vi "DetectorTest_MainV3.vi"() -> ()   [LabVIEW 2012]
uses:
  <vilib>/Utility/file.llb/Read From Spreadsheet File (DBL).vi
  <vilib>/Analysis/NI_AALBase.lvlib
panel:
  in  "TL4000 In":refnum<visa-resource-name> caption="resource name"
  out "Laser Counter":i32
  out "TL4000 Out":refnum<visa-resource-name> caption="instrument handle out"
  out "Calibration":cluster{"Y":dbl[], "Y":dbl[]}[](graph)
  out "Output Power (mW)":dbl
  in  "Load Calibration File":path
  out "Counter":i32
  out "NameList":string[](array[string])=["Diode_Open_3000", "Diode_Open_2000", "Diode_Open_1000", "Diode_Open_500", "Diode_Open_300", "Diode_Open_200", "Diode_Open_100", "Diode_Open_70", "Diode_Open_50", "Diode_Open_20", "Diode_Open_5_500", "Diode_Open_5_300", "Diode_Open_5_200", "Diode_Open_5_100", "Diode_Open_5_70", "Diode_Open_5_50", "Diode_Open_5_20", "Diode_Full_500", "Diode_Full_300", "Diode_Full_200", "Diode_Full_100", "Diode_Full_70", "Diode_Full_50", "Diode_Full_20", "Diode_Open_100_A", "Diode_Open_200_A", "QE_pad"]
  in  "Wafer Info Flash 2":T1={"Cell Name"="5500_130_05", "Package"="", "Coating"="", "LRC?"=enum."J2", "Comment"=""}
  in  "Parameters Flash 2":T2 {"Voc" format="%#_4g"; "Isc" format="%#_4g"; "FF" format="%#_4g"; "Imax" format="%#_4g"; "Vmax" format="%#_4g"; "Pmax" format="%#_4g"; "Itest" format="%#_4g"}
  in  "Wafer Info Flash":T1={"Cell Name"="Diode_Open_5_100", "Package"="", "Coating"="", "LRC?"=enum."J2", "Comment"=""}
  in  "Parameters Flash":T2={"Voc"=0.0, "Isc"=0.0, "FF"=0.0, "Vtest"=0.0, "Imax"=0.0, "Vmax"=0.0, "Pmax"=0.0, "Itest"=0.0, "Efficiency"=0.0, "Incident Power"=0.0, "Power Density (W/cm^2)"=0.0, "Cell Area (cm²)"=12801.99006, "Number of AM1.5D Suns"=0.0, "Input Current (mA)"=0.0, "Equivalent 1 sun Jsc"=0.0} {"Voc" format="%#_4g"; "Isc" format="%#_4g"; "FF" format="%#_4g"; "Imax" format="%#_4g"; "Vmax" format="%#_4g"; "Pmax" format="%#_4g"; "Itest" format="%#_4g"}
  out "RawData file":path=path "C:/Users/Flash/Desktop/Data/Detector test data/A-3348-2-A_Diode_Open_5_100_20171205171726.csv"
  out "Fine Cell Clusters":T3(array[cluster])=[{"Cell Name"="Diode_Open_5_100", "X-coord"=56060.0, "Y-coord"=24330.0, "Area"=12801.99006, "Grid Shadowing"=0.0, "Xdim"=50.0, "Ydim"=50.0, "Mesa Area"=7853.981634}, {"Cell Name"="Diode_Open_5_100", "X-coord"=56060.0, "Y-coord"=14330.0, "Area"=12801.99006, "Grid Shadowing"=0.0, "Xdim"=50.0, "Ydim"=50.0, "Mesa Area"=7853.981634}, {"Cell Name"="Diode_Open_5_100", "X-coord"=-3940.0, "Y-coord"=4330.0, "Area"=12801.99006, "Grid Shadowing"=0.0, "Xdim"=50.0, "Ydim"=50.0, "Mesa Area"=7853.981634}, {"Cell Name"="Diode_Open_5_100", "X-coord"=-9540.0, "Y-coord"=10700.0, "Area"=12801.99006, "Grid Shadowing"=0.0, "Xdim"=50.0, "Ydim"=50.0, "Mesa Area"=7853.981634}, {"Cell Name"="Diode_Open_5_100", "X-coord"=46060.0, "Y-coord"=4330.0, "Area"=12801.99006, "Grid Shadowing"=0.0, "Xdim"=50.0, "Ydim"=50.0, "Mesa Area"=7853.981634}, {"Cell Name"="Diode_Open_5_100", "X-coord"=6060.0, "Y-coord"=-5670.0, "Area"=12801.99006, "Grid Shadowing"=0.0, "Xdim"=50.0, "Ydim"=50.0, "Mesa Area"=7853.981634}, {"Cell Name"="Diode_Open_5_100", "X-coord"=460.0, "Y-coord"=700.0, "Area"=12801.99006, "Grid Shadowing"=0.0, "Xdim"=50.0, "Ydim"=50.0, "Mesa Area"=7853.981634}, {"Cell Name"="Diode_Open_5_100", "X-coord"=16060.0, "Y-coord"=-5670.0, "Area"=12801.99006, "Grid Shadowing"=0.0, "Xdim"=50.0, "Ydim"=50.0, "Mesa Area"=7853.981634}, {"Cell Name"="Diode_Open_5_100", "X-coord"=26060.0, "Y-coord"=-5670.0, "Area"=12801.99006, "Grid Shadowing"=0.0, "Xdim"=50.0, "Ydim"=50.0, "Mesa Area"=7853.981634}, {"Cell Name"="Diode_Open_5_100", "X-coord"=30460.0, "Y-coord"=700.0, "Area"=12801.99006, "Grid Shadowing"=0.0, "Xdim"=50.0, "Ydim"=50.0, "Mesa Area"=7853.981634}]
  out "Selected Data":cluster{dbl[], dbl[]}={[nan, nan, nan, nan, nan, nan, nan, nan, nan, nan, nan, nan, nan, nan, nan, nan, nan, nan, nan, nan, nan, nan, nan, nan, nan, nan, nan, nan, nan, nan, nan, nan, nan, nan, nan, nan, nan, nan, nan, nan, nan, nan, nan, nan, nan, nan, nan, nan, nan, nan, nan, nan, nan, nan, nan, nan, nan, nan, nan, nan, nan, nan, nan, nan, nan, nan, nan, nan, nan, nan, nan, nan, nan, nan, nan, nan, nan, nan, nan, nan, nan, nan, nan, nan, nan, nan, nan, nan, nan, nan, nan, nan, nan, nan, nan, nan, nan, nan, nan, nan, nan, nan, nan, nan], [nan, nan, nan, nan, nan, nan, nan, nan, nan, nan, nan, nan, nan, nan, nan, nan, nan, nan, nan, nan, nan, nan, nan, nan, nan, nan, nan, nan, nan, nan, nan, nan, nan, nan, nan, nan, nan, nan, nan, nan, nan, nan, nan, nan, nan, nan, nan, nan, nan, nan, nan, nan, nan, nan, nan, nan, nan, nan, nan, nan, nan, nan, nan, nan, nan, nan, nan, nan, nan, nan, nan, nan, nan, nan, nan, nan, nan, nan, nan, nan, nan, nan, nan, nan, nan, nan, nan, nan, nan, nan, nan, nan, nan, nan, nan, nan, nan, nan, nan, nan, nan, nan, nan, nan]}
  in  "Test Results 2":T4
  in  "Session Info 2":T5={"V set"=-1.0, "I compliance"=0.001, "J set"=0.01, "I set"=0.0, "V compliance"=1.0, "Laser Power (mW)"=0.0, "TestID"=0, "Session Time"=timestamp(0 s since 1904-01-01), "Operator"="Radek"} {"V compliance" format="%#_6f"; "I compliance" format="%#_6e"}
  in  "Die Info 2":T6={"Device Name"="", "ActiveArea_um2"=3848.451, "MesaArea_um2"=3848.451, "x"=0.0, "y"=0.0}
  in  "Wafer Info 2":T7
  in  "Test Results":T4={"I meas"=-8.21153e-09, "V meas"=0.229564, "Time"=timestamp(3595368212.7604895 s since 1904-01-01)}
  in  "Session Info":T5={"V set"=-1.0, "I compliance"=0.001, "J set"=0.01, "I set"=1.5393804e-06, "V compliance"=1.0, "Laser Power (mW)"=0.0, "TestID"=289, "Session Time"=timestamp(3595367846.336531 s since 1904-01-01), "Operator"="pkawula"} {"V compliance" format="%#_6f"; "I compliance" format="%#_6e"}
  in  "Die Info":T6={"Device Name"="Diode_Open_5_100", "ActiveArea_um2"=12801.99006, "MesaArea_um2"=7853.981634, "x"=6060.0, "y"=44330.0}
  in  "Wafer Info":T7={"Wafer Name"="A-3348-2-A", "Scribe"="BG531-103", "Mask"="SL066", "Lot"="SJC_ENG_342_4"}
  in  "Name Array":string[](array[string])=["Wafer name", "Scribe", "Mask", "Lot", "Device name", "Active Area", "Mesa Area", "x", "y", "Imeas", "Vmeas", "Time", "Vset", "Icomp", "Jset", "Iset", "Vcomp", "Laser Power", "TestID", "SessionTime", "Operator", "Selected"]
  in  "TestID file":path=path "C:/Users/Flash/Desktop/LabVIEW/Detector IV/rawtest_log.csv"
  in  "update wafer":bool
  in  "Lot":string="SJC_ENG_342_4"
  in  "Laser Current (mA)":dbl
  in  "Device Name":string="Diode_Open_5_100"
  in  "Scribe":string="BG531-105"
  in  "MesaArea_um2":dbl=7853.981634
  out "Status":string="idle"
  out "error out":errorcluster
  in  "error in (no error)":errorcluster
  out "Manaul Plot 1":cluster{"V manual":dbl[], dbl[]}[](array[cluster])=[{"V manual"=[-1.5, -1.45128, -1.40256, -1.35385, -1.30513, -1.25641, -1.20769, -1.15897, -1.11026, -1.06154, -1.01282, -0.964103, -0.915385, -0.866667, -0.817949, -0.769231, -0.720513, -0.671795, -0.623077, -0.574359, -0.525641, -0.476923, -0.428205, -0.379487, -0.330769, -0.282051, -0.233333, -0.184615, -0.135897, -0.0871795, -0.0384615, 0.0102564, 0.0589744, 0.107692, 0.15641, 0.205128, 0.253846, 0.302564, 0.351282, 0.4], [0.000371182, 0.000368087, 0.000365666, 0.000361585, 0.000358777, 0.000355415, 0.000352273, 0.00034839, 0.000345122, 0.00034151, 0.00033751, 0.000332836, 0.000329855, 0.000326461, 0.000322528, 0.000317656, 0.000313266, 0.000310053, 0.000304697, 0.000300113, 0.00029575, 0.000290713, 0.000285749, 0.00028048, 0.000275303, 0.000269023, 0.000263057, 0.000256756, 0.000250067, 0.000242646, 0.000235352, 0.000226249, 0.000216807, 0.000205541, 0.000192231, 0.000174354, 0.000146988, 9.49448e-05, 1.32493e-05, 0.000227531]}, {"V manual"=[-1.0, nan, nan, nan, nan, nan, nan, nan, nan, nan, nan, nan, nan, nan, nan, nan, nan, nan, nan, nan, nan, nan, nan, nan, nan, nan, nan, nan, nan, nan, nan, nan, nan, nan, nan, nan, nan, nan, nan, nan], [0.0003364616, nan, nan, nan, nan, nan, nan, nan, nan, nan, nan, nan, nan, nan, nan, nan, nan, nan, nan, nan, nan, nan, nan, nan, nan, nan, nan, nan, nan, nan, nan, nan, nan, nan, nan, nan, nan, nan, nan, nan]}, {"V manual"=[0.369974, nan, nan, nan, nan, nan, nan, nan, nan, nan, nan, nan, nan, nan, nan, nan, nan, nan, nan, nan, nan, nan, nan, nan, nan, nan, nan, nan, nan, nan, nan, nan, nan, nan, nan, nan, nan, nan, nan, nan], [8.183848863e-05, nan, nan, nan, nan, nan, nan, nan, nan, nan, nan, nan, nan, nan, nan, nan, nan, nan, nan, nan, nan, nan, nan, nan, nan, nan, nan, nan, nan, nan, nan, nan, nan, nan, nan, nan, nan, nan, nan, nan]}]
  out "Manual Plot 0":cluster{"V manual":dbl[], "I manual":dbl[]}[](array[cluster])=[{"V manual"=[-1.5, -1.45128, -1.40256, -1.35385, -1.30513, -1.25641, -1.20769, -1.15897, -1.11026, -1.06154, -1.01282, -0.964103, -0.915385, -0.866667, -0.817949, -0.769231, -0.720513, -0.671795, -0.623077, -0.574359, -0.525641, -0.476923, -0.428205, -0.379487, -0.330769, -0.282051, -0.233333, -0.184615, -0.135897, -0.0871795, -0.0384615, 0.0102564, 0.0589744, 0.107692, 0.15641, 0.205128, 0.253846, 0.302564, 0.351282, 0.4], "I manual"=[-0.000371182, -0.000368087, -0.000365666, -0.000361585, -0.000358777, -0.000355415, -0.000352273, -0.00034839, -0.000345122, -0.00034151, -0.00033751, -0.000332836, -0.000329855, -0.000326461, -0.000322528, -0.000317656, -0.000313266, -0.000310053, -0.000304697, -0.000300113, -0.00029575, -0.000290713, -0.000285749, -0.00028048, -0.000275303, -0.000269023, -0.000263057, -0.000256756, -0.000250067, -0.000242646, -0.000235352, -0.000226249, -0.000216807, -0.000205541, -0.000192231, -0.000174354, -0.000146988, -9.49448e-05, 1.32493e-05, 0.000227531]}, {"V manual"=[-1.0, nan, nan, nan, nan, nan, nan, nan, nan, nan, nan, nan, nan, nan, nan, nan, nan, nan, nan, nan, nan, nan, nan, nan, nan, nan, nan, nan, nan, nan, nan, nan, nan, nan, nan, nan, nan, nan, nan, nan], "I manual"=[-0.0003364616, nan, nan, nan, nan, nan, nan, nan, nan, nan, nan, nan, nan, nan, nan, nan, nan, nan, nan, nan, nan, nan, nan, nan, nan, nan, nan, nan, nan, nan, nan, nan, nan, nan, nan, nan, nan, nan, nan, nan]}, {"V manual"=[0.369974, nan, nan, nan, nan, nan, nan, nan, nan, nan, nan, nan, nan, nan, nan, nan, nan, nan, nan, nan, nan, nan, nan, nan, nan, nan, nan, nan, nan, nan, nan, nan, nan, nan, nan, nan, nan, nan, nan, nan], "I manual"=[8.183848863e-05, nan, nan, nan, nan, nan, nan, nan, nan, nan, nan, nan, nan, nan, nan, nan, nan, nan, nan, nan, nan, nan, nan, nan, nan, nan, nan, nan, nan, nan, nan, nan, nan, nan, nan, nan, nan, nan, nan, nan]}]
  in  "Reset 1st die":bool
  in  "Sweep Settings":T8={"Channel"=enum."Channel A", "Vstart"=-2.0, "Vend"=0.5, "# of points"=30, "NPLC"=1.0, "I compliance"=0.001, "Delay ms"=500.0}
  in  "Reset xy":bool
  out "current y":i32
  out "current x":i32
  in  "sweep delay ms":dbl=500.0
  in  "I compliance":dbl=0.001
  in  "points":u16=40
  in  "V end":dbl=0.4
  in  "V start":dbl=-1.5
  in  "Repeat Vf":u32=1
  out "I set":dbl=7.853981633999999e-07
  in  "V compliance":dbl=1.0 format="%#_6f"
  in  "Vf delay ms":dbl=100.0
  in  "J set A/cm2":dbl=0.01
  in  "Repeat Id":u32=5
  in  "I compliance":dbl=0.001 format="%#_6e"
  in  "Id delay ms":dbl=500.0
  in  "V set":dbl=-1.0
  out "Vmeas Settings":T9={"Channel"=enum."Channel A", "Iset"=-1.0, "NPLC"=1.0, "V compliance"=0.001, "Repeat time"=3, "Delay ms"=500.0}
  out "Imeas Settings":T10={"Channel"=enum."Channel A", "Vset"=-1.0, "NPLC"=1.0, "I compliance"=0.001, "Repeat time"=3, "Delay ms"=500.0}
  out "Array of Cell Data Clusters":T11(array[cluster])=[{"Cell Name"="Diode_Open_5_100", "X-coord"=-13940.0, "Y-coord"=24330.0, "Area"=12801.99006, "Grid Shadowing"=0.0, "Ydim"=50.0, "Xdim"=50.0, "Meas Area"=7853.981634}, {"Cell Name"="Diode_Open_5_100", "X-coord"=-19540.0, "Y-coord"=30700.0, "Area"=12801.99006, "Grid Shadowing"=0.0, "Ydim"=50.0, "Xdim"=50.0, "Meas Area"=7853.981634}, {"Cell Name"="Diode_Open_5_100", "X-coord"=-3940.0, "Y-coord"=24330.0, "Area"=12801.99006, "Grid Shadowing"=0.0, "Ydim"=50.0, "Xdim"=50.0, "Meas Area"=7853.981634}, {"Cell Name"="Diode_Open_5_100", "X-coord"=-9540.0, "Y-coord"=30700.0, "Area"=12801.99006, "Grid Shadowing"=0.0, "Ydim"=50.0, "Xdim"=50.0, "Meas Area"=7853.981634}, {"Cell Name"="Diode_Open_5_100", "X-coord"=6060.0, "Y-coord"=24330.0, "Area"=12801.99006, "Grid Shadowing"=0.0, "Ydim"=50.0, "Xdim"=50.0, "Meas Area"=7853.981634}, {"Cell Name"="Diode_Open_5_100", "X-coord"=460.0, "Y-coord"=30700.0, "Area"=12801.99006, "Grid Shadowing"=0.0, "Ydim"=50.0, "Xdim"=50.0, "Meas Area"=7853.981634}, {"Cell Name"="Diode_Open_5_100", "X-coord"=16060.0, "Y-coord"=24330.0, "Area"=12801.99006, "Grid Shadowing"=0.0, "Ydim"=50.0, "Xdim"=50.0, "Meas Area"=7853.981634}, {"Cell Name"="Diode_Open_5_100", "X-coord"=10460.0, "Y-coord"=30700.0, "Area"=12801.99006, "Grid Shadowing"=0.0, "Ydim"=50.0, "Xdim"=50.0, "Meas Area"=7853.981634}, {"Cell Name"="Diode_Open_5_100", "X-coord"=26060.0, "Y-coord"=24330.0, "Area"=12801.99006, "Grid Shadowing"=0.0, "Ydim"=50.0, "Xdim"=50.0, "Meas Area"=7853.981634}, {"Cell Name"="Diode_Open_5_100", "X-coord"=20460.0, "Y-coord"=30700.0, "Area"=12801.99006, "Grid Shadowing"=0.0, "Ydim"=50.0, "Xdim"=50.0, "Meas Area"=7853.981634}, {"Cell Name"="Diode_Open_5_100", "X-coord"=36060.0, "Y-coord"=24330.0, "Area"=12801.99006, "Grid Shadowing"=0.0, "Ydim"=50.0, "Xdim"=50.0, "Meas Area"=7853.981634}, {"Cell Name"="Diode_Open_5_100", "X-coord"=30460.0, "Y-coord"=30700.0, "Area"=12801.99006, "Grid Shadowing"=0.0, "Ydim"=50.0, "Xdim"=50.0, "Meas Area"=7853.981634}, {"Cell Name"="Diode_Open_5_100", "X-coord"=46060.0, "Y-coord"=24330.0, "Area"=12801.99006, "Grid Shadowing"=0.0, "Ydim"=50.0, "Xdim"=50.0, "Meas Area"=7853.981634}, {"Cell Name"="Diode_Open_5_100", "X-coord"=40460.0, "Y-coord"=30700.0, "Area"=12801.99006, "Grid Shadowing"=0.0, "Ydim"=50.0, "Xdim"=50.0, "Meas Area"=7853.981634}, {"Cell Name"="Diode_Open_5_100", "X-coord"=56060.0, "Y-coord"=24330.0, "Area"=12801.99006, "Grid Shadowing"=0.0, "Ydim"=50.0, "Xdim"=50.0, "Meas Area"=7853.981634}, {"Cell Name"="Diode_Open_5_100", "X-coord"=50460.0, "Y-coord"=30700.0, "Area"=12801.99006, "Grid Shadowing"=0.0, "Ydim"=50.0, "Xdim"=50.0, "Meas Area"=7853.981634}, {"Cell Name"="Diode_Open_5_100", "X-coord"=-13940.0, "Y-coord"=14330.0, "Area"=12801.99006, "Grid Shadowing"=0.0, "Ydim"=50.0, "Xdim"=50.0, "Meas Area"=7853.981634}, {"Cell Name"="Diode_Open_5_100", "X-coord"=-19540.0, "Y-coord"=20700.0, "Area"=12801.99006, "Grid Shadowing"=0.0, "Ydim"=50.0, "Xdim"=50.0, "Meas Area"=7853.981634}, {"Cell Name"="Diode_Open_5_100", "X-coord"=-3940.0, "Y-coord"=14330.0, "Area"=12801.99006, "Grid Shadowing"=0.0, "Ydim"=50.0, "Xdim"=50.0, "Meas Area"=7853.981634}, {"Cell Name"="Diode_Open_5_100", "X-coord"=-9540.0, "Y-coord"=20700.0, "Area"=12801.99006, "Grid Shadowing"=0.0, "Ydim"=50.0, "Xdim"=50.0, "Meas Area"=7853.981634}, {"Cell Name"="Diode_Open_5_100", "X-coord"=16060.0, "Y-coord"=14330.0, "Area"=12801.99006, "Grid Shadowing"=0.0, "Ydim"=50.0, "Xdim"=50.0, "Meas Area"=7853.981634}, {"Cell Name"="Diode_Open_5_100", "X-coord"=10460.0, "Y-coord"=20700.0, "Area"=12801.99006, "Grid Shadowing"=0.0, "Ydim"=50.0, "Xdim"=50.0, "Meas Area"=7853.981634}, {"Cell Name"="Diode_Open_5_100", "X-coord"=26060.0, "Y-coord"=14330.0, "Area"=12801.99006, "Grid Shadowing"=0.0, "Ydim"=50.0, "Xdim"=50.0, "Meas Area"=7853.981634}, {"Cell Name"="Diode_Open_5_100", "X-coord"=20460.0, "Y-coord"=20700.0, "Area"=12801.99006, "Grid Shadowing"=0.0, "Ydim"=50.0, "Xdim"=50.0, "Meas Area"=7853.981634}, {"Cell Name"="Diode_Open_5_100", "X-coord"=46060.0, "Y-coord"=14330.0, "Area"=12801.99006, "Grid Shadowing"=0.0, "Ydim"=50.0, "Xdim"=50.0, "Meas Area"=7853.981634}, {"Cell Name"="Diode_Open_5_100", "X-coord"=40460.0, "Y-coord"=20700.0, "Area"=12801.99006, "Grid Shadowing"=0.0, "Ydim"=50.0, "Xdim"=50.0, "Meas Area"=7853.981634}, {"Cell Name"="Diode_Open_5_100", "X-coord"=56060.0, "Y-coord"=14330.0, "Area"=12801.99006, "Grid Shadowing"=0.0, "Ydim"=50.0, "Xdim"=50.0, "Meas Area"=7853.981634}, {"Cell Name"="Diode_Open_5_100", "X-coord"=50460.0, "Y-coord"=20700.0, "Area"=12801.99006, "Grid Shadowing"=0.0, "Ydim"=50.0, "Xdim"=50.0, "Meas Area"=7853.981634}, {"Cell Name"="Diode_Open_5_100", "X-coord"=-3940.0, "Y-coord"=4330.0, "Area"=12801.99006, "Grid Shadowing"=0.0, "Ydim"=50.0, "Xdim"=50.0, "Meas Area"=7853.981634}, {"Cell Name"="Diode_Open_5_100", "X-coord"=-9540.0, "Y-coord"=10700.0, "Area"=12801.99006, "Grid Shadowing"=0.0, "Ydim"=50.0, "Xdim"=50.0, "Meas Area"=7853.981634}, {"Cell Name"="Diode_Open_5_100", "X-coord"=6060.0, "Y-coord"=4330.0, "Area"=12801.99006, "Grid Shadowing"=0.0, "Ydim"=50.0, "Xdim"=50.0, "Meas Area"=7853.981634}, {"Cell Name"="Diode_Open_5_100", "X-coord"=460.0, "Y-coord"=10700.0, "Area"=12801.99006, "Grid Shadowing"=0.0, "Ydim"=50.0, "Xdim"=50.0, "Meas Area"=7853.981634}, {"Cell Name"="Diode_Open_5_100", "X-coord"=16060.0, "Y-coord"=4330.0, "Area"=12801.99006, "Grid Shadowing"=0.0, "Ydim"=50.0, "Xdim"=50.0, "Meas Area"=7853.981634}, {"Cell Name"="Diode_Open_5_100", "X-coord"=10460.0, "Y-coord"=10700.0, "Area"=12801.99006, "Grid Shadowing"=0.0, "Ydim"=50.0, "Xdim"=50.0, "Meas Area"=7853.981634}, {"Cell Name"="Diode_Open_5_100", "X-coord"=26060.0, "Y-coord"=4330.0, "Area"=12801.99006, "Grid Shadowing"=0.0, "Ydim"=50.0, "Xdim"=50.0, "Meas Area"=7853.981634}, {"Cell Name"="Diode_Open_5_100", "X-coord"=20460.0, "Y-coord"=10700.0, "Area"=12801.99006, "Grid Shadowing"=0.0, "Ydim"=50.0, "Xdim"=50.0, "Meas Area"=7853.981634}, {"Cell Name"="Diode_Open_5_100", "X-coord"=36060.0, "Y-coord"=4330.0, "Area"=12801.99006, "Grid Shadowing"=0.0, "Ydim"=50.0, "Xdim"=50.0, "Meas Area"=7853.981634}, {"Cell Name"="Diode_Open_5_100", "X-coord"=30460.0, "Y-coord"=10700.0, "Area"=12801.99006, "Grid Shadowing"=0.0, "Ydim"=50.0, "Xdim"=50.0, "Meas Area"=7853.981634}, {"Cell Name"="Diode_Open_5_100", "X-coord"=46060.0, "Y-coord"=4330.0, "Area"=12801.99006, "Grid Shadowing"=0.0, "Ydim"=50.0, "Xdim"=50.0, "Meas Area"=7853.981634}, {"Cell Name"="Diode_Open_5_100", "X-coord"=40460.0, "Y-coord"=10700.0, "Area"=12801.99006, "Grid Shadowing"=0.0, "Ydim"=50.0, "Xdim"=50.0, "Meas Area"=7853.981634}, {"Cell Name"="Diode_Open_5_100", "X-coord"=6060.0, "Y-coord"=-5670.0, "Area"=12801.99006, "Grid Shadowing"=0.0, "Ydim"=50.0, "Xdim"=50.0, "Meas Area"=7853.981634}, {"Cell Name"="Diode_Open_5_100", "X-coord"=460.0, "Y-coord"=700.0, "Area"=12801.99006, "Grid Shadowing"=0.0, "Ydim"=50.0, "Xdim"=50.0, "Meas Area"=7853.981634}, {"Cell Name"="Diode_Open_5_100", "X-coord"=16060.0, "Y-coord"=-5670.0, "Area"=12801.99006, "Grid Shadowing"=0.0, "Ydim"=50.0, "Xdim"=50.0, "Meas Area"=7853.981634}, {"Cell Name"="Diode_Open_5_100", "X-coord"=10460.0, "Y-coord"=700.0, "Area"=12801.99006, "Grid Shadowing"=0.0, "Ydim"=50.0, "Xdim"=50.0, "Meas Area"=7853.981634}, {"Cell Name"="Diode_Open_5_100", "X-coord"=26060.0, "Y-coord"=-5670.0, "Area"=12801.99006, "Grid Shadowing"=0.0, "Ydim"=50.0, "Xdim"=50.0, "Meas Area"=7853.981634}, {"Cell Name"="Diode_Open_5_100", "X-coord"=20460.0, "Y-coord"=700.0, "Area"=12801.99006, "Grid Shadowing"=0.0, "Ydim"=50.0, "Xdim"=50.0, "Meas Area"=7853.981634}, {"Cell Name"="Diode_Open_5_100", "X-coord"=36060.0, "Y-coord"=-5670.0, "Area"=12801.99006, "Grid Shadowing"=0.0, "Ydim"=50.0, "Xdim"=50.0, "Meas Area"=7853.981634}, {"Cell Name"="Diode_Open_5_100", "X-coord"=30460.0, "Y-coord"=700.0, "Area"=12801.99006, "Grid Shadowing"=0.0, "Ydim"=50.0, "Xdim"=50.0, "Meas Area"=7853.981634}, {"Cell Name"="Diode_Open_5_100", "X-coord"=6060.0, "Y-coord"=54330.0, "Area"=12801.99006, "Grid Shadowing"=0.0, "Ydim"=50.0, "Xdim"=50.0, "Meas Area"=7853.981634}, {"Cell Name"="Diode_Open_5_100", "X-coord"=460.0, "Y-coord"=60700.0, "Area"=12801.99006, "Grid Shadowing"=0.0, "Ydim"=50.0, "Xdim"=50.0, "Meas Area"=7853.981634}, {"Cell Name"="Diode_Open_5_100", "X-coord"=6060.0, "Y-coord"=64330.0, "Area"=12801.99006, "Grid Shadowing"=0.0, "Ydim"=50.0, "Xdim"=50.0, "Meas Area"=7853.981634}, {"Cell Name"="Diode_Open_5_100", "X-coord"=460.0, "Y-coord"=70700.0, "Area"=12801.99006, "Grid Shadowing"=0.0, "Ydim"=50.0, "Xdim"=50.0, "Meas Area"=7853.981634}, {"Cell Name"="Diode_Open_5_100", "X-coord"=16060.0, "Y-coord"=64330.0, "Area"=12801.99006, "Grid Shadowing"=0.0, "Ydim"=50.0, "Xdim"=50.0, "Meas Area"=7853.981634}, {"Cell Name"="Diode_Open_5_100", "X-coord"=10460.0, "Y-coord"=70700.0, "Area"=12801.99006, "Grid Shadowing"=0.0, "Ydim"=50.0, "Xdim"=50.0, "Meas Area"=7853.981634}, {"Cell Name"="Diode_Open_5_100", "X-coord"=26060.0, "Y-coord"=64330.0, "Area"=12801.99006, "Grid Shadowing"=0.0, "Ydim"=50.0, "Xdim"=50.0, "Meas Area"=7853.981634}, {"Cell Name"="Diode_Open_5_100", "X-coord"=20460.0, "Y-coord"=70700.0, "Area"=12801.99006, "Grid Shadowing"=0.0, "Ydim"=50.0, "Xdim"=50.0, "Meas Area"=7853.981634}, {"Cell Name"="Diode_Open_5_100", "X-coord"=36060.0, "Y-coord"=64330.0, "Area"=12801.99006, "Grid Shadowing"=0.0, "Ydim"=50.0, "Xdim"=50.0, "Meas Area"=7853.981634}, {"Cell Name"="Diode_Open_5_100", "X-coord"=30460.0, "Y-coord"=70700.0, "Area"=12801.99006, "Grid Shadowing"=0.0, "Ydim"=50.0, "Xdim"=50.0, "Meas Area"=7853.981634}, {"Cell Name"="Diode_Open_5_100", "X-coord"=-3940.0, "Y-coord"=54330.0, "Area"=12801.99006, "Grid Shadowing"=0.0, "Ydim"=50.0, "Xdim"=50.0, "Meas Area"=7853.981634}, {"Cell Name"="Diode_Open_5_100", "X-coord"=-9540.0, "Y-coord"=60700.0, "Area"=12801.99006, "Grid Shadowing"=0.0, "Ydim"=50.0, "Xdim"=50.0, "Meas Area"=7853.981634}, {"Cell Name"="Diode_Open_5_100", "X-coord"=16060.0, "Y-coord"=54330.0, "Area"=12801.99006, "Grid Shadowing"=0.0, "Ydim"=50.0, "Xdim"=50.0, "Meas Area"=7853.981634}, {"Cell Name"="Diode_Open_5_100", "X-coord"=10460.0, "Y-coord"=60700.0, "Area"=12801.99006, "Grid Shadowing"=0.0, "Ydim"=50.0, "Xdim"=50.0, "Meas Area"=7853.981634}, {"Cell Name"="Diode_Open_5_100", "X-coord"=26060.0, "Y-coord"=54330.0, "Area"=12801.99006, "Grid Shadowing"=0.0, "Ydim"=50.0, "Xdim"=50.0, "Meas Area"=7853.981634}, {"Cell Name"="Diode_Open_5_100", "X-coord"=20460.0, "Y-coord"=60700.0, "Area"=12801.99006, "Grid Shadowing"=0.0, "Ydim"=50.0, "Xdim"=50.0, "Meas Area"=7853.981634}, {"Cell Name"="Diode_Open_5_100", "X-coord"=36060.0, "Y-coord"=54330.0, "Area"=12801.99006, "Grid Shadowing"=0.0, "Ydim"=50.0, "Xdim"=50.0, "Meas Area"=7853.981634}, {"Cell Name"="Diode_Open_5_100", "X-coord"=30460.0, "Y-coord"=60700.0, "Area"=12801.99006, "Grid Shadowing"=0.0, "Ydim"=50.0, "Xdim"=50.0, "Meas Area"=7853.981634}, {"Cell Name"="Diode_Open_5_100", "X-coord"=46060.0, "Y-coord"=54330.0, "Area"=12801.99006, "Grid Shadowing"=0.0, "Ydim"=50.0, "Xdim"=50.0, "Meas Area"=7853.981634}, {"Cell Name"="Diode_Open_5_100", "X-coord"=40460.0, "Y-coord"=60700.0, "Area"=12801.99006, "Grid Shadowing"=0.0, "Ydim"=50.0, "Xdim"=50.0, "Meas Area"=7853.981634}, {"Cell Name"="Diode_Open_5_100", "X-coord"=-13940.0, "Y-coord"=44330.0, "Area"=12801.99006, "Grid Shadowing"=0.0, "Ydim"=50.0, "Xdim"=50.0, "Meas Area"=7853.981634}, {"Cell Name"="Diode_Open_5_100", "X-coord"=-19540.0, "Y-coord"=50700.0, "Area"=12801.99006, "Grid Shadowing"=0.0, "Ydim"=50.0, "Xdim"=50.0, "Meas Area"=7853.981634}, {"Cell Name"="Diode_Open_5_100", "X-coord"=-3940.0, "Y-coord"=44330.0, "Area"=12801.99006, "Grid Shadowing"=0.0, "Ydim"=50.0, "Xdim"=50.0, "Meas Area"=7853.981634}, {"Cell Name"="Diode_Open_5_100", "X-coord"=-9540.0, "Y-coord"=50700.0, "Area"=12801.99006, "Grid Shadowing"=0.0, "Ydim"=50.0, "Xdim"=50.0, "Meas Area"=7853.981634}, {"Cell Name"="Diode_Open_5_100", "X-coord"=56060.0, "Y-coord"=34330.0, "Area"=12801.99006, "Grid Shadowing"=0.0, "Ydim"=50.0, "Xdim"=50.0, "Meas Area"=7853.981634}, {"Cell Name"="Diode_Open_5_100", "X-coord"=50460.0, "Y-coord"=40700.0, "Area"=12801.99006, "Grid Shadowing"=0.0, "Ydim"=50.0, "Xdim"=50.0, "Meas Area"=7853.981634}, {"Cell Name"="Diode_Open_5_100", "X-coord"=46060.0, "Y-coord"=34330.0, "Area"=12801.99006, "Grid Shadowing"=0.0, "Ydim"=50.0, "Xdim"=50.0, "Meas Area"=7853.981634}, {"Cell Name"="Diode_Open_5_100", "X-coord"=40460.0, "Y-coord"=40700.0, "Area"=12801.99006, "Grid Shadowing"=0.0, "Ydim"=50.0, "Xdim"=50.0, "Meas Area"=7853.981634}, {"Cell Name"="Diode_Open_5_100", "X-coord"=36060.0, "Y-coord"=34330.0, "Area"=12801.99006, "Grid Shadowing"=0.0, "Ydim"=50.0, "Xdim"=50.0, "Meas Area"=7853.981634}, {"Cell Name"="Diode_Open_5_100", "X-coord"=30460.0, "Y-coord"=40700.0, "Area"=12801.99006, "Grid Shadowing"=0.0, "Ydim"=50.0, "Xdim"=50.0, "Meas Area"=7853.981634}, {"Cell Name"="Diode_Open_5_100", "X-coord"=26060.0, "Y-coord"=34330.0, "Area"=12801.99006, "Grid Shadowing"=0.0, "Ydim"=50.0, "Xdim"=50.0, "Meas Area"=7853.981634}, {"Cell Name"="Diode_Open_5_100", "X-coord"=20460.0, "Y-coord"=40700.0, "Area"=12801.99006, "Grid Shadowing"=0.0, "Ydim"=50.0, "Xdim"=50.0, "Meas Area"=7853.981634}, {"Cell Name"="Diode_Open_5_100", "X-coord"=16060.0, "Y-coord"=34330.0, "Area"=12801.99006, "Grid Shadowing"=0.0, "Ydim"=50.0, "Xdim"=50.0, "Meas Area"=7853.981634}, {"Cell Name"="Diode_Open_5_100", "X-coord"=10460.0, "Y-coord"=40700.0, "Area"=12801.99006, "Grid Shadowing"=0.0, "Ydim"=50.0, "Xdim"=50.0, "Meas Area"=7853.981634}, {"Cell Name"="Diode_Open_5_100", "X-coord"=6060.0, "Y-coord"=34330.0, "Area"=12801.99006, "Grid Shadowing"=0.0, "Ydim"=50.0, "Xdim"=50.0, "Meas Area"=7853.981634}, {"Cell Name"="Diode_Open_5_100", "X-coord"=460.0, "Y-coord"=40700.0, "Area"=12801.99006, "Grid Shadowing"=0.0, "Ydim"=50.0, "Xdim"=50.0, "Meas Area"=7853.981634}, {"Cell Name"="Diode_Open_5_100", "X-coord"=-3940.0, "Y-coord"=34330.0, "Area"=12801.99006, "Grid Shadowing"=0.0, "Ydim"=50.0, "Xdim"=50.0, "Meas Area"=7853.981634}, {"Cell Name"="Diode_Open_5_100", "X-coord"=-9540.0, "Y-coord"=40700.0, "Area"=12801.99006, "Grid Shadowing"=0.0, "Ydim"=50.0, "Xdim"=50.0, "Meas Area"=7853.981634}, {"Cell Name"="Diode_Open_5_100", "X-coord"=-13940.0, "Y-coord"=34330.0, "Area"=12801.99006, "Grid Shadowing"=0.0, "Ydim"=50.0, "Xdim"=50.0, "Meas Area"=7853.981634}, {"Cell Name"="Diode_Open_5_100", "X-coord"=-19540.0, "Y-coord"=40700.0, "Area"=12801.99006, "Grid Shadowing"=0.0, "Ydim"=50.0, "Xdim"=50.0, "Meas Area"=7853.981634}, {"Cell Name"="Diode_Open_5_100", "X-coord"=56060.0, "Y-coord"=44330.0, "Area"=12801.99006, "Grid Shadowing"=0.0, "Ydim"=50.0, "Xdim"=50.0, "Meas Area"=7853.981634}, {"Cell Name"="Diode_Open_5_100", "X-coord"=50460.0, "Y-coord"=50700.0, "Area"=12801.99006, "Grid Shadowing"=0.0, "Ydim"=50.0, "Xdim"=50.0, "Meas Area"=7853.981634}, {"Cell Name"="Diode_Open_5_100", "X-coord"=46060.0, "Y-coord"=44330.0, "Area"=12801.99006, "Grid Shadowing"=0.0, "Ydim"=50.0, "Xdim"=50.0, "Meas Area"=7853.981634}, {"Cell Name"="Diode_Open_5_100", "X-coord"=40460.0, "Y-coord"=50700.0, "Area"=12801.99006, "Grid Shadowing"=0.0, "Ydim"=50.0, "Xdim"=50.0, "Meas Area"=7853.981634}, {"Cell Name"="Diode_Open_5_100", "X-coord"=26060.0, "Y-coord"=44330.0, "Area"=12801.99006, "Grid Shadowing"=0.0, "Ydim"=50.0, "Xdim"=50.0, "Meas Area"=7853.981634}, {"Cell Name"="Diode_Open_5_100", "X-coord"=20460.0, "Y-coord"=50700.0, "Area"=12801.99006, "Grid Shadowing"=0.0, "Ydim"=50.0, "Xdim"=50.0, "Meas Area"=7853.981634}, {"Cell Name"="Diode_Open_5_100", "X-coord"=16060.0, "Y-coord"=44330.0, "Area"=12801.99006, "Grid Shadowing"=0.0, "Ydim"=50.0, "Xdim"=50.0, "Meas Area"=7853.981634}, {"Cell Name"="Diode_Open_5_100", "X-coord"=10460.0, "Y-coord"=50700.0, "Area"=12801.99006, "Grid Shadowing"=0.0, "Ydim"=50.0, "Xdim"=50.0, "Meas Area"=7853.981634}, {"Cell Name"="Diode_Open_5_100", "X-coord"=30460.0, "Y-coord"=20700.0, "Area"=12801.99006, "Grid Shadowing"=0.0, "Ydim"=50.0, "Xdim"=50.0, "Meas Area"=7853.981634}, {"Cell Name"="Diode_Open_5_100", "X-coord"=36060.0, "Y-coord"=14330.0, "Area"=12801.99006, "Grid Shadowing"=0.0, "Ydim"=50.0, "Xdim"=50.0, "Meas Area"=7853.981634}, {"Cell Name"="Diode_Open_5_100", "X-coord"=460.0, "Y-coord"=20700.0, "Area"=12801.99006, "Grid Shadowing"=0.0, "Ydim"=50.0, "Xdim"=50.0, "Meas Area"=7853.981634}, {"Cell Name"="Diode_Open_5_100", "X-coord"=6060.0, "Y-coord"=14330.0, "Area"=12801.99006, "Grid Shadowing"=0.0, "Ydim"=50.0, "Xdim"=50.0, "Meas Area"=7853.981634}, {"Cell Name"="Diode_Open_5_100", "X-coord"=30460.0, "Y-coord"=50700.0, "Area"=12801.99006, "Grid Shadowing"=0.0, "Ydim"=50.0, "Xdim"=50.0, "Meas Area"=7853.981634}, {"Cell Name"="Diode_Open_5_100", "X-coord"=36060.0, "Y-coord"=44330.0, "Area"=12801.99006, "Grid Shadowing"=0.0, "Ydim"=50.0, "Xdim"=50.0, "Meas Area"=7853.981634}, {"Cell Name"="Diode_Open_5_100", "X-coord"=460.0, "Y-coord"=50700.0, "Area"=12801.99006, "Grid Shadowing"=0.0, "Ydim"=50.0, "Xdim"=50.0, "Meas Area"=7853.981634}, {"Cell Name"="Diode_Open_5_100", "X-coord"=6060.0, "Y-coord"=44330.0, "Area"=12801.99006, "Grid Shadowing"=0.0, "Ydim"=50.0, "Xdim"=50.0, "Meas Area"=7853.981634}]
  in  "stop":bool
  in  "ActiveArea_um2":dbl=12801.99006
  in  "NPLC":dbl=1.0
  in  "Operator":string(combo)="pkawula"
  in  "Mask":string="SL066"
  in  "Wafer Name":string="A-3348-3-A"
  in  "Tab Control":T12(tab)
  in  "Clear Laser List":bool
  in  "Remove from Laser List":bool
  in  "Add to Laser":bool
  in  "Desired Current (mA)":dbl
  in  "Laser List":i32(listbox)=-1
  in  "Start auto":bool
  in  "Clear List":bool
  in  "Refresh Device":bool
  in  "Mask Name":string="SL066"
  in  "Remove from List":bool
  in  "Add to list":bool
  in  "Available Device Name":string(combo)="Diode_Open_200_A"
  in  "Test List":i32(listbox)=-1
  in  "Mask File all":path=path "C:/Users/Flash/Desktop/Mask Files/SL066 Detector/SL066_mask_map_file_V3_align on D3000.csv"
  in  "Manual_Test":bool
  in  "Manual IV settting":enum32{"Linear plot", "Log plot"}(radio)
  out "Vmeas manual":dbl=0.369974
  out "Imeas manual":dbl=-0.0003364616
  out "Iarray manual":dbl[](array[numeric])=[-0.000371182, -0.000368087, -0.000365666, -0.000361585, -0.000358777, -0.000355415, -0.000352273, -0.00034839, -0.000345122, -0.00034151, -0.00033751, -0.000332836, -0.000329855, -0.000326461, -0.000322528, -0.000317656, -0.000313266, -0.000310053, -0.000304697, -0.000300113, -0.00029575, -0.000290713, -0.000285749, -0.00028048, -0.000275303, -0.000269023, -0.000263057, -0.000256756, -0.000250067, -0.000242646, -0.000235352, -0.000226249, -0.000216807, -0.000205541, -0.000192231, -0.000174354, -0.000146988, -9.49448e-05, 1.32493e-05, 0.000227531]
  out "Varray manual":dbl[](array[numeric])=[-1.5, -1.45128, -1.40256, -1.35385, -1.30513, -1.25641, -1.20769, -1.15897, -1.11026, -1.06154, -1.01282, -0.964103, -0.915385, -0.866667, -0.817949, -0.769231, -0.720513, -0.671795, -0.623077, -0.574359, -0.525641, -0.476923, -0.428205, -0.379487, -0.330769, -0.282051, -0.233333, -0.184615, -0.135897, -0.0871795, -0.0384615, 0.0102564, 0.0589744, 0.107692, 0.15641, 0.205128, 0.253846, 0.302564, 0.351282, 0.4]
  out "y target":i32=28070
  out "x target":i32=-15300
  in  "Die Number":u16(ring) items=["0", "1", "2", "3", "4", "5", "6", "7", "8", "9", "10", "11", "12", "13", "14", "15", "16", "17", "18", "19", "20", "21", "22", "23", "24", "25", "26", "27", "28", "29", "30", "31", "32", "33", "34", "35", "36", "37", "38", "39", "40", "41", "42", "43", "44", "45", "46", "47", "48", "49", "50", "51", "52", "53", "54", "55", "56", "57", "58", "59", "60", "61", "62", "63", "64", "65", "66", "67", "68", "69", "70", "71", "72", "73", "74", "75", "76", "77", "78", "79", "80", "81", "82", "83", "84", "85", "86", "87", "88", "89", "90", "91", "92", "93", "94", "95", "96", "97", "98", "99", "100", "101", "102", "103"]
  in  "load file":bool
  in  "Move to":bool
  in  "Mask File Manual":path=path "C:/Users/Flash/Desktop/Mask Files/SL066 Detector/SL066_mask_map_file_V3_align on D3000_Diode_Open_1000.csv"
  out "Manual IV":cluster{"V manual":dbl[], "I manual":dbl[]}[](graph)=[{"V manual"=[-1.5, -1.45128, -1.40256, -1.35385, -1.30513, -1.25641, -1.20769, -1.15897, -1.11026, -1.06154, -1.01282, -0.964103, -0.915385, -0.866667, -0.817949, -0.769231, -0.720513, -0.671795, -0.623077, -0.574359, -0.525641, -0.476923, -0.428205, -0.379487, -0.330769, -0.282051, -0.233333, -0.184615, -0.135897, -0.0871795, -0.0384615, 0.0102564, 0.0589744, 0.107692, 0.15641, 0.205128, 0.253846, 0.302564, 0.351282, 0.4], "I manual"=[-0.000371182, -0.000368087, -0.000365666, -0.000361585, -0.000358777, -0.000355415, -0.000352273, -0.00034839, -0.000345122, -0.00034151, -0.00033751, -0.000332836, -0.000329855, -0.000326461, -0.000322528, -0.000317656, -0.000313266, -0.000310053, -0.000304697, -0.000300113, -0.00029575, -0.000290713, -0.000285749, -0.00028048, -0.000275303, -0.000269023, -0.000263057, -0.000256756, -0.000250067, -0.000242646, -0.000235352, -0.000226249, -0.000216807, -0.000205541, -0.000192231, -0.000174354, -0.000146988, -9.49448e-05, 1.32493e-05, 0.000227531]}, {"V manual"=[-1.0, nan, nan, nan, nan, nan, nan, nan, nan, nan, nan, nan, nan, nan, nan, nan, nan, nan, nan, nan, nan, nan, nan, nan, nan, nan, nan, nan, nan, nan, nan, nan, nan, nan, nan, nan, nan, nan, nan, nan], "I manual"=[-0.0003364616, nan, nan, nan, nan, nan, nan, nan, nan, nan, nan, nan, nan, nan, nan, nan, nan, nan, nan, nan, nan, nan, nan, nan, nan, nan, nan, nan, nan, nan, nan, nan, nan, nan, nan, nan, nan, nan, nan, nan]}, {"V manual"=[0.369974, nan, nan, nan, nan, nan, nan, nan, nan, nan, nan, nan, nan, nan, nan, nan, nan, nan, nan, nan, nan, nan, nan, nan, nan, nan, nan, nan, nan, nan, nan, nan, nan, nan, nan, nan, nan, nan, nan, nan], "I manual"=[8.183848863e-05, nan, nan, nan, nan, nan, nan, nan, nan, nan, nan, nan, nan, nan, nan, nan, nan, nan, nan, nan, nan, nan, nan, nan, nan, nan, nan, nan, nan, nan, nan, nan, nan, nan, nan, nan, nan, nan, nan, nan]}]
  in  "Load raw":bool
  in  "Select":bool
  in  "Number Select":u16=10
  in  "Vmax":dbl=0.95
  in  "Vmin":dbl=0.05
  out "Test FileName":string="A-3348-2-A_Diode_Open_5_100_20171205171726.csv"
  out "RawTest ID":u32=289
  out "Progress":u8(slide)=99 scale=0.0..100.0
  out "Current Device":u32=104
  out "Total Device":u32=104
  out "V meas":dbl[](array[numeric])=[0.233008, 0.99988, 0.230081, 0.231856, 0.222896, 0.227718, 0.220368, 0.221624, 0.223083, 0.225844, 0.224788, 0.226016, 0.230367, 0.226863, 0.236152, 0.999885, 0.236278, 0.231894, 0.227969, 0.231092, 0.223719, 0.223157, 0.221075, 0.223088, 0.229423, 0.227845, 0.234104, 0.999884, 0.236984, 0.234402, 0.229175, 0.22777, 0.221645, 0.226168, 0.222958, 0.221157, 0.226097, 0.22608, 0.22911, 0.227312, 0.233594, 0.239497, 0.228026, 0.226055, 0.22758, 0.222034, 0.225611, 0.229698, 0.235983, 0.999873, 0.999878, 0.999876, 0.999884, 0.99988, 0.999881, 0.999878, 0.999876, 0.999876, 0.242386, 0.999877, 0.232405, 0.999877, 0.232378, 0.999881, 0.235204, 0.999878, 0.999878, 0.999878, 0.240209, 0.23837, 0.999879, 0.241394, 0.999882, 0.999877, 0.232764, 0.231476, 0.227194, 0.228614, 0.227446, 0.225845, 0.222835, 0.226481, 0.225718, 0.229356, 0.232511, 0.999874, 0.999878, 0.999879, 0.511839, 0.999881, 0.236876, 0.237455, 0.224476, 0.236416, 0.222221, 0.230631, 0.225214, 0.22589, 0.226556, 0.226418, 0.234927, 0.233388, 0.237265, 0.229564]
  out "I meas":dbl[](array[numeric])=[-1.791366e-08, -1.1957407999999998e-10, -8.510296e-09, -1.1848348e-08, -1.0634712e-08, -7.94538e-09, -1.0664641999999998e-08, -1.5484518e-08, -1.2807029999999998e-08, -1.2872500000000002e-08, -8.70304e-09, -1.0948554000000001e-08, -6.430202000000001e-09, -8.940911999999999e-09, -4.269804e-09, -2.3908200000000002e-09, -6.1184e-09, -7.475178e-09, -9.294318e-09, -1.0505516000000001e-08, -7.3206440000000005e-09, -8.520726e-09, -8.80908e-09, -1.0621755999999999e-08, -6.43336e-09, -8.429852e-09, -5.041916000000001e-09, -1.9718416e-10, -4.6682759999999995e-09, -5.138274e-09, -6.394414e-09, -7.840453999999999e-09, -8.213534e-09, -8.437916e-09, -8.39969e-09, -1.0195582e-08, -5.942146e-09, -7.641714e-09, -4.799278e-09, -6.2362860000000006e-09, -4.420012e-09, -3.2603080000000005e-09, -5.559286e-09, -5.7098779999999995e-09, -5.365526e-09, -7.813004e-09, -6.011059999999999e-09, -5.480968e-09, -1.035395e-08, 7.317542e-11, -6.2418100000000004e-12, 2.8383740000000004e-11, 3.794192e-11, 4.911428e-12, 2.923012e-11, 2.809286e-11, 3.036024e-11, -1.6028400000000002e-10, -9.937287999999999e-09, 4.2383680000000005e-11, -1.1358554000000001e-08, 3.9725299999999996e-11, -1.0078494000000001e-08, 6.30498e-11, -7.550982e-09, 8.784526e-11, -5.557216e-10, -9.84718e-11, -7.308986e-09, -1.3814348000000002e-08, 7.365464000000002e-11, -8.052186000000001e-09, -1.1067396e-11, -2.554022e-09, -7.325092e-09, -7.05232e-09, -9.755659999999999e-09, -1.1196856000000001e-08, -1.4346882000000001e-08, -1.4860736000000002e-08, -1.5036204e-08, -1.3369388e-08, -1.0021694e-08, -9.621842e-09, -8.068194e-09, 5.4979339999999994e-11, 5.7530419999999994e-12, -3.246182e-09, -4.980356000000001e-09, -2.7533859999999997e-09, -6.70936e-09, -6.9177280000000005e-09, -1.4554624e-08, -1.4164096000000001e-08, -1.6854384e-08, -1.380222e-08, -7.668758e-09, -5.926224e-09, -1.1557444000000001e-08, -7.354524000000001e-09, -8.160112000000001e-09, -9.152704000000001e-09, -1.1161659999999998e-08, -8.21153e-09]
  in  "RawData Save Path":path=path "C:/Users/Flash/Desktop/Data/Detector test data"
  in  "StartRaw":bool
  out "Vforward hist":T13(graph)={"X Values"=[0.25934385, 0.33729555, 0.41524725, 0.49319895, 0.57115065, 0.64910235, 0.72705405, 0.80500575, 0.88295745, 0.96090915], "Histogram: h(x)"=[78, 0, 0, 1, 0, 0, 0, 0, 0, 25]}
  out "Idark hist":T13(graph)={"X Values"=[-1.7013584737e-08, -1.5213434211e-08, -1.3413283685000001e-08, -1.1613133159000001e-08, -9.812982633000001e-09, -8.012832107e-09, -6.212681581000001e-09, -4.4125310550000005e-09, -2.6123805290000004e-09, -8.12230003e-10], "Histogram: h(x)"=[2, 5, 6, 6, 14, 23, 15, 7, 5, 21]}
  in  "Mask File Raw":path=path "C:/Users/Flash/Desktop/Mask Files/SL066 Detector/SL066_mask_map_file_V3_align on D3000_Diode_Open_5_100.csv"
  out "Spec Plot":cluster{"V meas":dbl[], "I meas":dbl[]}[](graph)=[{"V meas"=[0.233008, 0.99988, 0.230081, 0.231856, 0.222896, 0.227718, 0.220368, 0.221624, 0.223083, 0.225844, 0.224788, 0.226016, 0.230367, 0.226863, 0.236152, 0.999885, 0.236278, 0.231894, 0.227969, 0.231092, 0.223719, 0.223157, 0.221075, 0.223088, 0.229423, 0.227845, 0.234104, 0.999884, 0.236984, 0.234402, 0.229175, 0.22777, 0.221645, 0.226168, 0.222958, 0.221157, 0.226097, 0.22608, 0.22911, 0.227312, 0.233594, 0.239497, 0.228026, 0.226055, 0.22758, 0.222034, 0.225611, 0.229698, 0.235983, 0.999873, 0.999878, 0.999876, 0.999884, 0.99988, 0.999881, 0.999878, 0.999876, 0.999876, 0.242386, 0.999877, 0.232405, 0.999877, 0.232378, 0.999881, 0.235204, 0.999878, 0.999878, 0.999878, 0.240209, 0.23837, 0.999879, 0.241394, 0.999882, 0.999877, 0.232764, 0.231476, 0.227194, 0.228614, 0.227446, 0.225845, 0.222835, 0.226481, 0.225718, 0.229356, 0.232511, 0.999874, 0.999878, 0.999879, 0.511839, 0.999881, 0.236876, 0.237455, 0.224476, 0.236416, 0.222221, 0.230631, 0.225214, 0.22589, 0.226556, 0.226418, 0.234927, 0.233388, 0.237265, 0.229564], "I meas"=[-1.791366e-08, -1.1957407999999998e-10, -8.510296e-09, -1.1848348e-08, -1.0634712e-08, -7.94538e-09, -1.0664641999999998e-08, -1.5484518e-08, -1.2807029999999998e-08, -1.2872500000000002e-08, -8.70304e-09, -1.0948554000000001e-08, -6.430202000000001e-09, -8.940911999999999e-09, -4.269804e-09, -2.3908200000000002e-09, -6.1184e-09, -7.475178e-09, -9.294318e-09, -1.0505516000000001e-08, -7.3206440000000005e-09, -8.520726e-09, -8.80908e-09, -1.0621755999999999e-08, -6.43336e-09, -8.429852e-09, -5.041916000000001e-09, -1.9718416e-10, -4.6682759999999995e-09, -5.138274e-09, -6.394414e-09, -7.840453999999999e-09, -8.213534e-09, -8.437916e-09, -8.39969e-09, -1.0195582e-08, -5.942146e-09, -7.641714e-09, -4.799278e-09, -6.2362860000000006e-09, -4.420012e-09, -3.2603080000000005e-09, -5.559286e-09, -5.7098779999999995e-09, -5.365526e-09, -7.813004e-09, -6.011059999999999e-09, -5.480968e-09, -1.035395e-08, 7.317542e-11, -6.2418100000000004e-12, 2.8383740000000004e-11, 3.794192e-11, 4.911428e-12, 2.923012e-11, 2.809286e-11, 3.036024e-11, -1.6028400000000002e-10, -9.937287999999999e-09, 4.2383680000000005e-11, -1.1358554000000001e-08, 3.9725299999999996e-11, -1.0078494000000001e-08, 6.30498e-11, -7.550982e-09, 8.784526e-11, -5.557216e-10, -9.84718e-11, -7.308986e-09, -1.3814348000000002e-08, 7.365464000000002e-11, -8.052186000000001e-09, -1.1067396e-11, -2.554022e-09, -7.325092e-09, -7.05232e-09, -9.755659999999999e-09, -1.1196856000000001e-08, -1.4346882000000001e-08, -1.4860736000000002e-08, -1.5036204e-08, -1.3369388e-08, -1.0021694e-08, -9.621842e-09, -8.068194e-09, 5.4979339999999994e-11, 5.7530419999999994e-12, -3.246182e-09, -4.980356000000001e-09, -2.7533859999999997e-09, -6.70936e-09, -6.9177280000000005e-09, -1.4554624e-08, -1.4164096000000001e-08, -1.6854384e-08, -1.380222e-08, -7.668758e-09, -5.926224e-09, -1.1557444000000001e-08, -7.354524000000001e-09, -8.160112000000001e-09, -9.152704000000001e-09, -1.1161659999999998e-08, -8.21153e-09]}, {"V meas"=[0.236152, 0.234104, 0.236984, 0.234402, 0.22911, 0.233594, 0.239497, 0.228026, 0.22758, 0.229698, nan, nan, nan, nan, nan, nan, nan, nan, nan, nan, nan, nan, nan, nan, nan, nan, nan, nan, nan, nan, nan, nan, nan, nan, nan, nan, nan, nan, nan, nan, nan, nan, nan, nan, nan, nan, nan, nan, nan, nan, nan, nan, nan, nan, nan, nan, nan, nan, nan, nan, nan, nan, nan, nan, nan, nan, nan, nan, nan, nan, nan, nan, nan, nan, nan, nan, nan, nan, nan, nan, nan, nan, nan, nan, nan, nan, nan, nan, nan, nan, nan, nan, nan, nan, nan, nan, nan, nan, nan, nan, nan, nan, nan, nan], "I meas"=[-4.269804e-09, -5.041916000000001e-09, -4.6682759999999995e-09, -5.138274e-09, -4.799278e-09, -4.420012e-09, -3.2603080000000005e-09, -5.559286e-09, -5.365526e-09, -5.480968e-09, nan, nan, nan, nan, nan, nan, nan, nan, nan, nan, nan, nan, nan, nan, nan, nan, nan, nan, nan, nan, nan, nan, nan, nan, nan, nan, nan, nan, nan, nan, nan, nan, nan, nan, nan, nan, nan, nan, nan, nan, nan, nan, nan, nan, nan, nan, nan, nan, nan, nan, nan, nan, nan, nan, nan, nan, nan, nan, nan, nan, nan, nan, nan, nan, nan, nan, nan, nan, nan, nan, nan, nan, nan, nan, nan, nan, nan, nan, nan, nan, nan, nan, nan, nan, nan, nan, nan, nan, nan, nan, nan, nan, nan, nan]}]
  in  "FineTest save path":path=path "C:/Users/Flash/Desktop/Data/Detector test data/IV"
  out "I fine":dbl[](array[numeric])=[-1.52182e-05, -1.47166e-05, -1.48638e-05, -1.4948e-05, -1.49634e-05, -1.49403e-05, -1.48575e-05, -1.48749e-05, -1.47754e-05, -1.47251e-05, -1.46559e-05, -1.45851e-05, -1.45028e-05, -1.43852e-05, -1.42468e-05, -1.41684e-05, -1.40308e-05, -1.39364e-05, -1.37397e-05, -1.35679e-05, -1.3482e-05, -1.32093e-05, -1.2996e-05, -1.28281e-05, -1.25632e-05, -1.23417e-05, -1.20643e-05, -1.17371e-05, -1.14516e-05, -1.10657e-05, -1.06617e-05, -1.02025e-05, -9.26216e-06, -9.00798e-06, -8.21814e-06, -7.12779e-06, -5.50195e-06, -2.50105e-06, 4.02524e-06, 2.01571e-05]
  out "V fine":dbl[](array[numeric])=[-1.5, -1.45128, -1.40256, -1.35385, -1.30513, -1.25641, -1.20769, -1.15897, -1.11026, -1.06154, -1.01282, -0.964103, -0.915385, -0.866667, -0.817949, -0.769231, -0.720513, -0.671795, -0.623077, -0.574359, -0.525641, -0.476923, -0.428205, -0.379487, -0.330769, -0.282051, -0.233333, -0.184615, -0.135897, -0.0871795, -0.0384615, 0.0102564, 0.0589744, 0.107692, 0.15641, 0.205128, 0.253846, 0.302564, 0.351282, 0.4]
  out "Current Device":u32=10
  out "Total Device":u32=10
  out "IV fine log":cluster{dbl[], dbl[]}[](graph)=[{[-1.5, -1.45128, -1.40256, -1.35385, -1.30513, -1.25641, -1.20769, -1.15897, -1.11026, -1.06154, -1.01282, -0.964103, -0.915385, -0.866667, -0.817949, -0.769231, -0.720513, -0.671795, -0.623077, -0.574359, -0.525641, -0.476923, -0.428205, -0.379487, -0.330769, -0.282051, -0.233333, -0.184615, -0.135897, -0.0871795, -0.0384615, 0.0102564, 0.0589744, 0.107692, 0.15641, 0.205128, 0.253846, 0.302564, 0.351282, 0.4], [1.62518e-05, 1.59058e-05, 1.58552e-05, 1.58521e-05, 1.61136e-05, 1.58325e-05, 1.57837e-05, 1.57923e-05, 1.59421e-05, 1.57195e-05, 1.57072e-05, 1.57655e-05, 1.57462e-05, 1.56593e-05, 1.55775e-05, 1.56026e-05, 1.55346e-05, 1.54639e-05, 1.53912e-05, 1.53075e-05, 1.51382e-05, 1.50399e-05, 1.4928e-05, 1.47321e-05, 1.44447e-05, 1.42751e-05, 1.40992e-05, 1.37417e-05, 1.3347e-05, 1.30217e-05, 1.26796e-05, 1.21766e-05, 1.16136e-05, 1.09335e-05, 1.00961e-05, 8.60584e-06, 7.26446e-06, 4.26576e-06, 1.99124e-06, 1.66138e-05]}, {[-1.5, -1.45128, -1.40256, -1.35385, -1.30513, -1.25641, -1.20769, -1.15897, -1.11026, -1.06154, -1.01282, -0.964103, -0.915385, -0.866667, -0.817949, -0.769231, -0.720513, -0.671795, -0.623077, -0.574359, -0.525641, -0.476923, -0.428205, -0.379487, -0.330769, -0.282051, -0.233333, -0.184615, -0.135897, -0.0871795, -0.0384615, 0.0102564, 0.0589744, 0.107692, 0.15641, 0.205128, 0.253846, 0.302564, 0.351282, 0.4], [1.36029e-05, 1.39238e-05, 1.40077e-05, 1.39787e-05, 1.37902e-05, 1.38254e-05, 1.38807e-05, 1.39993e-05, 1.37559e-05, 1.37594e-05, 1.39334e-05, 1.38859e-05, 1.37374e-05, 1.37784e-05, 1.38315e-05, 1.3849e-05, 1.36736e-05, 1.36255e-05, 1.36181e-05, 1.35913e-05, 1.34346e-05, 1.33435e-05, 1.31651e-05, 1.30411e-05, 1.28623e-05, 1.27277e-05, 1.24139e-05, 1.2144e-05, 1.18426e-05, 1.15662e-05, 1.11112e-05, 1.06968e-05, 1.02089e-05, 9.22437e-06, 8.85657e-06, 7.82706e-06, 6.25243e-06, 3.38221e-06, 2.74369e-06, 1.77865e-05]}, {[-1.5, -1.45128, -1.40256, -1.35385, -1.30513, -1.25641, -1.20769, -1.15897, -1.11026, -1.06154, -1.01282, -0.964103, -0.915385, -0.866667, -0.817949, -0.769231, -0.720513, -0.671795, -0.623077, -0.574359, -0.525641, -0.476923, -0.428205, -0.379487, -0.330769, -0.282051, -0.233333, -0.184615, -0.135897, -0.0871795, -0.0384615, 0.0102564, 0.0589744, 0.107692, 0.15641, 0.205128, 0.253846, 0.302564, 0.351282, 0.4], [1.45487e-05, 1.44793e-05, 1.45091e-05, 1.45759e-05, 1.44845e-05, 1.44589e-05, 1.44101e-05, 1.43467e-05, 1.42634e-05, 1.42416e-05, 1.41538e-05, 1.39764e-05, 1.38688e-05, 1.37779e-05, 1.3677e-05, 1.34647e-05, 1.3336e-05, 1.32085e-05, 1.30882e-05, 1.28545e-05, 1.26536e-05, 1.24643e-05, 1.22342e-05, 1.20329e-05, 1.17647e-05, 1.14825e-05, 1.12311e-05, 1.09497e-05, 1.06108e-05, 1.02268e-05, 9.51786e-06, 9.44586e-06, 8.95039e-06, 8.37403e-06, 7.69201e-06, 6.79217e-06, 5.3745e-06, 2.81715e-06, 2.94395e-06, 1.74863e-05]}, {[-1.5, -1.45128, -1.40256, -1.35385, -1.30513, -1.25641, -1.20769, -1.15897, -1.11026, -1.06154, -1.01282, -0.964103, -0.915385, -0.866667, -0.817949, -0.769231, -0.720513, -0.671795, -0.623077, -0.574359, -0.525641, -0.476923, -0.428205, -0.379487, -0.330769, -0.282051, -0.233333, -0.184615, -0.135897, -0.0871795, -0.0384615, 0.0102564, 0.0589744, 0.107692, 0.15641, 0.205128, 0.253846, 0.302564, 0.351282, 0.4], [1.43268e-05, 1.41291e-05, 1.40792e-05, 1.40388e-05, 1.41617e-05, 1.40803e-05, 1.40236e-05, 1.39445e-05, 1.39384e-05, 1.3893e-05, 1.38786e-05, 1.38031e-05, 1.37261e-05, 1.37001e-05, 1.35949e-05, 1.3466e-05, 1.33568e-05, 1.31818e-05, 1.30797e-05, 1.28908e-05, 1.2725e-05, 1.25568e-05, 1.23307e-05, 1.21443e-05, 1.19645e-05, 1.17361e-05, 1.14207e-05, 1.11251e-05, 1.08126e-05, 1.04759e-05, 1.01039e-05, 9.29569e-06, 9.16141e-06, 8.54072e-06, 7.80004e-06, 6.80414e-06, 5.32019e-06, 2.59009e-06, 3.20517e-06, 1.73178e-05]}, {[-1.5, -1.45128, -1.40256, -1.35385, -1.30513, -1.25641, -1.20769, -1.15897, -1.11026, -1.06154, -1.01282, -0.964103, -0.915385, -0.866667, -0.817949, -0.769231, -0.720513, -0.671795, -0.623077, -0.574359, -0.525641, -0.476923, -0.428205, -0.379487, -0.330769, -0.282051, -0.233333, -0.184615, -0.135897, -0.0871795, -0.0384615, 0.0102564, 0.0589744, 0.107692, 0.15641, 0.205128, 0.253846, 0.302564, 0.351282, 0.4], [1.45128e-05, 1.44784e-05, 1.44337e-05, 1.45008e-05, 1.44765e-05, 1.44197e-05, 1.44825e-05, 1.44147e-05, 1.44257e-05, 1.44417e-05, 1.44472e-05, 1.43745e-05, 1.43881e-05, 1.43696e-05, 1.43656e-05, 1.44001e-05, 1.4292e-05, 1.43096e-05, 1.42966e-05, 1.42992e-05, 1.42272e-05, 1.41855e-05, 1.40808e-05, 1.39327e-05, 1.38064e-05, 1.37047e-05, 1.34936e-05, 1.32621e-05, 1.30014e-05, 1.26801e-05, 1.23085e-05, 1.18747e-05, 1.12903e-05, 1.06544e-05, 9.40974e-06, 8.59154e-06, 6.76655e-06, 3.48424e-06, 3.40767e-06, 1.98841e-05]}, {[-1.5, -1.45128, -1.40256, -1.35385, -1.30513, -1.25641, -1.20769, -1.15897, -1.11026, -1.06154, -1.01282, -0.964103, -0.915385, -0.866667, -0.817949, -0.769231, -0.720513, -0.671795, -0.623077, -0.574359, -0.525641, -0.476923, -0.428205, -0.379487, -0.330769, -0.282051, -0.233333, -0.184615, -0.135897, -0.0871795, -0.0384615, 0.0102564, 0.0589744, 0.107692, 0.15641, 0.205128, 0.253846, 0.302564, 0.351282, 0.4], [1.40475e-05, 1.4354e-05, 1.44564e-05, 1.44012e-05, 1.42809e-05, 1.43571e-05, 1.43786e-05, 1.43287e-05, 1.42537e-05, 1.42975e-05, 1.43208e-05, 1.42332e-05, 1.41469e-05, 1.41822e-05, 1.42689e-05, 1.42063e-05, 1.40896e-05, 1.39596e-05, 1.39855e-05, 1.39085e-05, 1.37852e-05, 1.36034e-05, 1.34773e-05, 1.33117e-05, 1.30942e-05, 1.28233e-05, 1.25734e-05, 1.22817e-05, 1.19194e-05, 1.16165e-05, 1.11835e-05, 1.07278e-05, 1.02202e-05, 9.20555e-06, 8.77193e-06, 7.70772e-06, 6.0801e-06, 3.16101e-06, 3.17945e-06, 1.88686e-05]}, {[-1.5, -1.45128, -1.40256, -1.35385, -1.30513, -1.25641, -1.20769, -1.15897, -1.11026, -1.06154, -1.01282, -0.964103, -0.915385, -0.866667, -0.817949, -0.769231, -0.720513, -0.671795, -0.623077, -0.574359, -0.525641, -0.476923, -0.428205, -0.379487, -0.330769, -0.282051, -0.233333, -0.184615, -0.135897, -0.0871795, -0.0384615, 0.0102564, 0.0589744, 0.107692, 0.15641, 0.205128, 0.253846, 0.302564, 0.351282, 0.4], [1.54351e-05, 1.50601e-05, 1.51056e-05, 1.52663e-05, 1.52168e-05, 1.51171e-05, 1.507e-05, 1.51743e-05, 1.51078e-05, 1.50298e-05, 1.49971e-05, 1.49526e-05, 1.49294e-05, 1.48765e-05, 1.46879e-05, 1.45901e-05, 1.44709e-05, 1.43723e-05, 1.41737e-05, 1.39806e-05, 1.37765e-05, 1.36025e-05, 1.338e-05, 1.30992e-05, 1.28407e-05, 1.25943e-05, 1.22959e-05, 1.19637e-05, 1.16023e-05, 1.12135e-05, 1.08209e-05, 1.03236e-05, 9.4587e-06, 9.22359e-06, 8.4509e-06, 7.48066e-06, 5.98309e-06, 3.29111e-06, 2.65596e-06, 1.74357e-05]}, {[-1.5, -1.45128, -1.40256, -1.35385, -1.30513, -1.25641, -1.20769, -1.15897, -1.11026, -1.06154, -1.01282, -0.964103, -0.915385, -0.866667, -0.817949, -0.769231, -0.720513, -0.671795, -0.623077, -0.574359, -0.525641, -0.476923, -0.428205, -0.379487, -0.330769, -0.282051, -0.233333, -0.184615, -0.135897, -0.0871795, -0.0384615, 0.0102564, 0.0589744, 0.107692, 0.15641, 0.205128, 0.253846, 0.302564, 0.351282, 0.4], [1.53447e-05, 1.47831e-05, 1.47122e-05, 1.46429e-05, 1.47243e-05, 1.47328e-05, 1.47086e-05, 1.46028e-05, 1.47432e-05, 1.47113e-05, 1.47218e-05, 1.46376e-05, 1.46699e-05, 1.46152e-05, 1.46717e-05, 1.46125e-05, 1.45853e-05, 1.46234e-05, 1.45533e-05, 1.44673e-05, 1.44896e-05, 1.4478e-05, 1.4459e-05, 1.43998e-05, 1.43584e-05, 1.425e-05, 1.42328e-05, 1.40931e-05, 1.38244e-05, 1.35004e-05, 1.31121e-05, 1.26449e-05, 1.20102e-05, 1.12588e-05, 1.02839e-05, 8.58833e-06, 6.90248e-06, 3.40666e-06, 3.80601e-06, 2.08878e-05]}, {[-1.5, -1.45128, -1.40256, -1.35385, -1.30513, -1.25641, -1.20769, -1.15897, -1.11026, -1.06154, -1.01282, -0.964103, -0.915385, -0.866667, -0.817949, -0.769231, -0.720513, -0.671795, -0.623077, -0.574359, -0.525641, -0.476923, -0.428205, -0.379487, -0.330769, -0.282051, -0.233333, -0.184615, -0.135897, -0.0871795, -0.0384615, 0.0102564, 0.0589744, 0.107692, 0.15641, 0.205128, 0.253846, 0.302564, 0.351282, 0.4], [1.44727e-05, 1.4384e-05, 1.44688e-05, 1.43704e-05, 1.43565e-05, 1.44014e-05, 1.44225e-05, 1.44796e-05, 1.43648e-05, 1.4355e-05, 1.43902e-05, 1.4375e-05, 1.43596e-05, 1.42258e-05, 1.43194e-05, 1.43306e-05, 1.42962e-05, 1.41932e-05, 1.41703e-05, 1.40789e-05, 1.41097e-05, 1.39534e-05, 1.39183e-05, 1.38152e-05, 1.36883e-05, 1.34469e-05, 1.32306e-05, 1.29288e-05, 1.27267e-05, 1.23973e-05, 1.19846e-05, 1.14551e-05, 1.08658e-05, 1.01658e-05, 8.93522e-06, 8.01026e-06, 6.20114e-06, 2.94987e-06, 3.83666e-06, 2.00962e-05]}, {[-1.5, -1.45128, -1.40256, -1.35385, -1.30513, -1.25641, -1.20769, -1.15897, -1.11026, -1.06154, -1.01282, -0.964103, -0.915385, -0.866667, -0.817949, -0.769231, -0.720513, -0.671795, -0.623077, -0.574359, -0.525641, -0.476923, -0.428205, -0.379487, -0.330769, -0.282051, -0.233333, -0.184615, -0.135897, -0.0871795, -0.0384615, 0.0102564, 0.0589744, 0.107692, 0.15641, 0.205128, 0.253846, 0.302564, 0.351282, 0.4], [1.52182e-05, 1.47166e-05, 1.48638e-05, 1.4948e-05, 1.49634e-05, 1.49403e-05, 1.48575e-05, 1.48749e-05, 1.47754e-05, 1.47251e-05, 1.46559e-05, 1.45851e-05, 1.45028e-05, 1.43852e-05, 1.42468e-05, 1.41684e-05, 1.40308e-05, 1.39364e-05, 1.37397e-05, 1.35679e-05, 1.3482e-05, 1.32093e-05, 1.2996e-05, 1.28281e-05, 1.25632e-05, 1.23417e-05, 1.20643e-05, 1.17371e-05, 1.14516e-05, 1.10657e-05, 1.06617e-05, 1.02025e-05, 9.26216e-06, 9.00798e-06, 8.21814e-06, 7.12779e-06, 5.50195e-06, 2.50105e-06, 4.02524e-06, 2.01571e-05]}]
  out "Progress 2":u8(slide)=100 scale=0.0..100.0
  in  "StartFine":bool
  out "IV fine linear":cluster{dbl[], dbl[]}[](graph)=[{[-1.5, -1.45128, -1.40256, -1.35385, -1.30513, -1.25641, -1.20769, -1.15897, -1.11026, -1.06154, -1.01282, -0.964103, -0.915385, -0.866667, -0.817949, -0.769231, -0.720513, -0.671795, -0.623077, -0.574359, -0.525641, -0.476923, -0.428205, -0.379487, -0.330769, -0.282051, -0.233333, -0.184615, -0.135897, -0.0871795, -0.0384615, 0.0102564, 0.0589744, 0.107692, 0.15641, 0.205128, 0.253846, 0.302564, 0.351282, 0.4], [-1.62518e-05, -1.59058e-05, -1.58552e-05, -1.58521e-05, -1.61136e-05, -1.58325e-05, -1.57837e-05, -1.57923e-05, -1.59421e-05, -1.57195e-05, -1.57072e-05, -1.57655e-05, -1.57462e-05, -1.56593e-05, -1.55775e-05, -1.56026e-05, -1.55346e-05, -1.54639e-05, -1.53912e-05, -1.53075e-05, -1.51382e-05, -1.50399e-05, -1.4928e-05, -1.47321e-05, -1.44447e-05, -1.42751e-05, -1.40992e-05, -1.37417e-05, -1.3347e-05, -1.30217e-05, -1.26796e-05, -1.21766e-05, -1.16136e-05, -1.09335e-05, -1.00961e-05, -8.60584e-06, -7.26446e-06, -4.26576e-06, 1.99124e-06, 1.66138e-05]}, {[-1.5, -1.45128, -1.40256, -1.35385, -1.30513, -1.25641, -1.20769, -1.15897, -1.11026, -1.06154, -1.01282, -0.964103, -0.915385, -0.866667, -0.817949, -0.769231, -0.720513, -0.671795, -0.623077, -0.574359, -0.525641, -0.476923, -0.428205, -0.379487, -0.330769, -0.282051, -0.233333, -0.184615, -0.135897, -0.0871795, -0.0384615, 0.0102564, 0.0589744, 0.107692, 0.15641, 0.205128, 0.253846, 0.302564, 0.351282, 0.4], [-1.36029e-05, -1.39238e-05, -1.40077e-05, -1.39787e-05, -1.37902e-05, -1.38254e-05, -1.38807e-05, -1.39993e-05, -1.37559e-05, -1.37594e-05, -1.39334e-05, -1.38859e-05, -1.37374e-05, -1.37784e-05, -1.38315e-05, -1.3849e-05, -1.36736e-05, -1.36255e-05, -1.36181e-05, -1.35913e-05, -1.34346e-05, -1.33435e-05, -1.31651e-05, -1.30411e-05, -1.28623e-05, -1.27277e-05, -1.24139e-05, -1.2144e-05, -1.18426e-05, -1.15662e-05, -1.11112e-05, -1.06968e-05, -1.02089e-05, -9.22437e-06, -8.85657e-06, -7.82706e-06, -6.25243e-06, -3.38221e-06, 2.74369e-06, 1.77865e-05]}, {[-1.5, -1.45128, -1.40256, -1.35385, -1.30513, -1.25641, -1.20769, -1.15897, -1.11026, -1.06154, -1.01282, -0.964103, -0.915385, -0.866667, -0.817949, -0.769231, -0.720513, -0.671795, -0.623077, -0.574359, -0.525641, -0.476923, -0.428205, -0.379487, -0.330769, -0.282051, -0.233333, -0.184615, -0.135897, -0.0871795, -0.0384615, 0.0102564, 0.0589744, 0.107692, 0.15641, 0.205128, 0.253846, 0.302564, 0.351282, 0.4], [-1.45487e-05, -1.44793e-05, -1.45091e-05, -1.45759e-05, -1.44845e-05, -1.44589e-05, -1.44101e-05, -1.43467e-05, -1.42634e-05, -1.42416e-05, -1.41538e-05, -1.39764e-05, -1.38688e-05, -1.37779e-05, -1.3677e-05, -1.34647e-05, -1.3336e-05, -1.32085e-05, -1.30882e-05, -1.28545e-05, -1.26536e-05, -1.24643e-05, -1.22342e-05, -1.20329e-05, -1.17647e-05, -1.14825e-05, -1.12311e-05, -1.09497e-05, -1.06108e-05, -1.02268e-05, -9.51786e-06, -9.44586e-06, -8.95039e-06, -8.37403e-06, -7.69201e-06, -6.79217e-06, -5.3745e-06, -2.81715e-06, 2.94395e-06, 1.74863e-05]}, {[-1.5, -1.45128, -1.40256, -1.35385, -1.30513, -1.25641, -1.20769, -1.15897, -1.11026, -1.06154, -1.01282, -0.964103, -0.915385, -0.866667, -0.817949, -0.769231, -0.720513, -0.671795, -0.623077, -0.574359, -0.525641, -0.476923, -0.428205, -0.379487, -0.330769, -0.282051, -0.233333, -0.184615, -0.135897, -0.0871795, -0.0384615, 0.0102564, 0.0589744, 0.107692, 0.15641, 0.205128, 0.253846, 0.302564, 0.351282, 0.4], [-1.43268e-05, -1.41291e-05, -1.40792e-05, -1.40388e-05, -1.41617e-05, -1.40803e-05, -1.40236e-05, -1.39445e-05, -1.39384e-05, -1.3893e-05, -1.38786e-05, -1.38031e-05, -1.37261e-05, -1.37001e-05, -1.35949e-05, -1.3466e-05, -1.33568e-05, -1.31818e-05, -1.30797e-05, -1.28908e-05, -1.2725e-05, -1.25568e-05, -1.23307e-05, -1.21443e-05, -1.19645e-05, -1.17361e-05, -1.14207e-05, -1.11251e-05, -1.08126e-05, -1.04759e-05, -1.01039e-05, -9.29569e-06, -9.16141e-06, -8.54072e-06, -7.80004e-06, -6.80414e-06, -5.32019e-06, -2.59009e-06, 3.20517e-06, 1.73178e-05]}, {[-1.5, -1.45128, -1.40256, -1.35385, -1.30513, -1.25641, -1.20769, -1.15897, -1.11026, -1.06154, -1.01282, -0.964103, -0.915385, -0.866667, -0.817949, -0.769231, -0.720513, -0.671795, -0.623077, -0.574359, -0.525641, -0.476923, -0.428205, -0.379487, -0.330769, -0.282051, -0.233333, -0.184615, -0.135897, -0.0871795, -0.0384615, 0.0102564, 0.0589744, 0.107692, 0.15641, 0.205128, 0.253846, 0.302564, 0.351282, 0.4], [-1.45128e-05, -1.44784e-05, -1.44337e-05, -1.45008e-05, -1.44765e-05, -1.44197e-05, -1.44825e-05, -1.44147e-05, -1.44257e-05, -1.44417e-05, -1.44472e-05, -1.43745e-05, -1.43881e-05, -1.43696e-05, -1.43656e-05, -1.44001e-05, -1.4292e-05, -1.43096e-05, -1.42966e-05, -1.42992e-05, -1.42272e-05, -1.41855e-05, -1.40808e-05, -1.39327e-05, -1.38064e-05, -1.37047e-05, -1.34936e-05, -1.32621e-05, -1.30014e-05, -1.26801e-05, -1.23085e-05, -1.18747e-05, -1.12903e-05, -1.06544e-05, -9.40974e-06, -8.59154e-06, -6.76655e-06, -3.48424e-06, 3.40767e-06, 1.98841e-05]}, {[-1.5, -1.45128, -1.40256, -1.35385, -1.30513, -1.25641, -1.20769, -1.15897, -1.11026, -1.06154, -1.01282, -0.964103, -0.915385, -0.866667, -0.817949, -0.769231, -0.720513, -0.671795, -0.623077, -0.574359, -0.525641, -0.476923, -0.428205, -0.379487, -0.330769, -0.282051, -0.233333, -0.184615, -0.135897, -0.0871795, -0.0384615, 0.0102564, 0.0589744, 0.107692, 0.15641, 0.205128, 0.253846, 0.302564, 0.351282, 0.4], [-1.40475e-05, -1.4354e-05, -1.44564e-05, -1.44012e-05, -1.42809e-05, -1.43571e-05, -1.43786e-05, -1.43287e-05, -1.42537e-05, -1.42975e-05, -1.43208e-05, -1.42332e-05, -1.41469e-05, -1.41822e-05, -1.42689e-05, -1.42063e-05, -1.40896e-05, -1.39596e-05, -1.39855e-05, -1.39085e-05, -1.37852e-05, -1.36034e-05, -1.34773e-05, -1.33117e-05, -1.30942e-05, -1.28233e-05, -1.25734e-05, -1.22817e-05, -1.19194e-05, -1.16165e-05, -1.11835e-05, -1.07278e-05, -1.02202e-05, -9.20555e-06, -8.77193e-06, -7.70772e-06, -6.0801e-06, -3.16101e-06, 3.17945e-06, 1.88686e-05]}, {[-1.5, -1.45128, -1.40256, -1.35385, -1.30513, -1.25641, -1.20769, -1.15897, -1.11026, -1.06154, -1.01282, -0.964103, -0.915385, -0.866667, -0.817949, -0.769231, -0.720513, -0.671795, -0.623077, -0.574359, -0.525641, -0.476923, -0.428205, -0.379487, -0.330769, -0.282051, -0.233333, -0.184615, -0.135897, -0.0871795, -0.0384615, 0.0102564, 0.0589744, 0.107692, 0.15641, 0.205128, 0.253846, 0.302564, 0.351282, 0.4], [-1.54351e-05, -1.50601e-05, -1.51056e-05, -1.52663e-05, -1.52168e-05, -1.51171e-05, -1.507e-05, -1.51743e-05, -1.51078e-05, -1.50298e-05, -1.49971e-05, -1.49526e-05, -1.49294e-05, -1.48765e-05, -1.46879e-05, -1.45901e-05, -1.44709e-05, -1.43723e-05, -1.41737e-05, -1.39806e-05, -1.37765e-05, -1.36025e-05, -1.338e-05, -1.30992e-05, -1.28407e-05, -1.25943e-05, -1.22959e-05, -1.19637e-05, -1.16023e-05, -1.12135e-05, -1.08209e-05, -1.03236e-05, -9.4587e-06, -9.22359e-06, -8.4509e-06, -7.48066e-06, -5.98309e-06, -3.29111e-06, 2.65596e-06, 1.74357e-05]}, {[-1.5, -1.45128, -1.40256, -1.35385, -1.30513, -1.25641, -1.20769, -1.15897, -1.11026, -1.06154, -1.01282, -0.964103, -0.915385, -0.866667, -0.817949, -0.769231, -0.720513, -0.671795, -0.623077, -0.574359, -0.525641, -0.476923, -0.428205, -0.379487, -0.330769, -0.282051, -0.233333, -0.184615, -0.135897, -0.0871795, -0.0384615, 0.0102564, 0.0589744, 0.107692, 0.15641, 0.205128, 0.253846, 0.302564, 0.351282, 0.4], [-1.53447e-05, -1.47831e-05, -1.47122e-05, -1.46429e-05, -1.47243e-05, -1.47328e-05, -1.47086e-05, -1.46028e-05, -1.47432e-05, -1.47113e-05, -1.47218e-05, -1.46376e-05, -1.46699e-05, -1.46152e-05, -1.46717e-05, -1.46125e-05, -1.45853e-05, -1.46234e-05, -1.45533e-05, -1.44673e-05, -1.44896e-05, -1.4478e-05, -1.4459e-05, -1.43998e-05, -1.43584e-05, -1.425e-05, -1.42328e-05, -1.40931e-05, -1.38244e-05, -1.35004e-05, -1.31121e-05, -1.26449e-05, -1.20102e-05, -1.12588e-05, -1.02839e-05, -8.58833e-06, -6.90248e-06, -3.40666e-06, 3.80601e-06, 2.08878e-05]}, {[-1.5, -1.45128, -1.40256, -1.35385, -1.30513, -1.25641, -1.20769, -1.15897, -1.11026, -1.06154, -1.01282, -0.964103, -0.915385, -0.866667, -0.817949, -0.769231, -0.720513, -0.671795, -0.623077, -0.574359, -0.525641, -0.476923, -0.428205, -0.379487, -0.330769, -0.282051, -0.233333, -0.184615, -0.135897, -0.0871795, -0.0384615, 0.0102564, 0.0589744, 0.107692, 0.15641, 0.205128, 0.253846, 0.302564, 0.351282, 0.4], [-1.44727e-05, -1.4384e-05, -1.44688e-05, -1.43704e-05, -1.43565e-05, -1.44014e-05, -1.44225e-05, -1.44796e-05, -1.43648e-05, -1.4355e-05, -1.43902e-05, -1.4375e-05, -1.43596e-05, -1.42258e-05, -1.43194e-05, -1.43306e-05, -1.42962e-05, -1.41932e-05, -1.41703e-05, -1.40789e-05, -1.41097e-05, -1.39534e-05, -1.39183e-05, -1.38152e-05, -1.36883e-05, -1.34469e-05, -1.32306e-05, -1.29288e-05, -1.27267e-05, -1.23973e-05, -1.19846e-05, -1.14551e-05, -1.08658e-05, -1.01658e-05, -8.93522e-06, -8.01026e-06, -6.20114e-06, -2.94987e-06, 3.83666e-06, 2.00962e-05]}, {[-1.5, -1.45128, -1.40256, -1.35385, -1.30513, -1.25641, -1.20769, -1.15897, -1.11026, -1.06154, -1.01282, -0.964103, -0.915385, -0.866667, -0.817949, -0.769231, -0.720513, -0.671795, -0.623077, -0.574359, -0.525641, -0.476923, -0.428205, -0.379487, -0.330769, -0.282051, -0.233333, -0.184615, -0.135897, -0.0871795, -0.0384615, 0.0102564, 0.0589744, 0.107692, 0.15641, 0.205128, 0.253846, 0.302564, 0.351282, 0.4], [-1.52182e-05, -1.47166e-05, -1.48638e-05, -1.4948e-05, -1.49634e-05, -1.49403e-05, -1.48575e-05, -1.48749e-05, -1.47754e-05, -1.47251e-05, -1.46559e-05, -1.45851e-05, -1.45028e-05, -1.43852e-05, -1.42468e-05, -1.41684e-05, -1.40308e-05, -1.39364e-05, -1.37397e-05, -1.35679e-05, -1.3482e-05, -1.32093e-05, -1.2996e-05, -1.28281e-05, -1.25632e-05, -1.23417e-05, -1.20643e-05, -1.17371e-05, -1.14516e-05, -1.10657e-05, -1.06617e-05, -1.02025e-05, -9.26216e-06, -9.00798e-06, -8.21814e-06, -7.12779e-06, -5.50195e-06, -2.50105e-06, 4.02524e-06, 2.01571e-05]}]
  in  "Mask File Fine":path=path "C:/Users/Flash/Desktop/Data/Detector test data/SL066_mask_map_file_V3_align on D3000_Diode_Open_1000_A-3348-2-A_1000123103_040000.0PM.csv"
  in  "Prober GPIB":string="0:1"
  in  "SMU":refnum<visa-resource-name>="GPIB0::26::INSTR"
  in  "Channel":enum32{"Channel A", "Channel B"}(ring)
  # "0 is for dark IV!"
  # "Sweep Settings"
  # "Forward Voltage"
  # "Dark/Light Current"
  # "Check settings before click start!"
  # "Make sure current x and y are same as prober before click Start!"
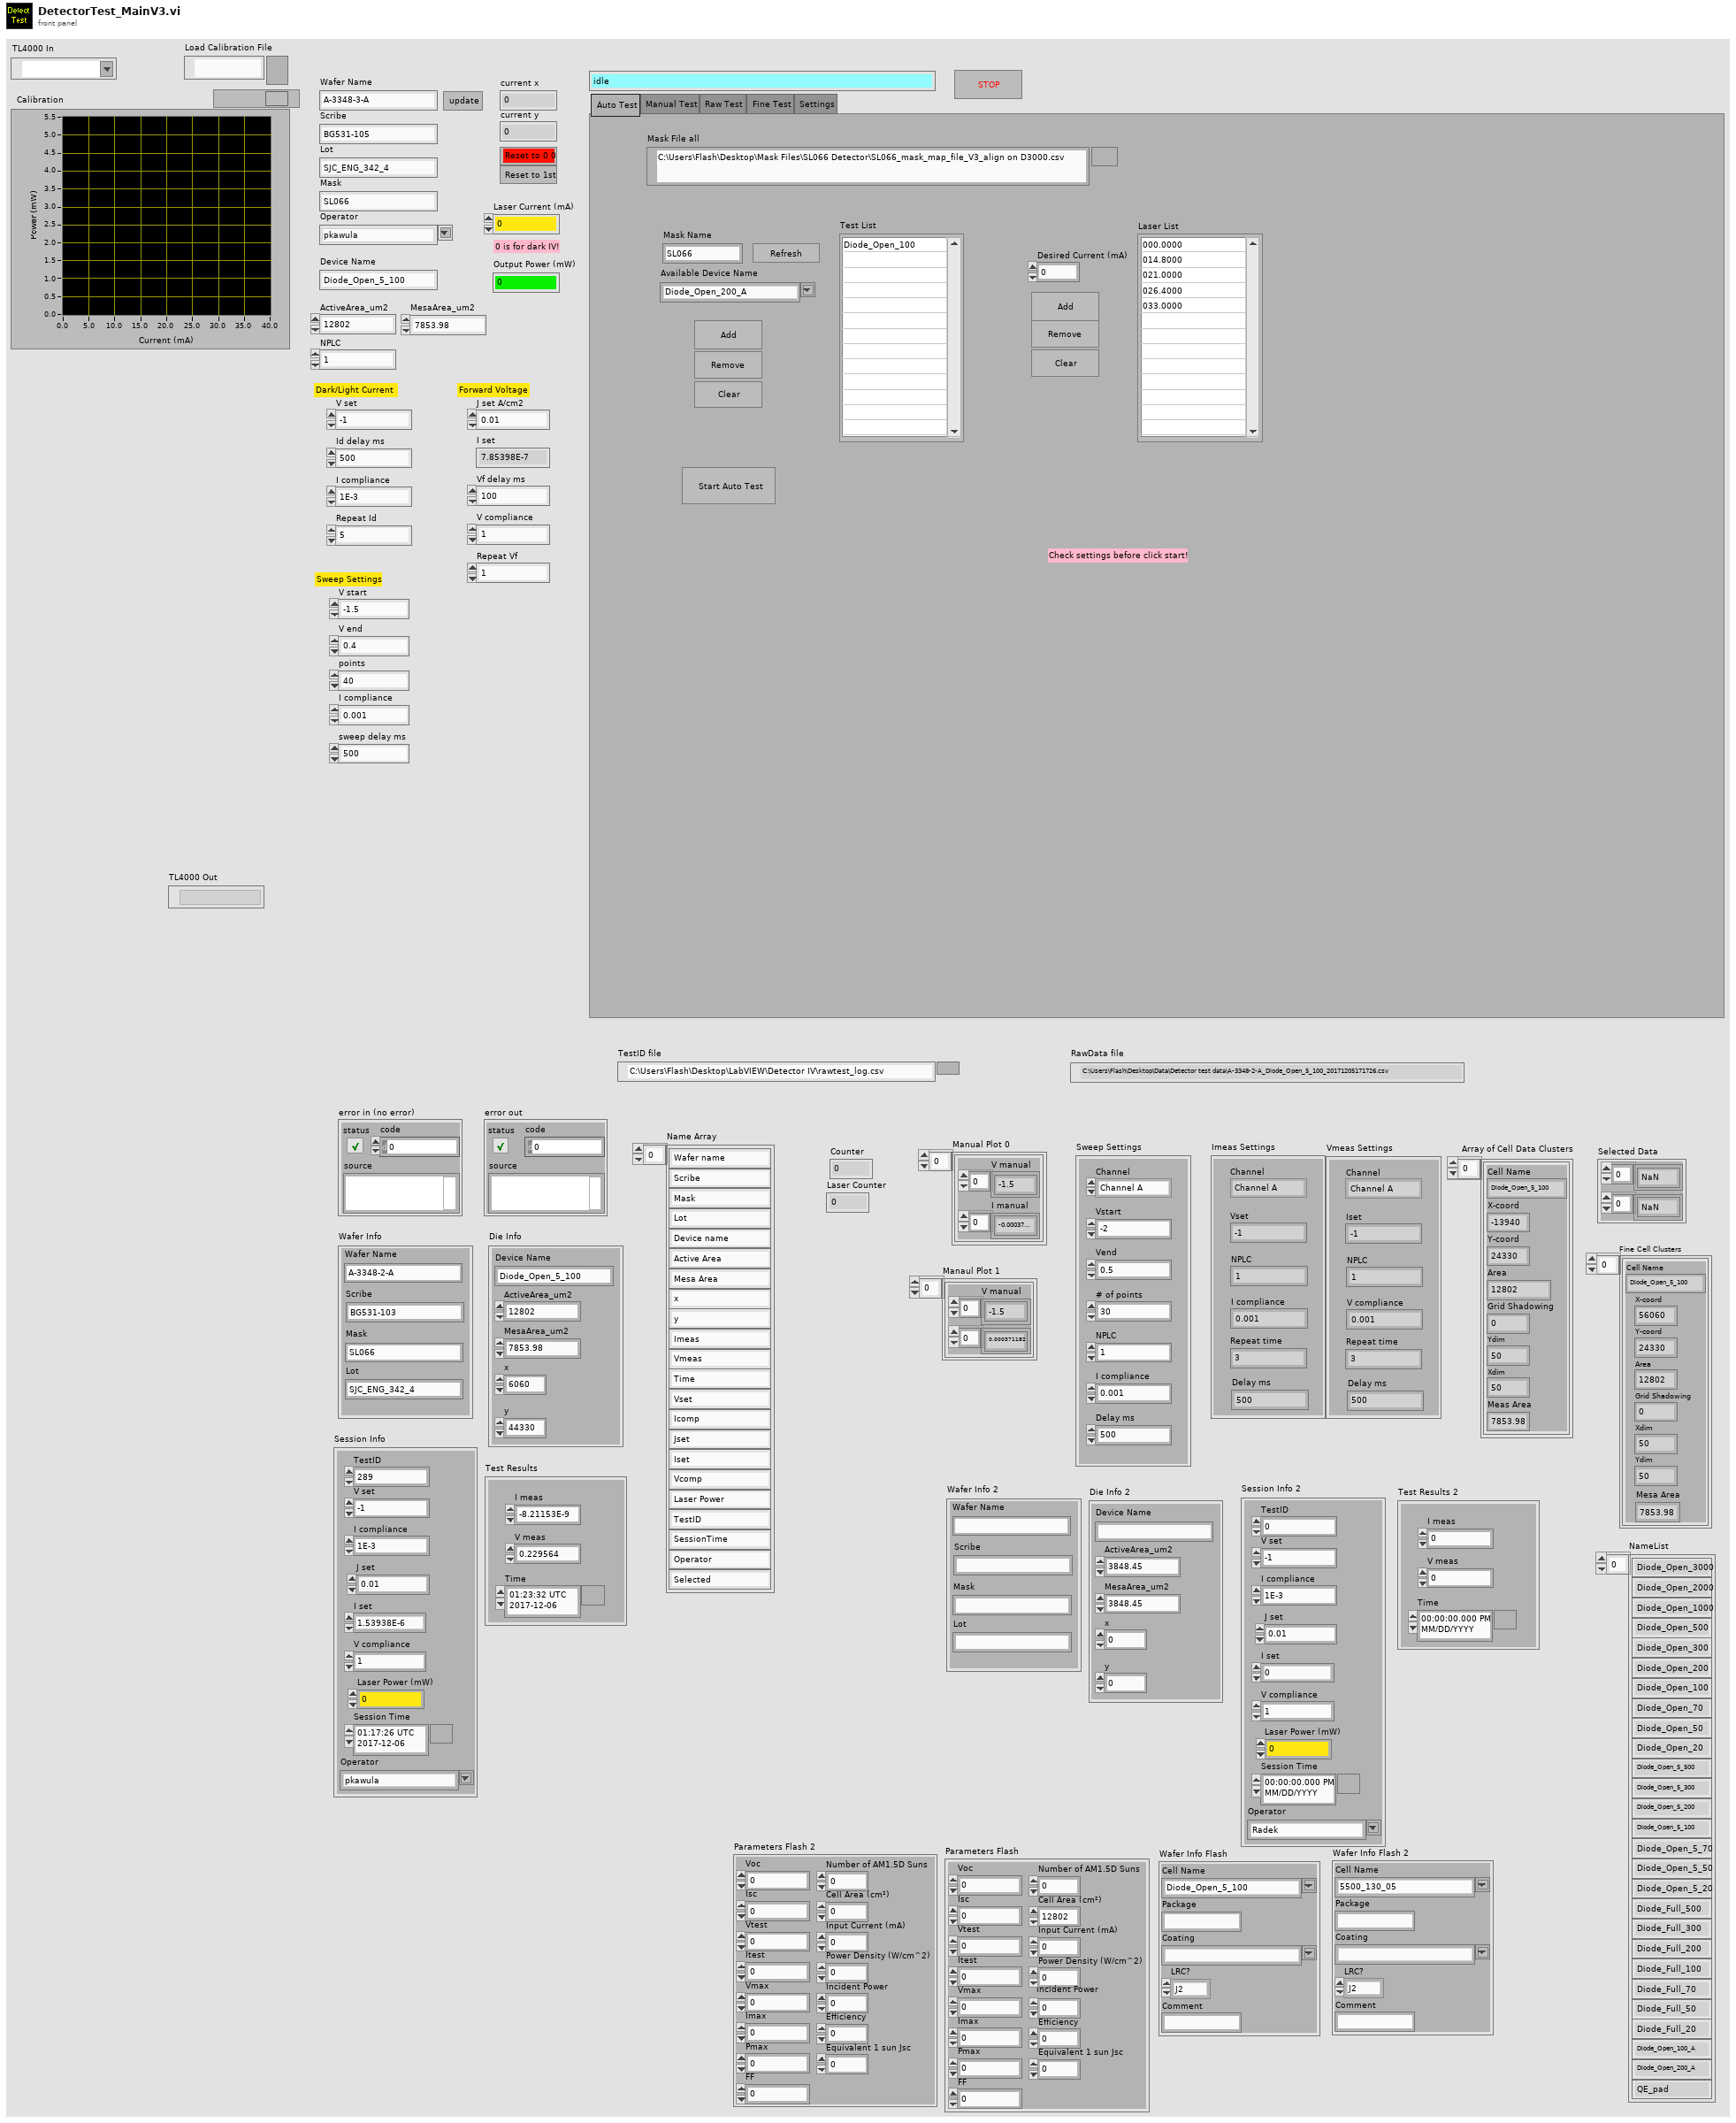
[diagram p1: front panel]
types:
  T1 = cluster{"Cell Name":string, "Package":string, "Coating":string, "LRC?":enum16{"J1", "J2", "LRC"}, "Comment":string}
  T2 = cluster{"Voc":dbl, "Isc":dbl, "FF":dbl, "Vtest":dbl, "Imax":dbl, "Vmax":dbl, "Pmax":dbl, "Itest":dbl, "Efficiency":dbl, "Incident Power":dbl, "Power Density (W/cm^2)":dbl, "Cell Area (cm²)":dbl, "Number of AM1.5D Suns":dbl, "Input Current (mA)":dbl, "Equivalent 1 sun Jsc":dbl}
  T3 = cluster{"Cell Name":string, "X-coord":dbl, "Y-coord":dbl, "Area":dbl, "Grid Shadowing":dbl, "Xdim":dbl, "Ydim":dbl, "Mesa Area":dbl}[]
  T4 = cluster{"I meas":dbl, "V meas":dbl, "Time":timestamp}
  T5 = cluster{"V set":dbl, "I compliance":dbl, "J set":dbl, "I set":dbl, "V compliance":dbl, "Laser Power (mW)":dbl, "TestID":u32, "Session Time":timestamp, "Operator":string}
  T6 = cluster{"Device Name":string, "ActiveArea_um2":dbl, "MesaArea_um2":dbl, "x":dbl, "y":dbl}
  T7 = cluster{"Wafer Name":string, "Scribe":string, "Mask":string, "Lot":string}
  T8 = cluster{"Channel":enum32{"Channel A", "Channel B"}, "Vstart":dbl, "Vend":dbl, "# of points":u16, "NPLC":dbl, "I compliance":dbl, "Delay ms":dbl}
  T9 = cluster{"Channel":enum32{"Channel A", "Channel B"}, "Iset":dbl, "NPLC":dbl, "V compliance":dbl, "Repeat time":u16, "Delay ms":dbl}
  T10 = cluster{"Channel":enum32{"Channel A", "Channel B"}, "Vset":dbl, "NPLC":dbl, "I compliance":dbl, "Repeat time":u16, "Delay ms":dbl}
  T11 = cluster{"Cell Name":string, "X-coord":dbl, "Y-coord":dbl, "Area":dbl, "Grid Shadowing":dbl, "Ydim":dbl, "Xdim":dbl, "Meas Area":dbl}[]
  T12 = enum32{"Auto Test", "Manual Test", "Raw Test", "Fine Test", "Settings"}
  T13 = cluster{"X Values":dbl[], "Histogram: h(x)":i32[]}
  T14 = cluster{"Cell Name":string, "X-coord":dbl, "Y-coord":dbl, "Area":dbl, "Grid Shadowing":dbl, "Ydim":dbl, "Xdim":dbl, "Meas Area":dbl}
  T15 = cluster{"Varray manual":dbl[], "Iarray manual":dbl[]}[]
  T16 = cluster{"WaferName":string, "Scribe":string, "Structure":string, "Lot":string, "Mask":string}
  T17 = cluster{"V set":dbl, "I compliance":dbl, "J set":dbl, "I set":dbl, "V compliance":dbl, "Laser Power (mW)":dbl, "TestID":u32, "Operator":string}
  T18 = cluster{"Device Name":string, "ActiveArea_um2":dbl, "MesaArea_um2":dbl}
  T19 = cluster{"Cell Name":string, "X-coord":dbl, "Y-coord":dbl, "Area":dbl, "Grid Shadowing":dbl, "Xdim":dbl, "Ydim":dbl, "Mesa Area":dbl}
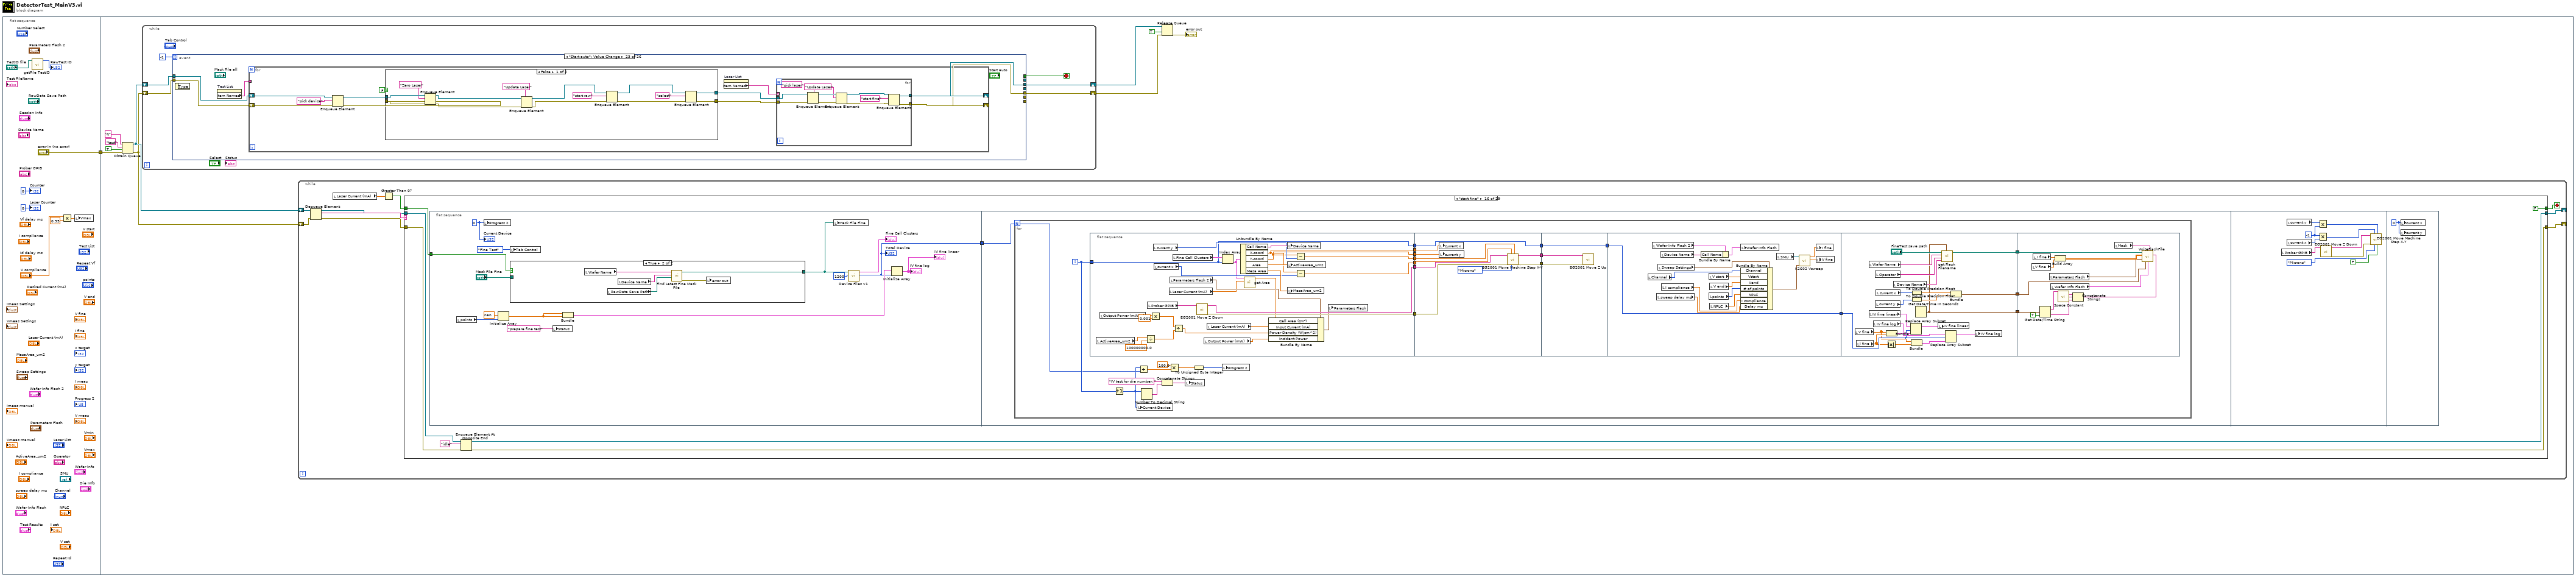
[diagram p0: block diagram]
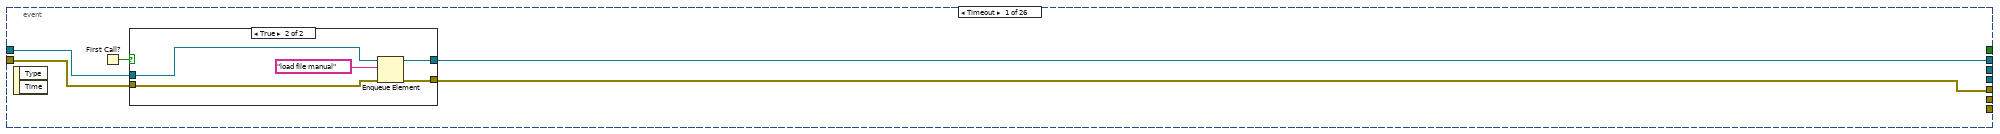
[diagram p2: hidden frame]
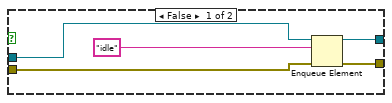
[diagram p3: hidden frame]
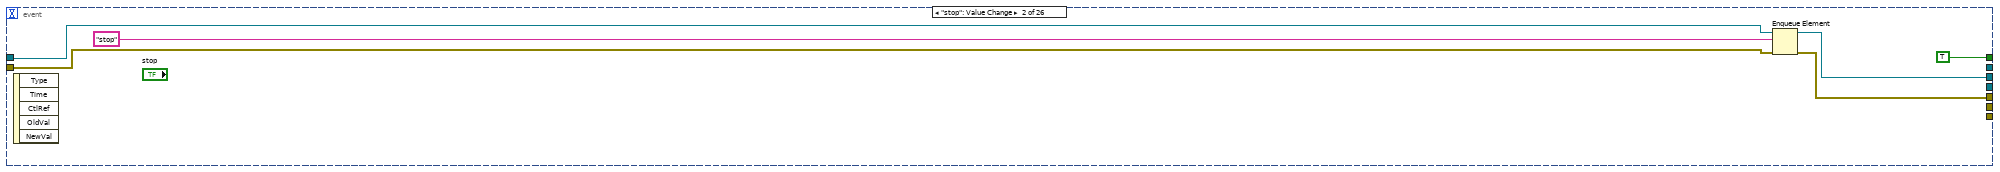
[diagram p4: hidden frame]
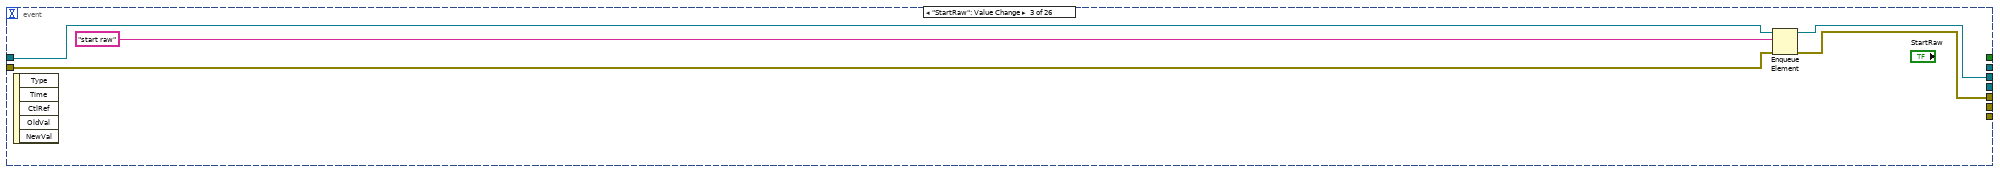
[diagram p5: hidden frame]
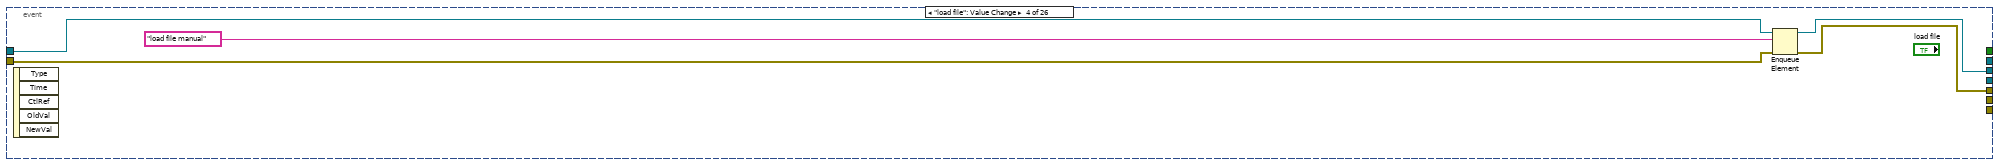
[diagram p6: hidden frame]
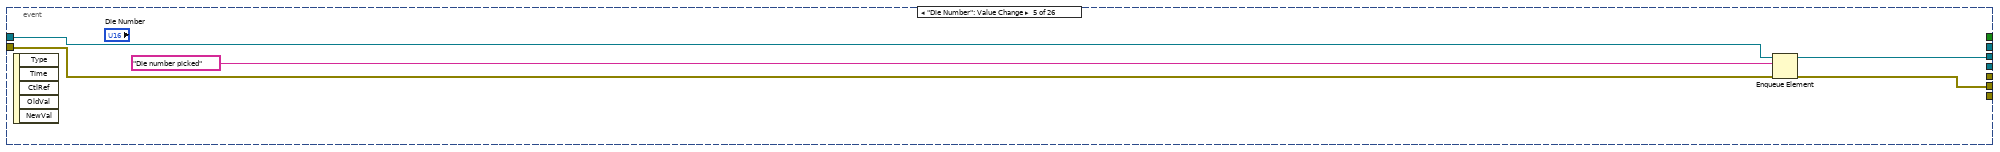
[diagram p7: hidden frame]
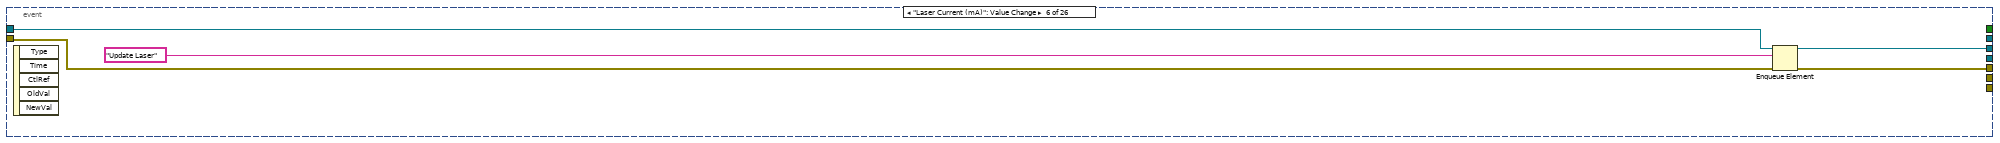
[diagram p8: hidden frame]
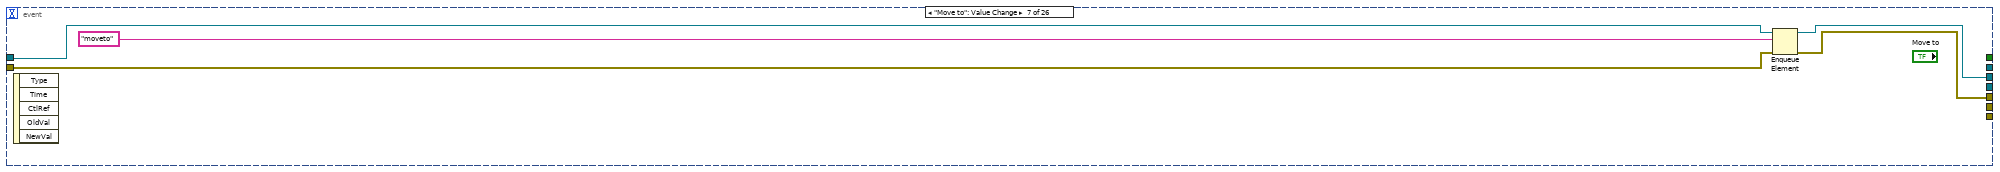
[diagram p9: hidden frame]
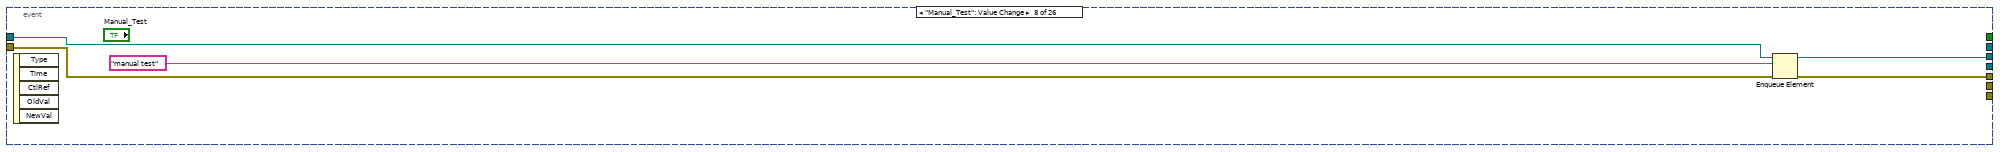
[diagram p10: hidden frame]
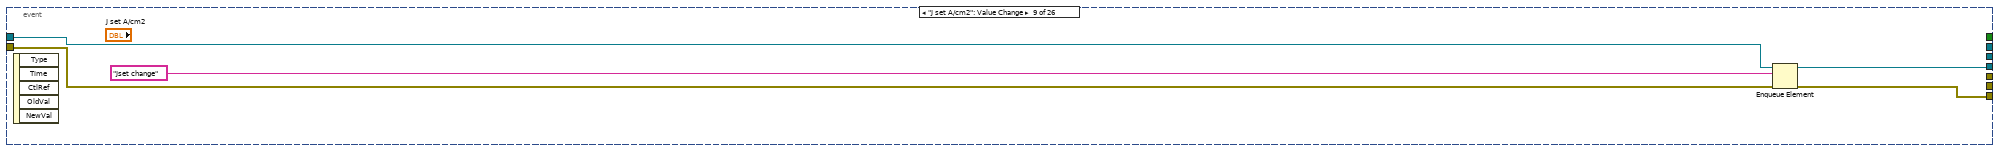
[diagram p11: hidden frame]
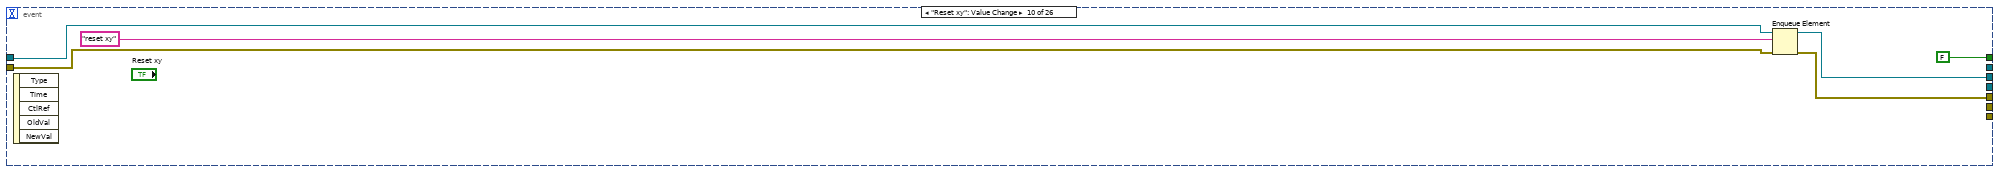
[diagram p12: hidden frame]
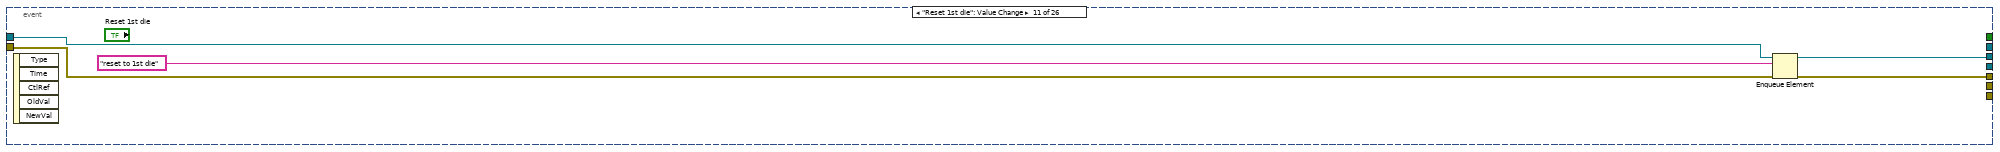
[diagram p13: hidden frame]
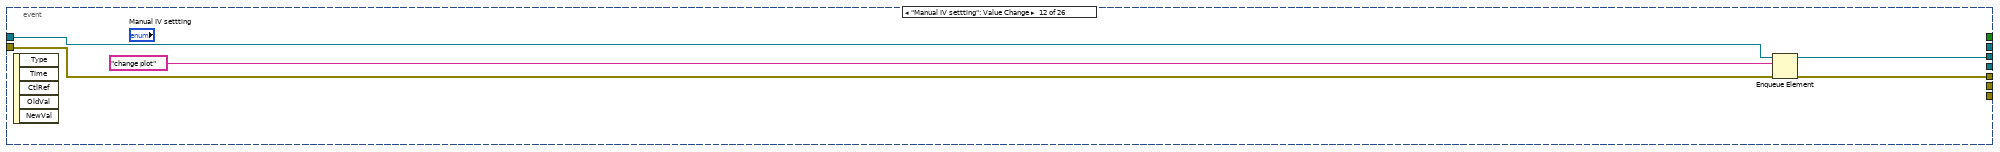
[diagram p14: hidden frame]
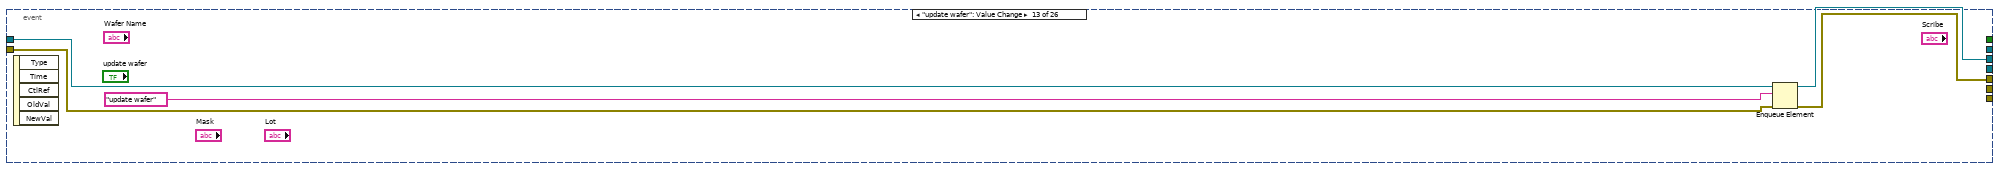
[diagram p15: hidden frame]
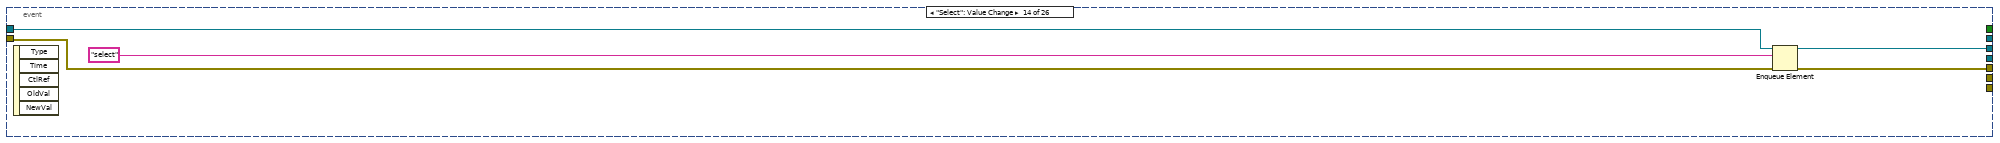
[diagram p16: hidden frame]
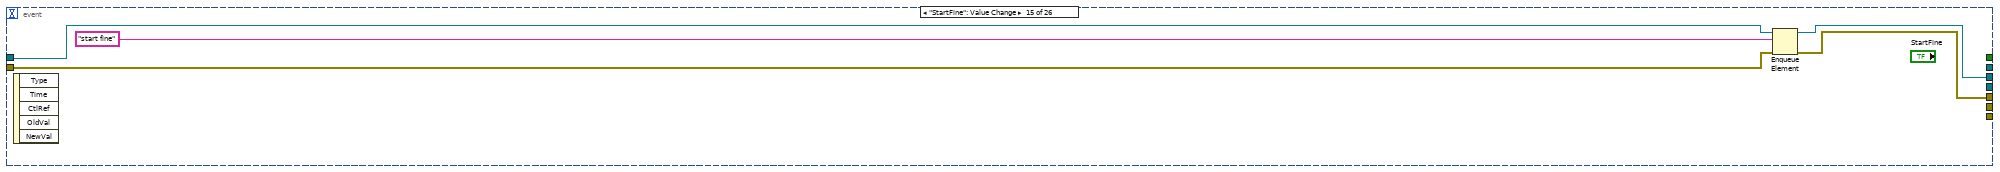
[diagram p17: hidden frame]
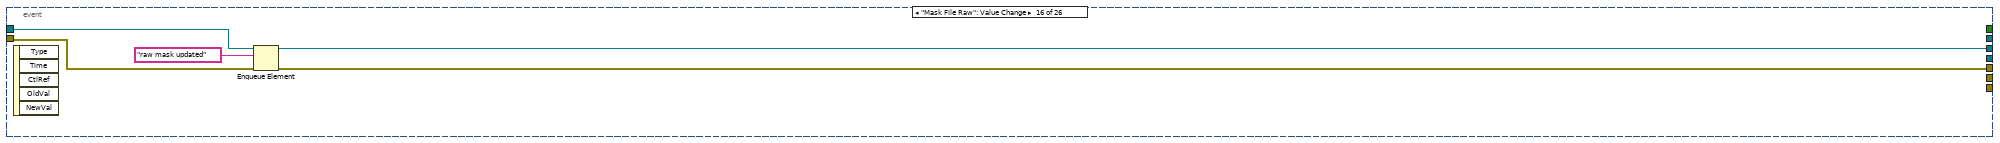
[diagram p18: hidden frame]
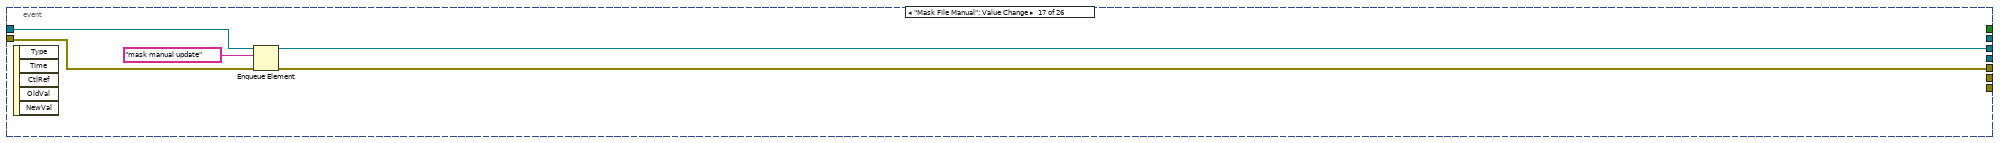
[diagram p19: hidden frame]
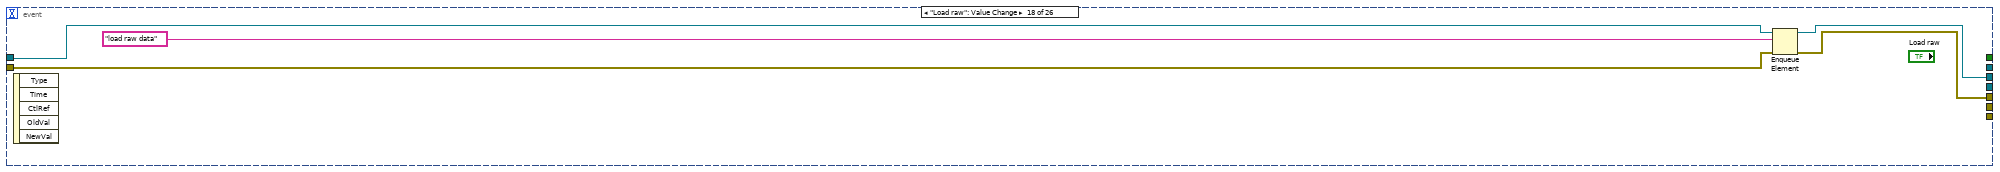
[diagram p20: hidden frame]
diagram:
  n1 = flat-sequence {
    tunnel: ["error in (no error)"] -> w1
    tunnel: w1 -> [w16]
    frame #0 {
      n2 = call "getFile TestID.vi"("Path"="TestID file") -> ("TestID"=→"RawTest ID":u32)  [unwired: 9 in, 1 out]
      n3 = Multiply(x="V compliance", y=0.95) -> (x*y=w4:dbl)
      n4 = local write "Vmax"(w4) -> ()
      "Counter" <- u32 0 ("Counter")
      "Laser Counter" <- u32 0 ("Counter")
    }
    frame #1 {
      n5 = Obtain Queue(name (unnamed)="q", element data type="test" ("name (unnamed)"), create if not found? (T)=TRUE, error in (no error)=w16) -> (queue out=w18:refnum<queue>, error out=w17:errorcluster)  [unwired: 1 in, 1 out]
      n6 = while {
        shift-right: [w23] -> w19
        shift-left: w18 -> [w24]
        shift-right: [w21] -> w10
        shift-left: w17 -> [w22]
        stop <- w25 stop-if-true
        n7 = event shown="[22] \"Start auto\": Value Change" {
          selector: _ -> [_ _ _ _ _ _ _ _ _ _ _ _ _ _ _ _ _ _ _ _ _ _ _ _ _ _]
          dyn-events: _ -> [_ _ _ _ _ _ _ _ _ _ _ _ _ _ _ _ _ _ _ _ _ _ _ _ _ _]
          timeout: -1 -> [_ _ _ _ _ _ _ _ _ _ _ _ _ _ _ _ _ _ _ _ _ _ _ _ _ _]
          tunnel: [_ TRUE _ _ _ _ _ _ _ FALSE _ _ _ _ _ _ _ _ _ _ _ _ _ _ _ _] -> w25
          tunnel: w24 -> [w29 w41 w51 w56 w61 w65 w70 w74 w81 w87 w92 w97 w102 w107 w112 w117 w122 w127 w132 w137 w142 w147 w152 w194 w199 w204]
          tunnel: [_ w45 w50 w55 w60 w64 w68 w73 _ w86 w91 w96 w100 w105 w110 w115 w120 w125 w130 w135 w141 w145 w151 w191 w196 w203] -> w23
          tunnel: w22 -> [w28 w44 w49 w54 w59 w63 w69 w75 w80 w84 w90 w95 w101 w106 w111 w116 w121 w126 w131 w136 w140 w146 w150 w193 w198 w202]
          tunnel: [w27 w43 w48 w53 _ w62 w67 w72 _ w85 w89 w94 w99 w104 w109 w114 w119 w124 w129 w134 w139 w144 w149 w192 w197 w201] -> w21
          tunnel: [_ _ _ _ _ _ _ _ w79 _ _ _ _ _ _ _ _ _ _ _ _ _ _ _ _ _] -> _
          tunnel: [_ _ _ _ _ _ _ _ w78 _ _ _ _ _ _ _ _ _ _ _ _ _ _ _ _ _] -> _
          tunnel: [w26 _ _ _ _ _ _ _ _ _ _ _ _ _ _ _ _ _ _ _ _ _ _ _ _ _] -> _
          tunnel: [_ _ _ _ w58 _ _ _ _ _ _ _ _ _ _ _ _ _ _ _ _ _ _ _ _ _] -> _
          event Timeout {
            n8 = event-data() -> ()  [unwired: 1 in, 2 out]
            n9 = First Call?() -> (First Call?: T/F=w30:bool)
            n10 = case shown="True" w30 {
              tunnel: w28 -> [w33 w39]
              tunnel: w29 -> [w35 w40]
              tunnel: [w32 w38] -> w27
              tunnel: [w34 w37] -> w26
              frame False {
                n11 = Enqueue Element(queue=w35, element="idle", error in (no error)=w33) -> (queue out=w34:refnum<queue>, error out=w32:errorcluster)  [unwired: 1 in, 1 out]
              }
              frame True {
                n12 = Enqueue Element(queue=w40, element="load file manual", error in (no error)=w39) -> (queue out=w37:refnum<queue>, error out=w38:errorcluster)  [unwired: 1 in, 1 out]
              }
            }
          }
          event "stop": Value Change {
            n13 = event-data() -> ()  [unwired: 1 in, 5 out]
            n14 = Enqueue Element(queue=w41, element="stop", error in (no error)=w44) -> (queue out=w45:refnum<queue>, error out=w43:errorcluster)  [unwired: 1 in, 1 out]
          }
          event "StartRaw": Value Change {
            n15 = event-data() -> ()  [unwired: 1 in, 5 out]
            n16 = Enqueue Element(queue=w51, element="start raw", error in (no error)=w49) -> (queue out=w50:refnum<queue>, error out=w48:errorcluster)  [unwired: 1 in, 1 out]
          }
          event "load file": Value Change {
            n17 = event-data() -> ()  [unwired: 1 in, 5 out]
            n18 = Enqueue Element(queue=w56, element="load file manual", error in (no error)=w54) -> (queue out=w55:refnum<queue>, error out=w53:errorcluster)  [unwired: 1 in, 1 out]
          }
          event "Die Number": Value Change {
            n19 = event-data() -> ()  [unwired: 1 in, 5 out]
            n20 = Enqueue Element(queue=w61, element="Die number picked", error in (no error)=w59) -> (queue out=w60:refnum<queue>, error out=w58:errorcluster)  [unwired: 1 in, 1 out]
          }
          event "Laser Current (mA)": Value Change {
            n21 = event-data() -> ()  [unwired: 1 in, 5 out]
            n22 = Enqueue Element(queue=w65, element="Update Laser", error in (no error)=w63) -> (queue out=w64:refnum<queue>, error out=w62:errorcluster)  [unwired: 1 in, 1 out]
          }
          event "Move to": Value Change {
            n23 = event-data() -> ()  [unwired: 1 in, 5 out]
            n24 = Enqueue Element(queue=w70, element="moveto", error in (no error)=w69) -> (queue out=w68:refnum<queue>, error out=w67:errorcluster)  [unwired: 1 in, 1 out]
          }
          event "Manual_Test": Value Change {
            n25 = event-data() -> ()  [unwired: 1 in, 5 out]
            n26 = Enqueue Element(queue=w74, element="manual test", error in (no error)=w75) -> (queue out=w73:refnum<queue>, error out=w72:errorcluster)  [unwired: 1 in, 1 out]
          }
          event "J set A/cm2": Value Change {
            n27 = event-data() -> ()  [unwired: 1 in, 5 out]
            n28 = Enqueue Element(queue=w81, element="Jset change", error in (no error)=w80) -> (queue out=w79:refnum<queue>, error out=w78:errorcluster)  [unwired: 1 in, 1 out]
          }
          event "Reset xy": Value Change {
            n29 = event-data() -> ()  [unwired: 1 in, 5 out]
            n30 = Enqueue Element(queue=w87, element="reset xy", error in (no error)=w84) -> (queue out=w86:refnum<queue>, error out=w85:errorcluster)  [unwired: 1 in, 1 out]
          }
          event "Reset 1st die": Value Change {
            n31 = event-data() -> ()  [unwired: 1 in, 5 out]
            n32 = Enqueue Element(queue=w92, element="reset to 1st die", error in (no error)=w90) -> (queue out=w91:refnum<queue>, error out=w89:errorcluster)  [unwired: 1 in, 1 out]
          }
          event "Manual IV settting": Value Change {
            n33 = event-data() -> ()  [unwired: 1 in, 5 out]
            n34 = Enqueue Element(queue=w97, element="change plot", error in (no error)=w95) -> (queue out=w96:refnum<queue>, error out=w94:errorcluster)  [unwired: 1 in, 1 out]
          }
          event "update wafer": Value Change {
            n35 = event-data() -> ()  [unwired: 1 in, 5 out]
            n36 = Enqueue Element(queue=w102, element="update wafer", error in (no error)=w101) -> (queue out=w100:refnum<queue>, error out=w99:errorcluster)  [unwired: 1 in, 1 out]
          }
          event "Select": Value Change {
            n37 = event-data() -> ()  [unwired: 1 in, 5 out]
            n38 = Enqueue Element(queue=w107, element="select", error in (no error)=w106) -> (queue out=w105:refnum<queue>, error out=w104:errorcluster)  [unwired: 1 in, 1 out]
          }
          event "StartFine": Value Change {
            n39 = event-data() -> ()  [unwired: 1 in, 5 out]
            n40 = Enqueue Element(queue=w112, element="start fine", error in (no error)=w111) -> (queue out=w110:refnum<queue>, error out=w109:errorcluster)  [unwired: 1 in, 1 out]
          }
          event "Mask File Raw": Value Change {
            n41 = event-data() -> ()  [unwired: 1 in, 5 out]
            n42 = Enqueue Element(queue=w117, element="raw mask updated", error in (no error)=w116) -> (queue out=w115:refnum<queue>, error out=w114:errorcluster)  [unwired: 1 in, 1 out]
          }
          event "Mask File Manual": Value Change {
            n43 = event-data() -> ()  [unwired: 1 in, 5 out]
            n44 = Enqueue Element(queue=w122, element="mask manual update", error in (no error)=w121) -> (queue out=w120:refnum<queue>, error out=w119:errorcluster)  [unwired: 1 in, 1 out]
          }
          event "Load raw": Value Change {
            n45 = event-data() -> ()  [unwired: 1 in, 5 out]
            n46 = Enqueue Element(queue=w127, element="load raw data", error in (no error)=w126) -> (queue out=w125:refnum<queue>, error out=w124:errorcluster)  [unwired: 1 in, 1 out]
          }
          event "Refresh Device": Value Change {
            n47 = event-data() -> ()  [unwired: 1 in, 5 out]
            n48 = Enqueue Element(queue=w132, element="refresh device names", error in (no error)=w131) -> (queue out=w130:refnum<queue>, error out=w129:errorcluster)  [unwired: 1 in, 1 out]
          }
          event "Add to list": Value Change {
            n49 = event-data() -> ()  [unwired: 1 in, 5 out]
            n50 = Enqueue Element(queue=w137, element="add to list", error in (no error)=w136) -> (queue out=w135:refnum<queue>, error out=w134:errorcluster)  [unwired: 1 in, 1 out]
          }
          event "Remove from List": Value Change {
            n51 = event-data() -> ()  [unwired: 1 in, 5 out]
            n52 = Enqueue Element(queue=w142, element="remove from list", error in (no error)=w140) -> (queue out=w141:refnum<queue>, error out=w139:errorcluster)  [unwired: 1 in, 1 out]
          }
          event "Clear List": Value Change {
            n53 = event-data() -> ()  [unwired: 1 in, 5 out]
            n54 = Enqueue Element(queue=w147, element="clear list", error in (no error)=w146) -> (queue out=w145:refnum<queue>, error out=w144:errorcluster)  [unwired: 1 in, 1 out]
          }
          event "Start auto": Value Change {
            n55 = event-data() -> ()  [unwired: 1 in, 1 out]
            n56 = property on="Test List" class="LstBox (strict)"() -> ("Item Names"=w148:string[])  [unwired: 2 in, 2 out]
            n57 = for {
              shift-right: [w157] -> w149
              shift-left: w150 -> [w161]
              shift-right: [w158] -> w151
              shift-left: w152 -> [w162]
              tunnel: w148 -> [_] mode=indexing
              n58 = Enqueue Element(queue=w162, element="pick device", error in (no error)=w161) -> (queue out=w160:refnum<queue>, error out=w159:errorcluster)  [unwired: 1 in, 1 out]
              n59 = case shown="False" FALSE {
                tunnel: w160 -> [w179 w189]
                tunnel: w159 -> [w177 w190]
                tunnel: [w188 w189] -> w156
                tunnel: [w187 w190] -> w155
                frame False {
                  n60 = Enqueue Element(queue=w179, element="Zero Laser", error in (no error)=w177) -> (queue out=w178:refnum<queue>, error out=w176:errorcluster)  [unwired: 1 in, 1 out]
                  n61 = Enqueue Element(queue=w178, element="Update Laser", error in (no error)=w176) -> (queue out=w182:refnum<queue>, error out=w181:errorcluster)  [unwired: 1 in, 1 out]
                  n62 = Enqueue Element(queue=w182, element="start raw", error in (no error)=w181) -> (queue out=w185:refnum<queue>, error out=w186:errorcluster)  [unwired: 1 in, 1 out]
                  n63 = Enqueue Element(queue=w185, element="select", error in (no error)=w186) -> (queue out=w188:refnum<queue>, error out=w187:errorcluster)  [unwired: 1 in, 1 out]
                }
                frame True {
                }
              }
              n64 = property on="Laser List" class="LstBox (strict)"() -> ("Item Names"=w154:string[])  [unwired: 2 in, 2 out]
              n65 = for {
                tunnel: [w173] -> w158
                tunnel: [w172] -> w157
                tunnel: w156 -> [w167]
                tunnel: w155 -> [w171]
                tunnel: w154 -> [_] mode=indexing
                n66 = Enqueue Element(queue=w167, element="pick laser", error in (no error)=w171) -> (queue out=w166:refnum<queue>, error out=w169:errorcluster)  [unwired: 1 in, 1 out]
                n67 = Enqueue Element(queue=w166, element="Update Laser", error in (no error)=w169) -> (queue out=w165:refnum<queue>, error out=w168:errorcluster)  [unwired: 1 in, 1 out]
                n68 = Enqueue Element(queue=w165, element="start fine", error in (no error)=w168) -> (queue out=w173:refnum<queue>, error out=w172:errorcluster)  [unwired: 1 in, 1 out]
              }
            }
          }
          event "Add to Laser": Value Change {
            n69 = event-data() -> ()  [unwired: 1 in, 5 out]
            n70 = Enqueue Element(queue=w194, element="add to laser list", error in (no error)=w193) -> (queue out=w191:refnum<queue>, error out=w192:errorcluster)  [unwired: 1 in, 1 out]
          }
          event "Remove from Laser List": Value Change {
            n71 = event-data() -> ()  [unwired: 1 in, 5 out]
            n72 = Enqueue Element(queue=w199, element="remove from laser list", error in (no error)=w198) -> (queue out=w196:refnum<queue>, error out=w197:errorcluster)  [unwired: 1 in, 1 out]
          }
          event "Clear Laser List": Value Change {
            n73 = event-data() -> ()  [unwired: 1 in, 5 out]
            n74 = Enqueue Element(queue=w204, element="clear laser list", error in (no error)=w202) -> (queue out=w203:refnum<queue>, error out=w201:errorcluster)  [unwired: 1 in, 1 out]
          }
        }
      }
      n75 = while {
        shift-right: [w213] -> _
        shift-left: w18 -> [w210]
        shift-right: [w212] -> _
        shift-left: w17 -> [w209]
        stop <- w215 stop-if-true
        n76 = Dequeue Element(queue=w210, error in (no error)=w209) -> (queue out=w208:refnum<queue>, element=w214:string, error out=w211:errorcluster)  [unwired: 1 in, 1 out]
        n77 = local read "Laser Current (mA)"() -> (w207:dbl)
        n78 = Greater Than 0?(x=w207) -> (x > 0?=w206:bool)
        n79 = case shown="\"start fine\"" w214 {
          tunnel: [FALSE TRUE FALSE FALSE FALSE FALSE FALSE FALSE FALSE FALSE FALSE FALSE FALSE FALSE FALSE FALSE FALSE FALSE FALSE FALSE FALSE FALSE FALSE FALSE FALSE FALSE FALSE FALSE FALSE] -> w215
          tunnel: w211 -> [w217 w220 w225 w387 w398 w409 w440 w464 w475 w505 w585 w595 w602 w617 w654 w692 w849 w877 w886 w897 w906 w914 w925 w928 w934 w940 w948 w956 w972]
          tunnel: [w217 w220 w226 w388 w395 w406 w443 w465 w478 w504 w590 w595 w601 w619 w656 w694 w849 w877 w888 w899 w908 w917 w925 w928 w934 w942 w951 w955 w972] -> w212
          tunnel: w208 -> [w216 w219 w228 w390 w397 w408 w441 w467 w480 w502 w592 w596 w600 w618 w655 w693 w850 w878 w887 w898 w907 w916 w926 w929 w935 w941 w950 w958 w973]
          tunnel: [w216 w219 w227 w389 w396 w407 w442 w466 w479 w503 w591 w596 w599 w620 w657 w695 w850 w878 w889 w900 w909 w918 w926 w929 w935 w943 w952 w957 w973] -> w213
          tunnel: w206 -> [_ _ _ _ _ _ _ _ _ _ _ _ _ _ _ w688 _ _ _ _ _ _ _ _ _ _ _ _ _]
          frame "False", Default {
          }
          frame "stop" {
          }
          frame "start raw" {
            n80 = flat-sequence {
              tunnel: [w240] -> w224
              tunnel: w224 -> [w270]
              tunnel: [w270] -> w223
              tunnel: [w260] -> w222
              tunnel: w223 -> [w272]
              tunnel: w222 -> [w271]
              frame #0 {
                n81 = local read "Wafer Name"() -> (w238:string)
                n82 = local read "RawTest ID"() -> (w243:u32)
                n83 = local write "Tab Control"(T12."Raw Test" ("Tab Control")) -> ()
                n84 = Increment(x=w243) -> (x+1=w242:u32)
                n85 = local read "Scribe"() -> (w237:string)
                n86 = local read "Mask"() -> (w236:string)
                n87 = call "Device Files v1.vi"("Rows"=1200, "Mask file path"="Mask File Raw") -> ("size(s)"=w240:i32, "Array of Cell Clusters"=→"Array of Cell Data Clusters":T3)  [unwired: 6 in, 2 out]
                "Total Device" <- w240
                n88 = local read "Lot"() -> (w235:string)
                n89 = local write "Status"("Prepare raw test" ("Status")) -> ()
                n90 = local write "RawTest ID"(w242) -> ()
                n91 = Bundle By Name(cluster="Wafer Info 2", "Wafer Name"=w238, "Scribe"=w237, "Mask"=w236, "Lot"=w235) -> (w239:T7)
                n92 = local write "Wafer Info"(w239) -> ()
                n93 = Initialize Array(nan ("element"), w240) -> (w233:dbl[])
                n94 = local write "I meas"(w233) -> ()
                n95 = local write "V meas"(w233) -> ()
                n96 = Bundle(w233, w233) -> (→"Selected Data":cluster{dbl[], dbl[]})  [unwired: 1 in]
                "Progress" <- u8 0 ("Progress")
              }
              frame #1 {
                n97 = local read "Wafer Name"() -> (w266:string)
                n98 = local read "J set A/cm2"() -> (w254:dbl)
                n99 = local read "RawTest ID"() -> (w250:u32)
                n100 = local read "Operator"() -> (w249:string)
                n101 = local read "RawData Save Path"() -> (w264:path)
                n102 = local read "Laser Current (mA)"() -> (w251:dbl)
                n103 = local read "Array of Cell Data Clusters"() -> (w269:T11)
                n104 = local read "V compliance"() -> (w252:dbl)
                n105 = local read "I compliance"() -> (w255:dbl)
                n106 = Index Array(array=w269, index=0) -> (element=w267:T14)
                n107 = Unbundle By Name(w267) -> ("Cell Name"=w265:string)
                n108 = call "get RawTest filename.vi"("Device Name"=w265, "Wafer Name"=w266) -> ("current time"=w257:timestamp, "FileName"=w263:string)  [unwired: 8 in]
                n109 = local write "Test FileName"(w263) -> ()
                n110 = local read "V set"() -> (w256:dbl)
                n111 = local read "I set"() -> (w253:dbl)
                n112 = Build Path(base path=w264, name or relative path=w263) -> (appended path=w262:path)
                n113 = Bundle By Name(cluster="Session Info 2", "V set"=w256, "I compliance"=w255, "J set"=w254, "I set"=w253, "V compliance"=w252, "Laser Power (mW)"=w251, "TestID"=w250, "Session Time"=w257, "Operator"=w249) -> (w258:T5)
                n114 = call "writeFile RawTestHead.vi"("Name Array"="Name Array", "Path"=w262) -> ("Path out"=w260:path)  [unwired: 9 in]
                "RawData file" <- w260
                n115 = local write "Session Info"(w258) -> ()
              }
              frame #2 {
                n116 = for {
                  N: w272 -> [w285]
                  tunnel: w271 -> [w273]
                  i -> [w274]
                  n117 = flat-sequence {
                    tunnel: [w320] -> w295
                    tunnel: [w319] -> w294
                    tunnel: w274 -> [w313]
                    tunnel: [w315] -> w289
                    tunnel: [w314] -> w288
                    tunnel: [w297] -> w287
                    tunnel: [w296] -> w286
                    tunnel: w295 -> [w321]
                    tunnel: w294 -> [w329]
                    tunnel: [w328] -> w293
                    tunnel: [w327] -> w292
                    tunnel: w289 -> [w325]
                    tunnel: w288 -> [w324]
                    tunnel: w287 -> [w323]
                    tunnel: w286 -> [w322]
                    tunnel: w293 -> [w332]
                    tunnel: w292 -> [w331]
                    tunnel: [w342] -> w291
                    tunnel: [w341] -> w290
                    tunnel: w291 -> [w345]
                    tunnel: w290 -> [w353]
                    tunnel: [w345] -> w276
                    tunnel: [w346] -> w275
                    tunnel: w276 -> [w364]
                    tunnel: w275 -> [w363]
                    tunnel: w274 -> [w370]
                    tunnel: w273 -> [w361]
                    frame #0 {
                      n118 = Increment(x=w313) -> (x+1=→"Current Device":i32)
                      n119 = local read "Prober GPIB"() -> (w311:string)
                      n120 = local read "J set A/cm2"() -> (w305:dbl)
                      n121 = local read "current y"() -> (w316:i32)
                      n122 = local read "current x"() -> (w318:i32)
                      n123 = local read "Laser Current (mA)"() -> (w309:dbl)
                      n124 = local read "Device Name"() -> (w300:string)
                      n125 = local read "Array of Cell Data Clusters"() -> (w317:T11)
                      n126 = call "EG2001 Move Z Down.vi"("GPIB Address"=w311) -> ("Error Out"=w319:errorcluster, "GPIB Address Out"=w320:string)  [unwired: 9 in]
                      n127 = Index Array(array=w317, index=w313) -> (element=w310:T14)
                      n128 = Unbundle By Name(w310) -> ("X-coord"=w297:dbl, "Y-coord"=w296:dbl, "Area"=w298:dbl, "Meas Area"=w299:dbl, "Cell Name"=w303:string)
                      n129 = call "get Area.vi"("Laser"=w309, "Cell Data Cluster"=w310) -> ("Area"=w307:dbl)  [unwired: 9 in]
                      n130 = local write "ActiveArea_um2"(w298) -> ()
                      n131 = local write "Device Name"(w303) -> ()
                      n132 = local write "MesaArea_um2"(w299) -> ()
                      n133 = Divide(x=w307, y=100000000.0) -> (x/y=w306:dbl)
                      n134 = Bundle By Name(cluster="Die Info 2", "Device Name"=w300, "ActiveArea_um2"=w298, "MesaArea_um2"=w299, "x"=w297, "y"=w296) -> (w301:T6)
                      n135 = Multiply(x=w305, y=w306) -> (x*y=w304:dbl)
                      n136 = local write "Die Info"(w301) -> ()
                      n137 = local write "I set"(w304) -> ()
                      n138 = Subtract(x=w296, y=w316) -> (x-y=w314:dbl)
                      n139 = Subtract(x=w297, y=w318) -> (x-y=w315:dbl)
                    }
                    frame #1 {
                      n140 = local write "current y"(w322) -> ()
                      n141 = local write "current x"(w323) -> ()
                      n142 = call "EG2001 Move Machine Step X-Y.vi"("Flip X Coordinates?"=FALSE, "Y"=w324, "Steps/Microns"=enum32{"Steps", "Microns"}."Microns", "X"=w325, "error in (no error)"=w329, "GPIB Address"=w321) -> ("Error Out"=w327:errorcluster, "GPIB Address Out"=w328:string)  [unwired: 4 in]
                    }
                    frame #2 {
                      n143 = call "EG2001 Move Z Up.vi"("error in (no error)"=w331, "GPIB Address"=w332) -> ()  [unwired: 10 out]
                    }
                    frame #3 {
                      n144 = local read "Id delay ms"() -> (w335:dbl)
                      n145 = local read "Repeat Id"() -> (w336:u32)
                      n146 = local read "Channel"() -> (w339:enum32{"Channel A", "Channel B"})
                      n147 = local read "Imeas Settings"() -> (w340:T10)
                      n148 = local read "I compliance"() -> (w337:dbl)
                      n149 = local read "NPLC"() -> (w338:dbl)
                      n150 = local read "V set"() -> (w333:dbl)
                      n151 = Bundle By Name(cluster=w340, "Channel"=w339, "Vset"=w333, "NPLC"=w338, "I compliance"=w337, "Repeat time"=w336, "Delay ms"=w335) -> (w334:T10)
                      n152 = local read "SMU"() -> (w341:refnum<visa-resource-name>)
                      n153 = call "K2602 setVmeasI.vi"("Settings"=w334, "SMU"=w341) -> ("Iavg"=w342:dbl)  [unwired: 6 in, 3 out]
                    }
                    frame #4 {
                      n154 = local read "Vf delay ms"() -> (w347:dbl)
                      n155 = local read "Repeat Vf"() -> (w348:u32)
                      n156 = local read "Channel"() -> (w350:enum32{"Channel A", "Channel B"})
                      n157 = local read "Vmeas Settings"() -> (w352:T9)
                      n158 = local read "V compliance"() -> (w349:dbl)
                      n159 = local read "NPLC"() -> (w344:dbl)
                      n160 = local read "I set"() -> (w343:dbl)
                      n161 = Bundle By Name(cluster=w352, "Channel"=w350, "Iset"=w343, "NPLC"=w344, "V compliance"=w349, "Repeat time"=w348, "Delay ms"=w347) -> (w351:T9)
                      n162 = call "K2602 setImeasV.vi"("Settings"=w351, "SMU"=w353) -> ("Vavg"=w346:dbl)  [unwired: 6 in, 3 out]
                    }
                    frame #5 {
                      n163 = local read "Session Info"() -> (w357:T5)
                      n164 = local read "Wafer Info"() -> (w359:T7)
                      n165 = local read "Die Info"() -> (w358:T6)
                      n166 = local read "V meas"() -> (w371:dbl[])
                      n167 = local read "I meas"() -> (w372:dbl[])
                      n168 = local read "Selected Data"() -> (w355:cluster{dbl[], dbl[]})
                      n169 = Replace Array Subset(array=w372, new element=w364, index=w370) -> (w367:dbl[])
                      n170 = Replace Array Subset(array=w371, new element=w363, index=w370) -> (w366:dbl[])
                      n171 = Get Date/Time In Seconds() -> (seconds since 1Jan1904=w362:timestamp)
                      n172 = local write "I meas"(w367) -> ()
                      n173 = local write "V meas"(w366) -> ()
                      n174 = Bundle By Name(cluster="Test Results 2", "I meas"=w364, "V meas"=w363, "Time"=w362) -> (w360:T4)
                      n175 = call <vilib>:"Histogram.vi"("X"=w366) -> ("Histogram Graph"=→"Vforward hist":T13)  [unwired: 7 in, 3 out]
                      n176 = call "writeFile RawTestData.vi"("Test Results"=w360, "Session Info"=w357, "Die Info"=w358, "Wafer Info"=w359, "Path"=w361) -> ()  [unwired: 6 in, 1 out]
                      n177 = local write "Test Results"(w360) -> ()
                      n178 = Bundle("V meas"=w366, "I meas"=w367) -> (w356:cluster{"V meas":dbl[], "I meas":dbl[]})  [unwired: 1 in]
                      n179 = call <vilib>:"Histogram.vi"("X"=w367) -> ("Histogram Graph"=→"Idark hist":T13)  [unwired: 7 in, 3 out]
                      n180 = Build Array(w356, w355) -> (→"Spec Plot":cluster{"V meas":dbl[], "I meas":dbl[]}[])
                    }
                  }
                  n181 = Divide(x=w274, y=w285) -> (x/y=w283:dbl)
                  n182 = Increment(x=w274) -> (x+1=w277:i32)
                  n183 = Number To Decimal String(number=w277) -> (decimal integer string=w279:string)  [unwired: 1 in]
                  n184 = Multiply(x=w283, y=100.0) -> (x*y=w281:dbl)
                  n185 = To Unsigned Byte Integer(number=w281) -> (unsigned 8bit integer=w284:u8)
                  n186 = local write "Progress"(w284) -> ()
                  n187 = Concatenate Strings("Raw Test for die number:" ("string"), w279) -> (w280:string)
                  n188 = local write "Status"(w280) -> ()
                }
              }
              frame #3 {
                w377 = -1
                n189 = local read "Prober GPIB"() -> (w384:string)
                n190 = local read "RawTest ID"() -> (w374:u32)
                n191 = local read "TestID file"() -> (w373:path)
                n192 = local read "current y"() -> (w378:i32)
                n193 = local read "current x"() -> (w379:i32)
                n194 = Multiply(x=w377, y=w378) -> (x*y=w375:i32)
                n195 = Multiply(x=w377, y=w379) -> (x*y=w376:i32)
                n196 = call "writeFile TestID.vi"("TestID"=w374, "Path"=w373) -> ()  [unwired: 10 in]
                n197 = call "EG2001 Move Z Down.vi"("GPIB Address"=w384) -> ("Error Out"=w383:errorcluster, "GPIB Address Out"=w382:string)  [unwired: 9 in]
                n198 = call "EG2001 Move Machine Step X-Y.vi"("Flip X Coordinates?"=FALSE, "Y"=w375, "Steps/Microns"=enum32{"Steps", "Microns"}."Microns", "X"=w376, "error in (no error)"=w383, "GPIB Address"=w382) -> ()  [unwired: 4 in, 2 out]
              }
              frame #4 {
                w385 = 0
                n199 = local write "current y"(w385) -> ()
                n200 = local write "current x"(w385) -> ()
              }
            }
            n201 = Enqueue Element At Opposite End(queue=w228, element="idle", error in (no error)=w225) -> (queue out=w227:refnum<queue>, error out=w226:errorcluster)  [unwired: 1 in, 1 out]
          }
          frame "reset xy" {
            n202 = local read "Prober GPIB"() -> (w386:string)
            n203 = Enqueue Element At Opposite End(queue=w390, element="idle", error in (no error)=w387) -> (queue out=w389:refnum<queue>, error out=w388:errorcluster)  [unwired: 1 in, 1 out]
            n204 = call "EG2001 Move First.vi"("GPIB Address"=w386) -> ()  [unwired: 9 in, 2 out]
            "current x" <- u32 0 ("current x")
            "current y" <- u32 0 ("current y")
          }
          frame "reset to 1st die" {
            n205 = Enqueue Element At Opposite End(queue=w397, element="idle", error in (no error)=w398) -> (queue out=w396:refnum<queue>, error out=w395:errorcluster)  [unwired: 1 in, 1 out]
            n206 = local read "Array of Cell Data Clusters"() -> (w404:T11)
            n207 = Index Array(array=w404, index=0) -> (element=w402:T14)
            n208 = Unbundle By Name(w402) -> ("X-coord"=w401:dbl, "Y-coord"=w400:dbl)
            n209 = local write "current x"(w401) -> ()
            n210 = local write "current y"(w400) -> ()
          }
          frame "load file manual" {
            n211 = flat-sequence {
              tunnel: [w416] -> w411
              tunnel: w411 -> [w420]
              frame #0 {
                n212 = local write "Status"("Loading mask file" ("Status")) -> ()
                n213 = call "Device Files v1.vi"("Rows"=1200, "Mask file path"="Mask File Manual") -> ("Mask Name"=w417:string, "size(s)"=w416:i32, "Array of Cell Clusters"=w413:T3)  [unwired: 6 in, 1 out]
                n214 = local write "Mask"(w417) -> ()
                n215 = local write "Array of Cell Data Clusters"(w413) -> ()
              }
              frame #1 {
                n216 = for {
                  N: w420 -> [_]
                  tunnel: [w421] -> w419 mode=indexing
                  i -> [w422]
                  n217 = Number To Decimal String(number=w422) -> (decimal integer string=w421:string)  [unwired: 1 in]
                }
                n218 = property on="Die Number" class="Ring (strict)"("Strings []"=w419) -> ()  [unwired: 2 in, 2 out]
              }
              frame #2 {
                n219 = local read "Die Number"() -> (w429:u16)
                n220 = local read "Array of Cell Data Clusters"() -> (w430:T11)
                n221 = Index Array(array=w430, index=w429) -> (element=w428:T14)
                n222 = Unbundle By Name(w428) -> ("Cell Name"=w423:string, "X-coord"=w426:dbl, "Y-coord"=w427:dbl, "Area"=w425:dbl, "Meas Area"=w424:dbl)
                n223 = local write "Device Name"(w423) -> ()
                n224 = local write "x target"(w426) -> ()
                n225 = local write "y target"(w427) -> ()
                n226 = local write "ActiveArea_um2"(w425) -> ()
                n227 = local write "MesaArea_um2"(w424) -> ()
              }
              frame #3 {
                n228 = local read "J set A/cm2"() -> (w436:dbl)
                n229 = local read "Laser Current (mA)"() -> (w433:dbl)
                n230 = Equal To 0?(x=w433) -> (x = 0?=w432:bool)
                n231 = case shown="True" w432 {
                  tunnel: [w438 w439] -> w431
                  frame False {
                    n232 = local read "ActiveArea_um2"() -> (w438:dbl)
                  }
                  frame True {
                    n233 = local read "MesaArea_um2"() -> (w439:dbl)
                  }
                }
                n234 = Divide(x=w431, y=100000000.0) -> (x/y=w435:dbl)
                n235 = Multiply(x=w435, y=w436) -> (x*y=w437:dbl)
                n236 = local write "I set"(w437) -> ()
              }
            }
            n237 = Enqueue Element At Opposite End(queue=w408, element="idle", error in (no error)=w409) -> (queue out=w407:refnum<queue>, error out=w406:errorcluster)  [unwired: 1 in, 1 out]
          }
          frame "Die number picked" {
            n238 = flat-sequence {
              frame #0 {
                n239 = local read "Die Number"() -> (w453:u16)
                n240 = local read "Array of Cell Data Clusters"() -> (w454:T11)
                n241 = Index Array(array=w454, index=w453) -> (element=w452:T14)
                n242 = Unbundle By Name(w452) -> ("Cell Name"=w449:string, "X-coord"=w451:dbl, "Y-coord"=w450:dbl, "Area"=w448:dbl, "Meas Area"=w447:dbl)
                n243 = local write "Device Name"(w449) -> ()
                n244 = local write "x target"(w451) -> ()
                n245 = local write "y target"(w450) -> ()
                n246 = local write "ActiveArea_um2"(w448) -> ()
                n247 = local write "MesaArea_um2"(w447) -> ()
              }
              frame #1 {
                n248 = local read "J set A/cm2"() -> (w460:dbl)
                n249 = local read "Laser Current (mA)"() -> (w457:dbl)
                n250 = Equal To 0?(x=w457) -> (x = 0?=w456:bool)
                n251 = case shown="True" w456 {
                  tunnel: [w462 w463] -> w455
                  frame False {
                    n252 = local read "ActiveArea_um2"() -> (w462:dbl)
                  }
                  frame True {
                    n253 = local read "MesaArea_um2"() -> (w463:dbl)
                  }
                }
                n254 = Divide(x=w455, y=100000000.0) -> (x/y=w459:dbl)
                n255 = Multiply(x=w459, y=w460) -> (x*y=w461:dbl)
                n256 = local write "I set"(w461) -> ()
              }
            }
            n257 = Enqueue Element At Opposite End(queue=w441, element="idle", error in (no error)=w440) -> (queue out=w442:refnum<queue>, error out=w443:errorcluster)  [unwired: 1 in, 1 out]
            n258 = local write "Status"("Changing Die" ("Status")) -> ()
          }
          frame "Jset change" {
            n259 = local read "J set A/cm2"() -> (w470:dbl)
            n260 = Enqueue Element At Opposite End(queue=w467, element="idle", error in (no error)=w464) -> (queue out=w466:refnum<queue>, error out=w465:errorcluster)  [unwired: 1 in, 1 out]
            n261 = local read "ActiveArea_um2"() -> (w473:dbl)
            n262 = Divide(x=w473, y=100000000.0) -> (x/y=w471:dbl)
            n263 = Multiply(x=w471, y=w470) -> (x*y=w469:dbl)
            n264 = local write "I set"(w469) -> ()
          }
          frame "moveto" {
            n265 = flat-sequence {
              tunnel: [w486] -> w477
              tunnel: [w485] -> w476
              tunnel: w477 -> [w491]
              tunnel: w476 -> [w490]
              frame #0 {
                n266 = local read "Prober GPIB"() -> (w484:string)
                n267 = local write "Status"("Probe up" ("Status")) -> ()
                n268 = call "EG2001 Move Z Down.vi"("GPIB Address"=w484) -> ("Error Out"=w485:errorcluster, "GPIB Address Out"=w486:string)  [unwired: 9 in]
              }
              frame #1 {
                n269 = local read "current y"() -> (w494:i32)
                n270 = local read "current x"() -> (w496:i32)
                n271 = local read "y target"() -> (w495:i32)
                n272 = local read "x target"() -> (w497:i32)
                n273 = local write "Status"("Moving Probe" ("Status")) -> ()
                n274 = Subtract(x=w495, y=w494) -> (x-y=w492:i32)
                n275 = Subtract(x=w497, y=w496) -> (x-y=w493:i32)
                n276 = call "EG2001 Move Machine Step X-Y.vi"("Flip X Coordinates?"=FALSE, "Y"=w492, "Steps/Microns"=enum32{"Steps", "Microns"}."Microns", "X"=w493, "error in (no error)"=w490, "GPIB Address"=w491) -> ()  [unwired: 4 in, 2 out]
              }
              frame #2 {
                n277 = local read "y target"() -> (w499:i32)
                n278 = local read "x target"() -> (w500:i32)
                n279 = local write "Status"("Done" ("Status")) -> ()
                n280 = local write "current x"(w500) -> ()
                n281 = local write "current y"(w499) -> ()
              }
            }
            n282 = Enqueue Element At Opposite End(queue=w480, element="idle", error in (no error)=w475) -> (queue out=w479:refnum<queue>, error out=w478:errorcluster)  [unwired: 1 in, 1 out]
          }
          frame "manual test" {
            n283 = flat-sequence {
              tunnel: [w518] -> w515
              tunnel: [w517] -> w514
              tunnel: [w523] -> w513
              tunnel: [w522] -> w512
              tunnel: w515 -> [w522]
              tunnel: [w521] -> w511
              tunnel: w514 -> [w521]
              tunnel: w513 -> [w547]
              tunnel: [w547] -> w510
              tunnel: [w537] -> w509
              tunnel: w512 -> [w537]
              tunnel: [w536] -> w508
              tunnel: w511 -> [w536]
              tunnel: w510 -> [w560]
              tunnel: [w550] -> w507
              tunnel: w509 -> [w550]
              tunnel: [w549] -> w506
              tunnel: w508 -> [w549]
              tunnel: w507 -> [w574]
              tunnel: w506 -> [w573]
              frame #0 {
                n284 = local read "Prober GPIB"() -> (w519:string)
                n285 = call "EG2001 Move Z Up.vi"("GPIB Address"=w519) -> ("Error Out"=w517:errorcluster, "GPIB Address Out"=w518:string)  [unwired: 1 in, 8 out]
              }
              frame #1 {
                n286 = local read "Channel"() -> (w533:enum32{"Channel A", "Channel B"})
                n287 = local read "sweep delay ms"() -> (w527:dbl)
                n288 = local read "Sweep Settings"() -> (w534:T8)
                n289 = local read "I compliance"() -> (w528:dbl)
                n290 = local write "Status"("Sweeping IV Curve") -> ()
                n291 = local read "V start"() -> (w532:dbl)
                n292 = local read "points"() -> (w530:u16)
                n293 = local read "V end"() -> (w531:dbl)
                n294 = local read "NPLC"() -> (w529:dbl)
                n295 = Bundle By Name(cluster=w534, "Channel"=w533, "Vstart"=w532, "Vend"=w531, "# of points"=w530, "NPLC"=w529, "I compliance"=w528, "Delay ms"=w527) -> (w526:T8)
                n296 = local read "SMU"() -> (w523:refnum<visa-resource-name>)
                n297 = call "K2602 Vsweep.vi"("Settings"=w526, "SMU"=w523) -> ("V"=→"Varray manual":dbl[], "I"=→"Iarray manual":dbl[])  [unwired: 7 in, 1 out]
              }
              frame #2 {
                n298 = local read "Id delay ms"() -> (w538:dbl)
                n299 = local read "Repeat Id"() -> (w539:u32)
                n300 = local read "Channel"() -> (w543:enum32{"Channel A", "Channel B"})
                n301 = local read "Imeas Settings"() -> (w546:T10)
                n302 = local read "I compliance"() -> (w540:dbl)
                n303 = local write "Status"("Measuring I @ Vset") -> ()
                n304 = local read "NPLC"() -> (w541:dbl)
                n305 = local read "V set"() -> (w542:dbl)
                n306 = Bundle By Name(cluster=w546, "Channel"=w543, "Vset"=w542, "NPLC"=w541, "I compliance"=w540, "Repeat time"=w539, "Delay ms"=w538) -> (w545:T10)
                n307 = call "K2602 setVmeasI.vi"("Settings"=w545, "SMU"=w547) -> ("Iavg"=w544:dbl)  [unwired: 6 in, 3 out]
                n308 = local write "Imeas manual"(w544) -> ()
              }
              frame #3 {
                n309 = local read "Vf delay ms"() -> (w551:dbl)
                n310 = local read "Repeat Vf"() -> (w552:u32)
                n311 = local read "Channel"() -> (w556:enum32{"Channel A", "Channel B"})
                n312 = local read "Vmeas Settings"() -> (w558:T9)
                n313 = local read "V compliance"() -> (w553:dbl)
                n314 = local write "Status"("Measuring V @ Iset") -> ()
                n315 = local read "NPLC"() -> (w554:dbl)
                n316 = local read "I set"() -> (w555:dbl)
                n317 = Bundle By Name(cluster=w558, "Channel"=w556, "Iset"=w555, "NPLC"=w554, "V compliance"=w553, "Repeat time"=w552, "Delay ms"=w551) -> (w557:T9)
                n318 = call "K2602 setImeasV.vi"("Settings"=w557, "SMU"=w560) -> ("Vavg"=w559:dbl)  [unwired: 6 in, 3 out]
                n319 = local write "Vmeas manual"(w559) -> ()
              }
              frame #4 {
                n320 = call "EG2001 Move Z Down.vi"("error in (no error)"=w573, "GPIB Address"=w574) -> ()  [unwired: 8 in, 2 out]
                n321 = local write "Status"("Done") -> ()
                n322 = local read "Manual IV settting"() -> (w572:enum32{"Linear plot", "Log plot"})
                n323 = local read "Vmeas manual"() -> (w564:dbl)
                n324 = local read "Varray manual"() -> (w566:dbl[])
                n325 = local read "Imeas manual"() -> (w563:dbl)
                n326 = local read "Iarray manual"() -> (w565:dbl[])
                n327 = local read "points"() -> (w567:u16)
                n328 = local read "V set"() -> (w562:dbl)
                n329 = local read "I set"() -> (w561:dbl)
                n330 = call "get Plot.vi"("I set"=w561, "Imeas"=w563, "V set"=w562, "Vmeas"=w564, "Iarray"=w565, "Varray"=w566, "points"=w567) -> ("logplot"=w569:cluster{"Varray manual":dbl[], dbl[]}[], "Linearplot"=w568:T15)  [unwired: 3 in]
                "Manual Plot 0" <- w568
                "Manaul Plot 1" <- w569
                n331 = case shown="\"Linear plot\", Default" w572 {
                  tunnel: w568 -> [w577 _]
                  tunnel: [w577 w580] -> w571
                  tunnel: w569 -> [_ w580]
                  frame "Linear plot", Default {
                    n332 = property on="Manual IV" class="XYGraph (strict)"("YScale.Mapping Mode"=u8 0 ("Y Scale.Mapping Mode")) -> ()  [unwired: 2 in, 2 out]
                    n333 = property on="Manual IV" class="XYGraph (strict)"("YScale.NameLbl.Text"="Current (A)" ("X Scale.Name Label.Text")) -> ()  [unwired: 2 in, 2 out]
                  }
                  frame "Log plot" {
                    n334 = property on="Manual IV" class="XYGraph (strict)"("YScale.NameLbl.Text"="Abs(I)" ("Y Scale.Name Label.Text")) -> ()  [unwired: 2 in, 2 out]
                    n335 = property on="Manual IV" class="XYGraph (strict)"("YScale.Mapping Mode"=u8 1 ("Y Scale.Mapping Mode")) -> ()  [unwired: 2 in, 2 out]
                  }
                }
                "Manual IV" <- w571
              }
            }
            n336 = Enqueue Element At Opposite End(queue=w502, element="idle", error in (no error)=w505) -> (queue out=w503:refnum<queue>, error out=w504:errorcluster)  [unwired: 1 in, 1 out]
          }
          frame "update wafer" {
            n337 = local read "Wafer Name"() -> (w583:string)
            n338 = Enqueue Element At Opposite End(queue=w592, element="idle", error in (no error)=w585) -> (queue out=w591:refnum<queue>, error out=w590:errorcluster)  [unwired: 1 in, 1 out]
            n339 = call "getDB Wafer Info.vi"("Wafer Name"=w583) -> ("WaferInfo"=w584:T16)  [unwired: 9 in, 1 out]
            n340 = Unbundle By Name(w584) -> ("WaferName"=w581:string, "Scribe"=w589:string, "Lot"=w588:string, "Mask"=w587:string)  [unwired: 1 out]
            n341 = local write "Scribe"(w589) -> ()
            n342 = local write "Lot"(w588) -> ()
            n343 = local write "Mask"(w587) -> ()
            n344 = Equal?(x=w583, y=w581) -> (x = y?=w582:bool)
            n345 = case shown="False" w582 {
              tunnel: w581 -> [w594 _]
              frame False {
                n346 = local write "Wafer Name"(w594) -> ()
              }
              frame True {
              }
            }
          }
          frame "idle" {
            n347 = local write "Status"("idle" ("Status")) -> ()
          }
          frame "change plot" {
            n348 = Enqueue Element At Opposite End(queue=w600, element="idle", error in (no error)=w602) -> (queue out=w599:refnum<queue>, error out=w601:errorcluster)  [unwired: 1 in, 1 out]
            n349 = local read "Manual IV settting"() -> (w606:enum32{"Linear plot", "Log plot"})
            n350 = case shown="\"Log plot\"" w606 {
              tunnel: [w609 w612] -> w605
              frame "Linear plot", Default {
                n351 = property on="Manual IV" class="XYGraph (strict)"("YScale.Mapping Mode"=u8 0 ("Y Scale.Mapping Mode")) -> ()  [unwired: 2 in, 2 out]
                n352 = local read "Manual Plot 0"() -> (w609:cluster{"V manual":dbl[], "I manual":dbl[]}[])
                n353 = property on="Manual IV" class="XYGraph (strict)"("YScale.NameLbl.Text"="Current (A)" ("Y Scale.Name Label.Text")) -> ()  [unwired: 2 in, 2 out]
              }
              frame "Log plot" {
                n354 = property on="Manual IV" class="XYGraph (strict)"("YScale.Mapping Mode"=u8 1 ("Y Scale.Mapping Mode")) -> ()  [unwired: 2 in, 2 out]
                n355 = property on="Manual IV" class="XYGraph (strict)"("YScale.NameLbl.Text"="Abs(I)" ("Y Scale.Name Label.Text")) -> ()  [unwired: 2 in, 2 out]
                n356 = local read "Manaul Plot 1"() -> (w612:cluster{"V manual":dbl[], dbl[]}[])
              }
            }
            n357 = local write "Manual IV"(w605) -> ()
          }
          frame "select" {
            n358 = local read "I meas"() -> (w615:dbl[])
            n359 = Enqueue Element At Opposite End(queue=w618, element="idle", error in (no error)=w617) -> (queue out=w620:refnum<queue>, error out=w619:errorcluster)  [unwired: 1 in, 1 out]
            n360 = Array Size(array=w615) -> (size(s)=w613:i32)
            n361 = Greater Than 0?(x=w613) -> (x > 0?=w614:bool)
            n362 = case shown="True" w614 {
              tunnel: w613 -> [_ w639]
              frame False {
              }
              frame True {
                n363 = Initialize Array(nan ("element"), w639) -> (w635:dbl[])
                n364 = local read "Wafer Name"() -> (w647:string)
                n365 = local read "RawData file"() -> (w626:path)
                n366 = local read "V meas"() -> (w631:dbl[])
                n367 = local read "I meas"() -> (w630:dbl[])
                n368 = local read "RawData Save Path"() -> (w641:path)
                n369 = local read "Laser Current (mA)"() -> (w623:dbl)
                n370 = local read "Number Select"() -> (w645:u16)
                n371 = local read "Mask File Raw"() -> (w646:path)
                n372 = Bundle("V meas"=w631, "I meas"=w630) -> (w629:cluster{"V meas":dbl[], "I meas":dbl[]})  [unwired: 1 in]
                n373 = Greater Than 0?(x=w623) -> (x > 0?=w622:bool)
                n374 = local read "Vmax"() -> (w644:dbl)
                n375 = local read "Vmin"() -> (w643:dbl)
                n376 = call "select RawTestData.vi"("Light > 0?"=w622, "Number Select"=w645, "Vmax"=w644, "Vmin"=w643, "V meas"=w631, "I meas"=w630) -> ("Selected V"=w638:dbl[], "Selected I"=w636:dbl[], "Selected Index"=w624:dbl[])  [unwired: 2 in, 1 out]
                n377 = call "save FineMask.vi"("Selected Index"=w624, "RawData Save Path"=w641, "Text Add"=w647, "Mask File Raw"=w646) -> ("Output path"=w642:path)  [unwired: 7 in]
                n378 = call "updatedFile RawTestSelect.vi"("Column Number"=u32 21, "Selected Index"=w624, "Path"=w626) -> ()  [unwired: 9 in]
                n379 = local write "Mask File Fine"(w642) -> ()
                n380 = Replace Array Subset(array=w635, new element=w638, index=0) -> (w633:dbl[])
                n381 = Replace Array Subset(array=w635, new element=w636, index=0) -> (w632:dbl[])
                n382 = Bundle(w633, w632) -> (w628:cluster{dbl[], dbl[]})  [unwired: 1 in]
                n383 = Build Array(w629, w628) -> (w627:cluster{"V meas":dbl[], "I meas":dbl[]}[])
                n384 = local write "Spec Plot"(w627) -> ()
              }
            }
          }
          frame "load raw data" {
            n385 = local read "RawData Save Path"() -> (w650:path)
            n386 = Enqueue Element At Opposite End(queue=w655, element="idle", error in (no error)=w654) -> (queue out=w657:refnum<queue>, error out=w656:errorcluster)  [unwired: 1 in, 1 out]
            n387 = call "File Dialog"("start path"=w650, "prompt"="Please pick a raw test data file", "pattern (all files)"="*.csv" ("pattern label")) -> ("selected path"=w649:path, "cancelled"=w653:bool)  [unwired: 9 in, 2 out]
            n388 = case shown="False" w653 {
              tunnel: w649 -> [_ w659]
              frame True {
              }
              frame False {
                n389 = local write "RawData file"(w659) -> ()
                n390 = Strip Path(path=w659) -> (name=w660:string)  [unwired: 1 out]
                n391 = call "read Raw.vi"("Path"=w659) -> ("Session Info"=w678:T17, "Die Info"=w687:T18, "Wafer Info"=w686:T7, "V"=w664:dbl[], "I"=w663:dbl[])  [unwired: 6 in]
                n392 = local write "I meas"(w663) -> ()
                n393 = local write "Test FileName"(w660) -> ()
                n394 = local write "V meas"(w664) -> ()
                n395 = Unbundle By Name(w678) -> ("V set"=w677:dbl, "I compliance"=w676:dbl, "J set"=w675:dbl, "I set"=w674:dbl, "V compliance"=w673:dbl, "Laser Power (mW)"=w671:dbl, "Operator"=w672:string)
                n396 = Unbundle By Name(w687) -> ("Device Name"=w681:string, "ActiveArea_um2"=w680:dbl, "MesaArea_um2"=w679:dbl)
                n397 = Unbundle By Name(w686) -> ("Wafer Name"=w685:string, "Scribe"=w684:string, "Mask"=w683:string, "Lot"=w682:string)
                n398 = Array Size(array=w663) -> (size(s)=w669:i32)
                n399 = Bundle("V"=w664, "I"=w663) -> (w667:cluster{"V":dbl[], "I":dbl[]})  [unwired: 1 in]
                n400 = call <vilib>:"Histogram.vi"("X"=w664) -> ("Histogram Graph"=w661:T13)  [unwired: 7 in, 3 out]
                n401 = call <vilib>:"Histogram.vi"("X"=w663) -> ("Histogram Graph"=w662:T13)  [unwired: 7 in, 3 out]
                n402 = local write "Vforward hist"(w661) -> ()
                n403 = local write "Scribe"(w684) -> ()
                n404 = local write "Mask"(w683) -> ()
                n405 = local write "Lot"(w682) -> ()
                n406 = local write "Idark hist"(w662) -> ()
                n407 = local write "Device Name"(w681) -> ()
                n408 = local write "MesaArea_um2"(w679) -> ()
                n409 = local write "V set"(w677) -> ()
                n410 = local write "ActiveArea_um2"(w680) -> ()
                n411 = local write "I set"(w674) -> ()
                n412 = Initialize Array(nan ("element"), w669) -> (w668:dbl[])
                n413 = local write "Laser Current (mA)"(w671) -> ()
                n414 = local write "Wafer Name"(w685) -> ()
                n415 = local write "Operator"(w672) -> ()
                n416 = local write "I compliance"(w676) -> ()
                n417 = local write "J set A/cm2"(w675) -> ()
                n418 = local write "V compliance"(w673) -> ()
                n419 = Bundle(w668, w668) -> (w666:cluster{dbl[], dbl[]})  [unwired: 1 in]
                n420 = local write "Selected Data"(w666) -> ()
                n421 = Build Array(w667, w666) -> (w665:cluster{"V":dbl[], "I":dbl[]}[])
                n422 = local write "Spec Plot"(w665) -> ()
              }
            }
          }
          frame "start fine" {
            n423 = flat-sequence {
              tunnel: [w700] -> w690
              tunnel: w688 -> [w698]
              tunnel: w690 -> [w716]
              frame #0 {
                w701 = u8 0 ("Progress 2")
                n424 = local read "points"() -> (w703:u16)
                n425 = local write "Progress 2"(w701) -> ()
                n426 = Initialize Array(nan ("element"), w703) -> (w705:dbl[])
                n427 = local write "Tab Control"(T12."Fine Test" ("Tab Control")) -> ()
                n428 = case shown="True" w698 {
                  tunnel: "Mask File Fine" -> [w710 _]
                  tunnel: [w710 w715] -> w696
                  frame False {
                  }
                  frame True {
                    n429 = local read "Wafer Name"() -> (w714:string)
                    n430 = local read "RawData Save Path"() -> (w712:path)
                    n431 = local read "Device Name"() -> (w713:string)
                    n432 = call "Find Latest Fine Mask File.vi"("RawData Save Path"=w712, "Device Name"=w713, "Wafer Name"=w714) -> ("Error Out"=w711:errorcluster, "Mask File Fine"=w715:path)  [unwired: 7 in]
                    n433 = local write "error out"(w711) -> ()
                  }
                }
                n434 = local write "Status"("prepare fine test" ("Status")) -> ()
                n435 = Bundle(w705, w705) -> (w704:cluster{dbl[], dbl[]})  [unwired: 1 in]
                n436 = local write "Mask File Fine"(w696) -> ()
                n437 = call "Device Files v1.vi"("Rows"=1200, "Mask file path"=w696) -> ("size(s)"=w700:i32, "Array of Cell Clusters"=→"Fine Cell Clusters":T3)  [unwired: 6 in, 2 out]
                "Total Device" <- w700
                n438 = Initialize Array(w704, w700) -> (→"IV fine linear" →"IV fine log":cluster{dbl[], dbl[]}[])
                "Current Device" <- w701
              }
              frame #1 {
                n439 = for {
                  N: w716 -> [w740]
                  i -> [w741]
                  n440 = flat-sequence {
                    tunnel: w741 -> [w756]
                    tunnel: [w764] -> w735
                    tunnel: [w763] -> w734
                    tunnel: [w760] -> w733
                    tunnel: [w759] -> w732
                    tunnel: [w758] -> w731
                    tunnel: [w757] -> w730
                    tunnel: [w756] -> w721
                    tunnel: w735 -> [w779]
                    tunnel: w734 -> [w778]
                    tunnel: w733 -> [w776]
                    tunnel: w732 -> [w775]
                    tunnel: w731 -> [w774]
                    tunnel: w730 -> [w773]
                    tunnel: [w772] -> w729
                    tunnel: [w771] -> w728
                    tunnel: [w770] -> w722
                    tunnel: w721 -> [w770]
                    tunnel: w729 -> [w782]
                    tunnel: w728 -> [w781]
                    tunnel: [w780] -> w723
                    tunnel: w722 -> [w780]
                    tunnel: [w786] -> w724
                    tunnel: w723 -> [w786]
                    tunnel: w724 -> [w816]
                    tunnel: [w806] -> w719
                    tunnel: [w800] -> w718
                    tunnel: [w799] -> w717
                    tunnel: w719 -> [w833]
                    tunnel: w718 -> [w826]
                    tunnel: w717 -> [w825]
                    frame #0 {
                      n441 = local read "ActiveArea_um2"() -> (w748:dbl)
                      n442 = local read "Output Power (mW)"() -> (w746:dbl)
                      n443 = Divide(x=w748, y=100000000.0) -> (x/y=w743:dbl)
                      n444 = local read "Prober GPIB"() -> (w765:string)
                      n445 = Multiply(x=w746, y=0.001) -> (x*y=w744:dbl)
                      n446 = local read "current y"() -> (w761:i32)
                      n447 = local read "current x"() -> (w762:i32)
                      n448 = local read "Laser Current (mA)"() -> (w752:dbl)
                      n449 = local read "Parameters Flash 2"() -> (w755:T2)
                      n450 = local read "Fine Cell Clusters"() -> (w769:T3)
                      n451 = Divide(x=w744, y=w743) -> (x/y=w742:dbl)
                      n452 = call "EG2001 Move Z Down.vi"("GPIB Address"=w765) -> ("Error Out"=w763:errorcluster, "GPIB Address Out"=w764:string)  [unwired: 9 in]
                      n453 = local read "Output Power (mW)"() -> (w749:dbl)
                      n454 = local read "Laser Current (mA)"() -> (w750:dbl)
                      n455 = Index Array(array=w769, index=w756) -> (element=w753:T19)
                      n456 = Unbundle By Name(w753) -> ("Cell Name"=w768:string, "X-coord"=w758:dbl, "Y-coord"=w757:dbl, "Area"=w767:dbl, "Mesa Area"=w766:dbl)
                      n457 = call "get Area.vi"("Laser"=w752, "Cell Data Cluster"=w753) -> ("Area"=w754:dbl)  [unwired: 9 in]
                      n458 = Bundle By Name(cluster=w755, "Cell Area (cm²)"=w754, "Input Current (mA)"=w750, "Power Density (W/cm^2)"=w742, "Incident Power"=w749) -> (w751:T2)
                      n459 = local write "Device Name"(w768) -> ()
                      n460 = local write "ActiveArea_um2"(w767) -> ()
                      n461 = local write "MesaArea_um2"(w766) -> ()
                      n462 = Subtract(x=w757, y=w761) -> (x-y=w759:dbl)
                      n463 = Subtract(x=w758, y=w762) -> (x-y=w760:dbl)
                      n464 = local write "Parameters Flash"(w751) -> ()
                    }
                    frame #1 {
                      n465 = local write "current x"(w774) -> ()
                      n466 = local write "current y"(w773) -> ()
                      n467 = call "EG2001 Move Machine Step X-Y.vi"("Y"=w775, "Steps/Microns"=enum32{"Steps", "Microns"}."Microns", "X"=w776, "error in (no error)"=w778, "GPIB Address"=w779) -> ("Error Out"=w771:errorcluster, "GPIB Address Out"=w772:string)  [unwired: 5 in]
                    }
                    frame #2 {
                      n468 = call "EG2001 Move Z Up.vi"("error in (no error)"=w781, "GPIB Address"=w782) -> ()  [unwired: 10 out]
                    }
                    frame #3 {
                      n469 = local read "Channel"() -> (w795:enum32{"Channel A", "Channel B"})
                      n470 = local read "Wafer Info Flash 2"() -> (w785:T1)
                      n471 = local read "sweep delay ms"() -> (w789:dbl)
                      n472 = local read "Sweep Settings"() -> (w797:T8)
                      n473 = local read "Device Name"() -> (w784:string)
                      n474 = local read "I compliance"() -> (w790:dbl)
                      n475 = Bundle By Name(cluster=w785, "Cell Name"=w784) -> (w783:T1)
                      n476 = local read "V start"() -> (w793:dbl)
                      n477 = local read "points"() -> (w792:u16)
                      n478 = local read "V end"() -> (w794:dbl)
                      n479 = local read "NPLC"() -> (w791:dbl)
                      n480 = local write "Wafer Info Flash"(w783) -> ()
                      n481 = Bundle By Name(cluster=w797, "Channel"=w795, "Vstart"=w793, "Vend"=w794, "# of points"=w792, "NPLC"=w791, "I compliance"=w790, "Delay ms"=w789) -> (w796:T8)
                      n482 = local read "SMU"() -> (w798:refnum<visa-resource-name>)
                      n483 = call "K2602 Vsweep.vi"("Settings"=w796, "SMU"=w798) -> ("V"=w787:dbl[], "I"=w788:dbl[])  [unwired: 7 in, 1 out]
                      n484 = local write "I fine"(w788) -> ()
                      n485 = local write "V fine"(w787) -> ()
                    }
                    frame #4 {
                      n486 = local read "V fine"() -> (w805:dbl[])
                      n487 = local read "I fine"() -> (w812:dbl[])
                      n488 = local read "Wafer Name"() -> (w809:string)
                      n489 = local read "IV fine linear"() -> (w819:cluster{dbl[], dbl[]}[])
                      n490 = local read "IV fine log"() -> (w814:cluster{dbl[], dbl[]}[])
                      n491 = local read "Operator"() -> (w808:string)
                      n492 = local read "current y"() -> (w801:i32)
                      n493 = local read "current x"() -> (w802:i32)
                      n494 = Bundle("V fine"=w805, "I fine"=w812) -> (w817:cluster{"V fine":dbl[], "I fine":dbl[]})  [unwired: 1 in]
                      n495 = Absolute Value(x=w812) -> (abs(x)=w813:dbl[])
                      n496 = local read "Device Name"() -> (w807:string)
                      n497 = Replace Array Subset(array=w819, new element=w817, index=w816) -> (w818:cluster{dbl[], dbl[]}[])
                      n498 = Bundle("V fine"=w805, w813) -> (w811:cluster{"V fine":dbl[], dbl[]})  [unwired: 1 in]
                      n499 = To Double Precision Float(number=w802) -> (double precision float=w804:dbl)
                      n500 = To Double Precision Float(number=w801) -> (double precision float=w803:dbl)
                      n501 = Get Date/Time In Seconds() -> (seconds since 1Jan1904=w799:timestamp)
                      n502 = local write "IV fine linear"(w818) -> ()
                      n503 = call "get Flash FileName .vi"("Time"=w799, "Device Name"=w807, "Operator"=w808, "Wafer Name"=w809, "FineTest save path"="FineTest save path") -> ("appended path"=w806:path)  [unwired: 6 in]
                      n504 = Replace Array Subset(array=w814, new element=w811, index=w816) -> (w815:cluster{dbl[], dbl[]}[])
                      n505 = Bundle(w804, w803) -> (w800:cluster{dbl, dbl})  [unwired: 1 in]
                      n506 = local write "IV fine log"(w815) -> ()
                    }
                    frame #5 {
                      n507 = local read "V fine"() -> (w830:dbl[])
                      n508 = local read "I fine"() -> (w831:dbl[])
                      n509 = Get Date/Time String(seconds (now)=w825, want seconds? (F)=TRUE) -> (date string=w824:string, time string=w821:string)  [unwired: 1 in]
                      n510 = local read "Parameters Flash"() -> (w828:T2)
                      n511 = local read "Wafer Info Flash"() -> (w827:T1)
                      n512 = Build Array(w831, w830) -> (w829:dbl[][])
                      n513 = call <vilib>:"Space Constant.vi"() -> ("String"=w820:string)
                      n514 = Concatenate Strings(w824, w820, w821) -> (w822:string)
                      n515 = local read "Mask"() -> (w832:string)
                      n516 = call "WriteFlashFile.vi"("file path (dialog if empty)"=w833, "Mask Name"=w832, "IV array"=w829, "Date/Time String"=w822, "Parameters"=w828, "Coords"=w826, "Wafer Info"=w827) -> ()  [unwired: 8 in, 1 out]
                    }
                  }
                  n517 = Increment(x=w741) -> (x+1=w720:i32)
                  n518 = local write "Current Device"(w720) -> ()
                  n519 = Divide(x=w720, y=w740) -> (x/y=w739:dbl)
                  n520 = Number To Decimal String(number=w720) -> (decimal integer string=w726:string)  [unwired: 1 in]
                  n521 = Concatenate Strings("IV test for die number: " ("string"), w726) -> (w725:string)
                  n522 = Multiply(x=100.0, y=w739) -> (x*y=w737:dbl)
                  n523 = local write "Status"(w725) -> ()
                  n524 = To Unsigned Byte Integer(number=w737) -> (unsigned 8bit integer=w736:u8)
                  n525 = local write "Progress 2"(w736) -> ()
                }
              }
              frame #2 {
                w838 = -1 ("x")
                n526 = local read "Prober GPIB"() -> (w842:string)
                n527 = local read "current y"() -> (w839:i32)
                n528 = local read "current x"() -> (w840:i32)
                n529 = Multiply(x=w839, y=w838) -> (x*y=w836:i32)
                n530 = Multiply(x=w838, y=w840) -> (x*y=w837:i32)
                n531 = call "EG2001 Move Z Down.vi"("GPIB Address"=w842) -> ("Error Out"=w841:errorcluster, "GPIB Address Out"=w843:string)  [unwired: 9 in]
                n532 = call "EG2001 Move Machine Step X-Y.vi"("Flip X Coordinates?"=FALSE, "Y"=w836, "Steps/Microns"=enum32{"Steps", "Microns"}."Microns", "X"=w837, "error in (no error)"=w841, "GPIB Address"=w843) -> ()  [unwired: 4 in, 2 out]
              }
              frame #3 {
                w844 = 0 ("current x")
                n533 = local write "current x"(w844) -> ()
                n534 = local write "current y"(w844) -> ()
              }
            }
            n535 = Enqueue Element At Opposite End(queue=w693, element="idle", error in (no error)=w692) -> (queue out=w695:refnum<queue>, error out=w694:errorcluster)  [unwired: 1 in, 1 out]
          }
          frame "Update Laser" {
            n536 = local read "TL4000 In"() -> (w854:refnum<visa-resource-name>)
            n537 = local read "Laser Current (mA)"() -> (w851:dbl)
            n538 = call <instrlib>:"TL4000 Initialize.vi"("Reset Device (Reset Device)"=FALSE, "resource name"="TL4000 In") -> ("instrument handle out"=→"TL4000 Out":refnum<visa-resource-name>)  [unwired: 8 in, 1 out]
            n539 = Divide(x=w851, y=1000.0) -> (x/y=w866:dbl)
            n540 = call-poly <vilib>:"Read From Spreadsheet File.vi"("delimiter (\\t)"="," ("delimiter (\\t)"), "file path (dialog if empty)"="Load Calibration File") -> ("all rows"=w861:dbl[][])  [unwired: 5 in, 4 out]
            n541 = call <instrlib>:"TL4000 Set Laser Diode Current Setpoint.vi"("Laser Diode Current Setpoint (0.0)"=w866, "instrument handle"=w854) -> ()  [unwired: 8 in, 2 out]
            n542 = Index Array(array=w861, index (row)=0) -> (element=w863:dbl[])  [unwired: 1 in]
            n543 = Index Array(array=w861, index (row)=1) -> (element=w853:dbl[])  [unwired: 1 in]
            n544 = Array Size(array=w853) -> (size(s)=w852:i32)
            n545 = call "Convert to Dynamic Data"("Array"=w863) -> ("Dynamic Data Type"=w864:dynamicdata)  [unwired: 3 in]
            n546 = call "Convert to Dynamic Data2"("Array"=w853) -> ("Dynamic Data Type"=w865:dynamicdata)  [unwired: 3 in]
            n547 = for {
              N: w852 -> [_]
              tunnel: w863 -> [w871] mode=indexing
              tunnel: w851 -> [w872]
              tunnel: w853 -> [w870]
              tunnel: [w868] -> w858
              i -> [w869]
              stop <- w867 stop-if-true
              n548 = Equal?(x=w871, y=w872) -> (x = y?=w867:bool)
              n549 = case shown="False" w867 {
                tunnel: w870 -> [_ w875]
                tunnel: w869 -> [_ w874]
                tunnel: [_ w873] -> w868
                frame False {
                }
                frame True {
                  n550 = Index Array(array=w875, index=w874) -> (element=w873:dbl)
                }
              }
            }
            "Output Power (mW)" <- w858
            n551 = call "Build XY Graph"("Y Input"=w865, "X Input"=w864) -> ("XY Graph"=→"Calibration":cluster{"Y":dbl[], "Y":dbl[]}[])  [unwired: 3 in, 6 out]
          }
          frame "Zero Laser" {
            n552 = local write "Laser Current (mA)"(0.0) -> ()
          }
          frame "raw mask updated" {
            n553 = Enqueue Element At Opposite End(queue=w887, element="idle", error in (no error)=w886) -> (queue out=w889:refnum<queue>, error out=w888:errorcluster)  [unwired: 1 in, 1 out]
            n554 = Two Button Dialog(message="Wold you like to update the Manual mask?", 1:"No" ("F button name (\"Cancel\")"), 2:"Yes" ("T button name (\"OK\")")) -> (T button?=w880:bool)
            n555 = case shown="True" w880 {
              frame False {
              }
              frame True {
                n556 = local read "Mask File Raw"() -> (w890:path)
                n557 = local write "Mask File Manual"(w890) -> ()
              }
            }
          }
          frame "mask manual update" {
            n558 = Enqueue Element At Opposite End(queue=w898, element="idle", error in (no error)=w897) -> (queue out=w900:refnum<queue>, error out=w899:errorcluster)  [unwired: 1 in, 1 out]
            n559 = Two Button Dialog(message="Would you like update mask file for raw test?", 1:"No" ("F button name (\"Cancel\")"), 2:"Yes" ("T button name (\"OK\")")) -> (T button?=w891:bool)
            n560 = case shown="True" w891 {
              frame False {
              }
              frame True {
                n561 = local read "Mask File Manual"() -> (w901:path)
                n562 = local write "Mask File Raw"(w901) -> ()
              }
            }
          }
          frame "refresh device names" {
            n563 = Enqueue Element At Opposite End(queue=w907, element="idle", error in (no error)=w906) -> (queue out=w909:refnum<queue>, error out=w908:errorcluster)  [unwired: 1 in, 1 out]
            n564 = call "getDB unique Device.vi"("Mask"="Mask Name") -> ("NameList"=w902:string[])  [unwired: 9 in, 1 out]
            "NameList" <- w902
            n565 = property on="Available Device Name" class="CmbBox"("Strings[]"=w902) -> ()  [unwired: 2 in, 2 out]
          }
          frame "add to list" {
            n566 = property on="Test List" class="LstBox (strict)"() -> ("Item Names"=w912:string[])  [unwired: 2 in, 2 out]
            n567 = Enqueue Element At Opposite End(queue=w916, element="idle", error in (no error)=w914) -> (queue out=w918:refnum<queue>, error out=w917:errorcluster)  [unwired: 1 in, 1 out]
            n568 = local read "Available Device Name"() -> (w911:string)
            n569 = Build Array (concatenate)(w912, w911) -> (w910:string[])
            n570 = property on="Test List" class="LstBox (strict)"("Item Names"=w910) -> ()  [unwired: 2 in, 2 out]
          }
          frame "add to laser list" {
            n571 = property on="Laser List" class="LstBox (strict)"() -> ("Item Names"=w923:string[])  [unwired: 2 in, 2 out]
            n572 = local read "Desired Current (mA)"() -> (w920:dbl)
            n573 = Format Into String(format string="%08.4f", w920) -> (resulting string=w919:string)  [unwired: 2 in, 1 out]
            n574 = Build Array (concatenate)(w923, w919) -> (w922:string[])
            n575 = property on="Laser List" class="LstBox (strict)"("Item Names"=w922) -> ()  [unwired: 2 in, 2 out]
          }
          frame "remove from laser list" {
            n576 = local read "Laser List"() -> (w932:i32)
            n577 = property on="Laser List" class="LstBox (strict)"() -> ("Item Names"=w931:string[])  [unwired: 2 in, 2 out]
            n578 = Delete From Array(array=w931, index=w932) -> (array with subset deleted=w930:string[])  [unwired: 1 in, 1 out]
            n579 = property on="Laser List" class="LstBox (strict)"("Item Names"=w930) -> ()  [unwired: 2 in, 2 out]
          }
          frame "clear laser list" {
            n580 = property on="Laser List" class="LstBox (strict)"("Item Names"=string[] []) -> ()  [unwired: 2 in, 2 out]
          }
          frame "remove from list" {
            n581 = property on="Test List" class="LstBox (strict)"() -> ("Item Names"=w939:string[])  [unwired: 2 in, 2 out]
            n582 = local read "Test List"() -> (w937:i32)
            n583 = Enqueue Element At Opposite End(queue=w941, element="idle", error in (no error)=w940) -> (queue out=w943:refnum<queue>, error out=w942:errorcluster)  [unwired: 1 in, 1 out]
            n584 = Delete From Array(array=w939, index=w937) -> (array with subset deleted=w938:string[])  [unwired: 1 in, 1 out]
            n585 = property on="Test List" class="LstBox (strict)"("Item Names"=w938) -> ()  [unwired: 2 in, 2 out]
          }
          frame "clear list" {
            n586 = property on="Test List" class="LstBox (strict)"("Item Names"=string[] []) -> ()  [unwired: 2 in, 2 out]
            n587 = Enqueue Element(queue=w950, element="idle", error in (no error)=w948) -> (queue out=w952:refnum<queue>, error out=w951:errorcluster)  [unwired: 1 in, 1 out]
          }
          frame "pick device" {
            n588 = flat-sequence {
              frame #0 {
                n589 = local read "Mask File all"() -> (w961:path)
                n590 = property on="Test List" class="LstBox (strict)"() -> ("Item Names"=w963:string[])  [unwired: 2 in, 2 out]
                n591 = local read "Counter"() -> (w962:i32)
                n592 = Index Array(array=w963, index=w962) -> (element=w959:string)
                n593 = local write "Device Name"(w959) -> ()
                n594 = call "Mask file select device.vi"("Device"=w959, "MaskFile"=w961) -> ("RawMask"=w960:path)  [unwired: 9 in]
                n595 = local write "Mask File Raw"(w960) -> ()
              }
              frame #1 {
                n596 = local read "Counter"() -> (w965:i32)
                n597 = Increment(x=w965) -> (x+1=w964:i32)
                n598 = local write "Counter"(w964) -> ()
              }
              frame #2 {
                n599 = property on="Test List" class="LstBox (strict)"() -> ("Item Names"=w968:string[])  [unwired: 2 in, 2 out]
                n600 = local read "Counter"() -> (w969:i32)
                n601 = Array Size(array=w968) -> (size(s)=w967:i32)
                n602 = Equal?(x=w969, y=w967) -> (x = y?=w966:bool)
                n603 = case shown="False" w966 {
                  frame False {
                  }
                  frame True {
                    n604 = local write "Counter"(0 ("Counter")) -> ()
                  }
                }
              }
            }
            n605 = Enqueue Element(queue=w958, element="idle", error in (no error)=w956) -> (queue out=w957:refnum<queue>, error out=w955:errorcluster)  [unwired: 1 in, 1 out]
          }
          frame "pick laser" {
            n606 = flat-sequence {
              frame #0 {
                n607 = property on="Laser List" class="LstBox (strict)"() -> ("Item Names"=w976:string[])  [unwired: 2 in, 2 out]
                n608 = local read "Laser Counter"() -> (w977:i32)
                n609 = Index Array(array=w976, index=w977) -> (element=w975:string)
                n610 = Fract/Exp String To Number(string=w975) -> (number=w974:dbl)  [unwired: 3 in, 1 out]
                n611 = local write "Laser Current (mA)"(w974) -> ()
              }
              frame #1 {
                n612 = local read "Laser Counter"() -> (w979:i32)
                n613 = Increment(x=w979) -> (x+1=w978:i32)
                n614 = local write "Laser Counter"(w978) -> ()
              }
              frame #2 {
                n615 = property on="Laser List" class="LstBox (strict)"() -> ("Item Names"=w980:string[])  [unwired: 2 in, 2 out]
                n616 = local read "Laser Counter"() -> (w983:i32)
                n617 = Array Size(array=w980) -> (size(s)=w982:i32)
                n618 = Equal?(x=w983, y=w982) -> (x = y?=w981:bool)
                n619 = case shown="True" w981 {
                  frame False {
                  }
                  frame True {
                    n620 = local write "Laser Counter"(0 ("Counter")) -> ()
                  }
                }
              }
            }
          }
        }
      }
      n621 = Release Queue(queue=w19, force destroy? (F)=TRUE, error in (no error)=w10) -> (error out=→"error out":errorcluster)  [unwired: 2 out]
    }
  }
